vi "MC_7_24_12c_JW.vi"() -> ()   [LabVIEW 2011]
uses:
  <vilib>/Utility/file.llb/Read From Spreadsheet File (string).vi
  <vilib>/Utility/inputDevices.llb/keyboardAcquire.vi
  <vilib>/Utility/file.llb/Write To Spreadsheet File (DBL).vi
  <vilib>/Utility/file.llb/Write To Spreadsheet File (string).vi
  <vilib>/regexp/Match Regular Expression.xnode
panel:
  in  "Room Temp":dbl
  out "No Image 2":path=path "\\\\acad1\\physics/Jurchescu-group/JW-PD/Image Not Found.png"
  out "Save1 Array":string[][](array[string])
  out "XY Graph-Lin":cluster{dbl[], dbl[]}[](graph)
  out "Lin Vd":dbl
  out "Lin-Vg Array-Used":dbl[](array[numeric])
  out "Lin Id-Used":dbl[](array[numeric])
  out "Comments":string
  out "Folder Index":dbl caption="Length"
  out "Current \nRecord":string[](array[string])
  out "Transformer \nHeaders":string[](array[string])
  out "Current Device ID":string
  out "Column":string
  out "Row":string
  out "Rec: Concentration":dbl
  out "Rec: Solvent":string
  out "Rec: Method":string
  in  "?":T1(tab)
  out "Rec: Material":string
  in  "Treatment Concentration (mM):":dbl=30.0
  in  "Surface Treatment:":string
  in  "# Drops*:":dbl=inf
  in  "Solution Temp (C):":dbl=55.0
  in  "Relative Humidity (%):":dbl=nan
  in  "Room Temp (F):":dbl=nan
  in  "Time (s):":dbl=80.0
  out "Accel (RPM/s):":dbl
  in  "RPM:":dbl=1000.0
  in  "Wait Time (s):":dbl=10.0
  in  "Sample #:":dbl=1.0
  in  "Fabricator:":string="Jeremy"
  in  "Data File":path
  out "Data Folder":path
  in  "Image Folder":path
  out "Image File":path=path "D:/UserData/Desktop/Jeremy/WFU/Research/Programs/VI mods/Image Not Found.png"
  in  "Ramp (s):":dbl=3.0
  out "Calc: Off I-Sat":dbl caption="Off I-Sat" format="%#_4e"
  in  "Manuel-Dielectric":bool
  in  "Manuel-Length":bool
  out "Calc: VT-Lin":dbl
  out "New: VT-Lin":dbl
  out "Rec: VT-Lin":dbl caption="VT-Lin" format="%#_3g"
  out "Calc: Trap Density-STS":dbl format="%#_3e"
  out "New: Trap Density-STS":dbl format="%#_3e"
  out "Rec: Trap Density-STS":dbl caption="N-Sat (STS)" format="%#_3e"
  out "Calc: Trap Density-VT":dbl format="%#_3e"
  out "New: Trap Density-VT":dbl format="%#_3e"
  out "Rec: Trap Density-VT":dbl caption="N-Sat (VT)" format="%#_3e"
  out "Calc: Mobility-Lin":dbl format="%#_4e"
  out "New: Mobility-Lin":dbl format="%#_4e"
  out "Rec: Mobility-Lin":dbl caption="Mobility-Lin" format="%#_4e"
  out "Calc: Mobility-Sat":dbl format="%#_4e"
  out "Rec: Length":dbl caption="Length" format="%#_3g"
  out "Rec: Width":dbl caption="Width" format="%#_4g"
  out "Rec: Dielectric (d)":dbl caption="Dielectric (d)" format="%#_3g"
  out "XY Graph":cluster{dbl[], dbl[]}[](graph)
  in  "NumPts":dbl=5.0
  in  "Cancel Button":bool
  in  "Next Button":bool
  in  "Previous Button":bool
  in  "Up Button":bool
  in  "Down Button":bool
  out "Data Name:":string
  in  "Save Changes?":bool
  in  "New: Dielectric":dbl
  in  "New: Length":dbl
  in  "New: Width":dbl
  out "New: Mobility-Sat":dbl format="%#_4e"
  in  "Slide":dbl(slide) step=1.0 scale=-14.3..89.0 scale format="%#_1p"
  in  "Blank Button":bool
  in  "Zoom":i16(slide)=-3 scale=-5.0..5.0
  out "Image Out 2":T2(plugin-control)
  out "Image Out":T2(plugin-control)
  in  "Magnification":u16(ring) items=["5x", "10x", "20x", "50x", "80x"]
  out "Total Width":dbl
  out "Distances":dbl[](array[numeric])
  in  "Undo Button":bool
  in  "Remove Button":bool
  out "Rec: Mobility-Sat":dbl caption="Mobility-Sat" format="%#_4e"
  out "Index":string
  out "Image Name":string
  in  "Export":bool
  out "Calc: VT-Sat":dbl format="%#_3g"
  out "New: VT-Sat":dbl format="%#_3g"
  in  "Manual-Width":bool caption="Manual"
  out "XY Graph 2":cluster{dbl[], dbl[]}[](graph)
  in  "Next Button 2":bool
  in  "Previous Button 2":bool
  in  "Slide 2":dbl(slide) step=1.0 scale=-1.0..82.0 scale format="%#_1p"
  out "Calc: STS":dbl format="%#_3g"
  out "New: STS":dbl format="%#_3g"
  in  "NumPts 2":dbl=5.0 caption="NumPts"
  out "Rec: VT-Sat":dbl caption="VT-Sat" format="%#_3g"
  out "Rec: STS":dbl caption="STS-Sat" format="%#_3g"
  out "Rec: On/Off":dbl caption="On/Off-Sat" format="%#_4e"
  in  "Save Changes? 2":bool
  in  "Save Changes? 3":bool
  out "Date Recorded":string="Date Recorded" caption="Measured"
  out "Date Created":string caption="Fabricated"
  out "Rec: Temp":dbl caption="Sample Temp"
  out "New: Temp":dbl
  out "String":string
  in  "No Image":path=path "\\\\acad1\\physics/Jurchescu-group/JW-PD/Image Not Found.png"
  in  "Project":path=path "\\\\acad1\\physics/Jurchescu-group/JW-PD/Group Library/Origin Project Files/DeviceData_7_25a_JWW.opj"
  out "Index 2":dbl
  out "Sat Id-Log-Used":dbl[](array[numeric])
  out "Vg Array-Log-Used":dbl[](array[numeric])
  out "ROI Descriptor out":T3 {"Contours"."Type" items=["No Selection", "Point", "Line", "Rectangle", "Oval", "Polygon", "Freehand Region", "Annulus", "Unused2", "Unused3", "Broken Line", "Freehand Line", "Rotated Rectangle"]}
  out "ROI Descriptor":T3 {"Contours"."Type" items=["No Selection", "Point", "Line", "Rectangle", "Oval", "Polygon", "Freehand Region", "Annulus", "Unused2", "Unused3", "Broken Line", "Freehand Line", "Rotated Rectangle"]}
  out "Numeric 3":dbl
  out "Array 6":dbl[][](array[numeric])
  out "Cluster":T4
  out "Array 5":dbl[](array[numeric])
  out "Array 4":dbl[](array[numeric])
  out "Array 3":dbl[](array[numeric])
  out "Numeric 2":dbl
  out "Numeric":dbl
  out "Sat Id-Used":dbl[](array[numeric])
  out "Sat Vg Array-Used":dbl[](array[numeric])
  out "MobVi Index":dbl
  in  "Row Start":dbl=20.0
  # "Data Locations"
  # "Data Location"
  # "Image Location"
  # "Sample Properties"
  # "*     Inf = Full coverage\n   NaN = Unknown or Not Applicable"
  # "Recorded"
  # "Calculated"
  # "Re-Calculated"
  # "Manual"
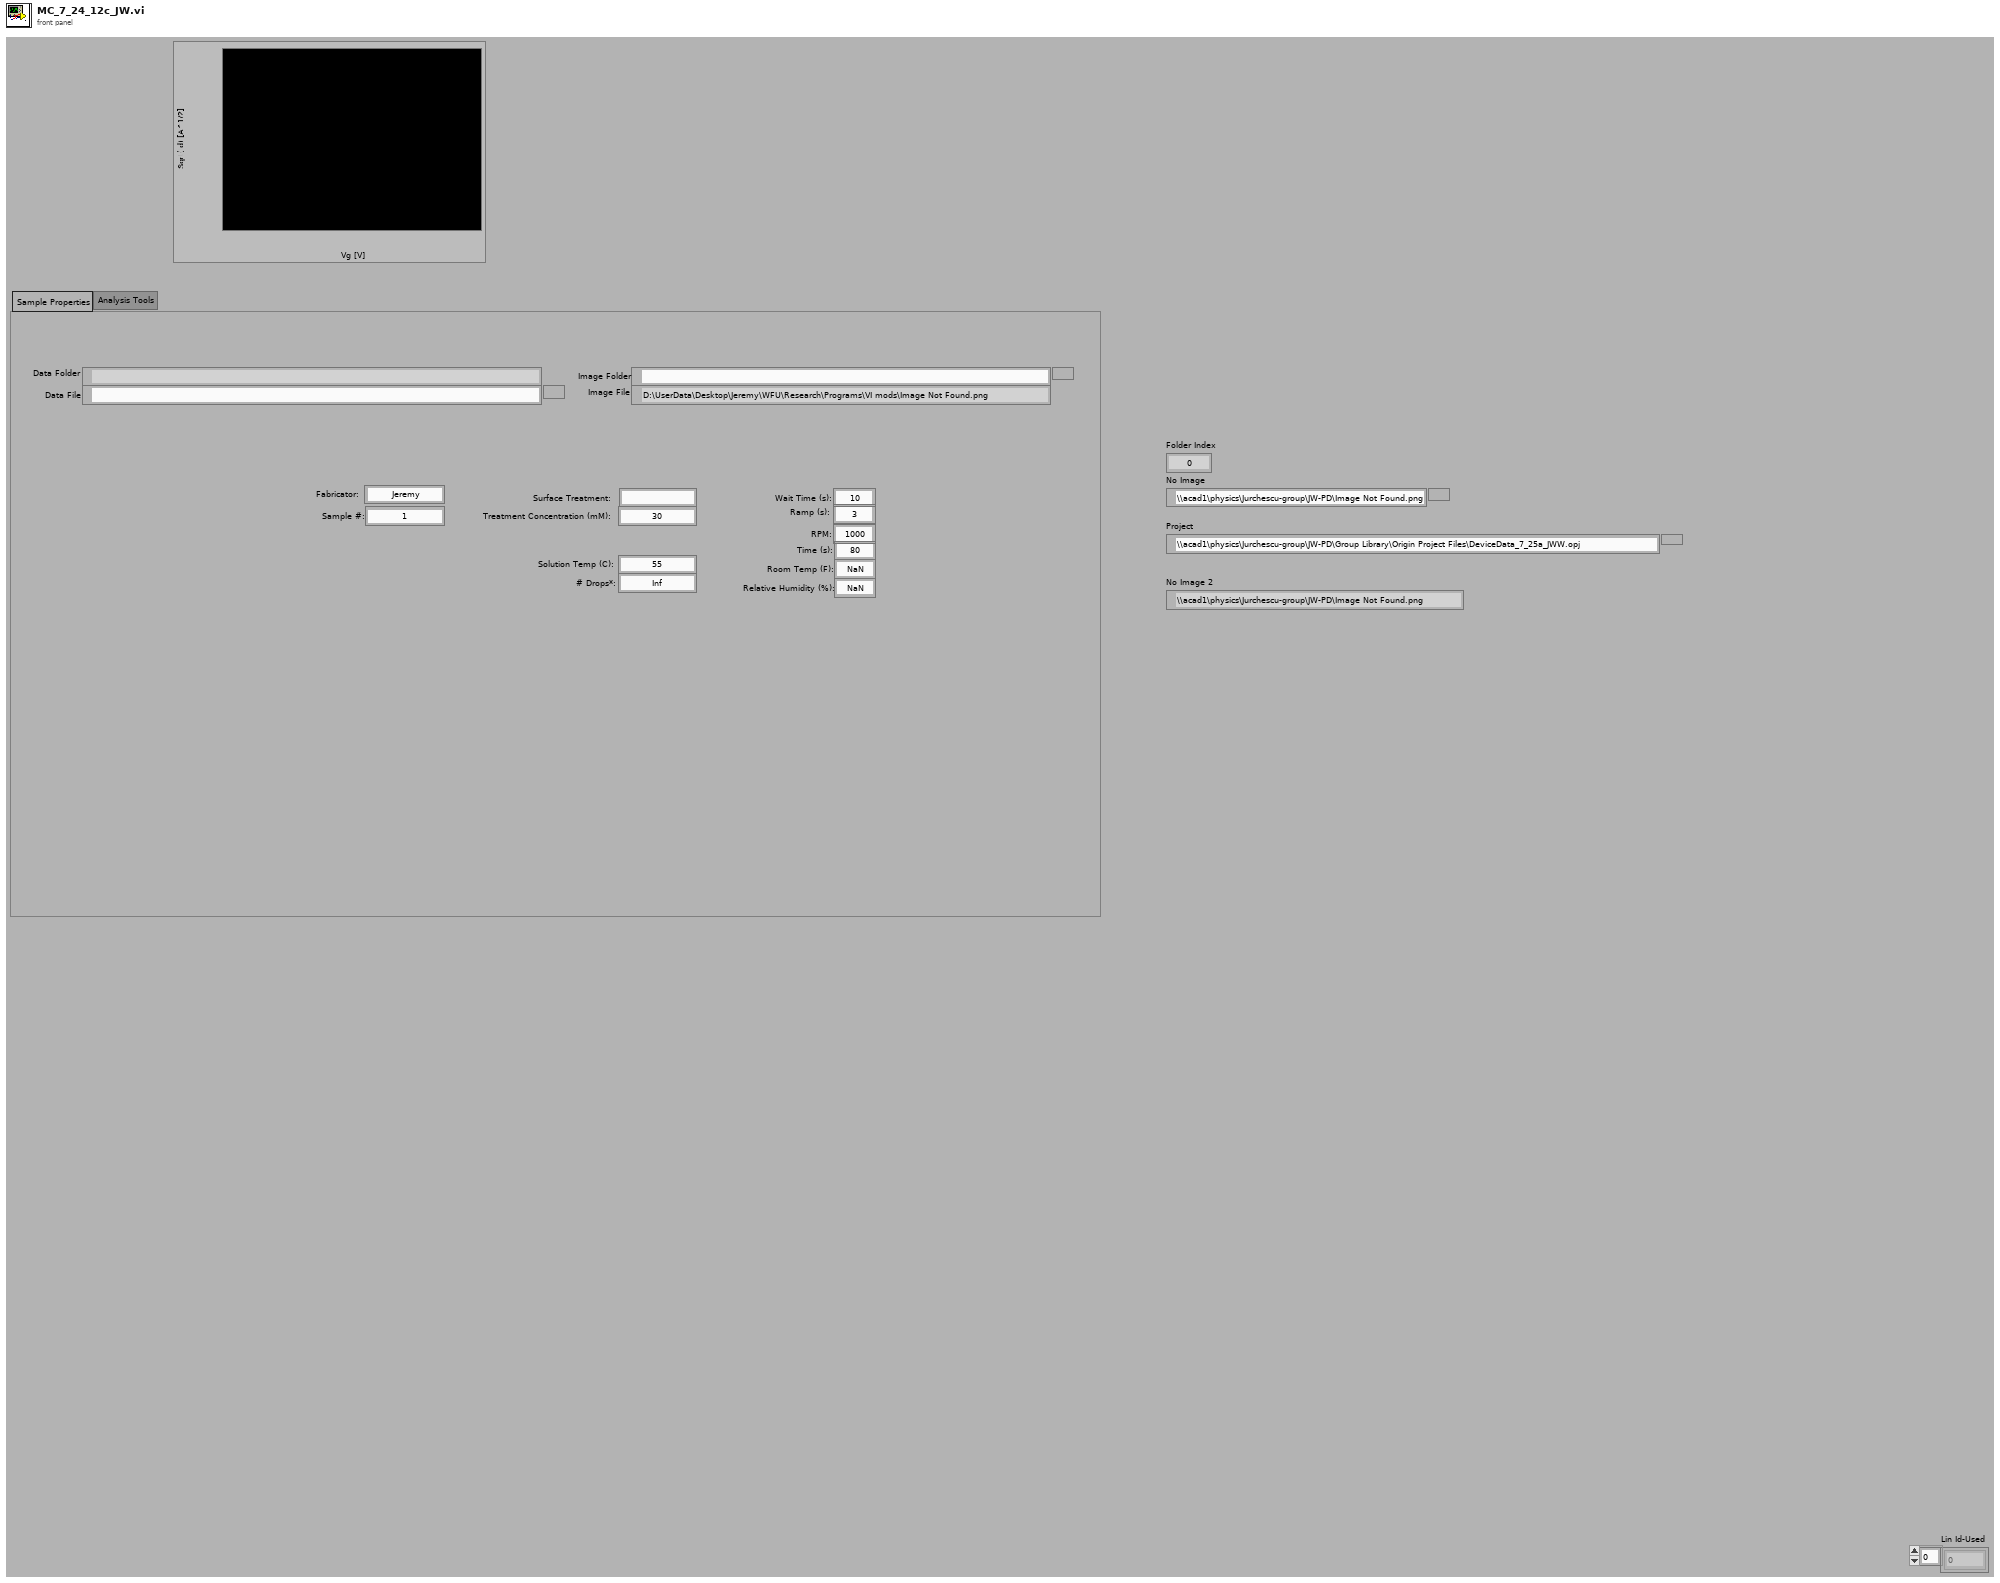
[diagram p1: front panel]
types:
  T1 = enum32{"Sample Properties", "Analysis Tools", "Current Database"}
  T2 = typedef "IMAQ Image.ctl" = refnum<image>
  T3 = typedef "ROI Descriptor" = cluster{"Global Rectangle":i32[], "Contours":cluster{"ID":enum32{"External", "Internal"}, "Type":u32, "Coordinates":i32[]}[]}
  T4 = cluster{"Numeric":dbl, "Numeric 2":dbl, "Numeric 3":dbl, "Numeric 4":dbl}
  T5 = cluster{"Mobility-Sat":dbl, "Moblitity-Lin":dbl, "On/Off":dbl, "Off Current":dbl, "Vt-Sat":dbl, "STS":dbl, "Trap Density-VT":dbl, "Trap Density-STS":dbl}
  T6 = cluster{"Date Recorded":string, "Index":string, "Length":dbl, "Width":dbl, "Sample Temp":dbl}
  T7 = cluster{"Date Created":string, "Material":string, "Solvent":string, "Concentration":dbl, "Method":string, "Dielectric (nm)":dbl, "Treatment":string, "Comments":string}
  T8 = cluster{"Mobility-Sat":dbl, "Vt-Sat":dbl, "Mobility-Lin":dbl, "Vt-Lin":dbl, "Off I-Sat":dbl, "On/Off I-Sat":dbl}
  T9 = cluster{"[0]":cluster{dbl[], dbl[]}, "[1]":cluster{dbl[], dbl[]}, "[2]":cluster{dbl[], dbl[]}, "[3]":cluster{dbl[], dbl[]}, "[4]":cluster{dbl[], dbl[]}, "[5]":cluster{dbl[], dbl[]}, "[6]":cluster{dbl[], dbl[]}, "[7]":cluster{dbl[], dbl[]}, "[8]":cluster{dbl[], dbl[]}}
  T10 = cluster{"Global Rectangle":i32[], "Contours":cluster{"Contour Type":u32, "ROI Type":u32, "Points":i32[]}[]}
  T11 = typedef "LVBoundsTypeDef.ctl" = cluster{"Width":u32, "Height":u32}
  T12 = enum16{"0", "1", "2", "3", "4", "5", "6", "7", "8", "9", "A", "B", "C", "D", "E", "F", "G", "H", "I", "J", "K", "L", "M", "N", "O", "P", "Q", "R", "S", "T", "U", "V", "W", "X", "Y", "Z", "F1", "F2", "F3", "F4", "F5", "F6", "F7", "F8", "F9", "F10", "F11", "F12", "F13", "F14", "F15", "ADD", "BACK", "BACKSLASH", "CAPITAL", "COMMA", "DECIMAL", "DELETE", "DIVIDE", "DOWN", "END", "EQUALS", "ESCAPE", "GRAVE (`)", "HOME", "INSERT", "LBRACKET", "LCONTROL", "LEFT", "L ALT", "LSHIFT", "LWIN", "MINUS", "MULTIPLY", "NEXT", "NUMLOCK", "NUMPAD_0", "NUMPAD_1", "NUMPAD_2", "NUMPAD_3", "NUMPAD_4", "NUMPAD_5", "NUMPAD_6", "NUMPAD_7", "NUMPAD_8", "NUMPAD_9", "PAUSE", "PERIOD", "PRIOR (PG UP)", "RBRACKET", "RCONTROL", "RETURN", "RIGHT", "R ALT", "RSHIFT", "RWIN", "SCROLL", "SEMICOLON", "SLASH", "SPACE", "SUBTRACT", "TAB", "UP", "ENTER (num pad)", "' (quote)"}[]
  T13 = enum16{"0", "1", "2", "3", "4", "5", "6", "7", "8", "9", "A", "B", "C", "D", "E", "F", "G", "H", "I", "J", "K", "L", "M", "N", "O", "P", "Q", "R", "S", "T", "U", "V", "W", "X", "Y", "Z", "F1", "F2", "F3", "F4", "F5", "F6", "F7", "F8", "F9", "F10", "F11", "F12", "F13", "F14", "F15", "ADD", "BACK", "BACKSLASH", "CAPITAL", "COMMA", "DECIMAL", "DELETE", "DIVIDE", "DOWN", "END", "EQUALS", "ESCAPE", "GRAVE (`)", "HOME", "INSERT", "LBRACKET", "LCONTROL", "LEFT", "L ALT", "LSHIFT", "LWIN", "MINUS", "MULTIPLY", "NEXT", "NUMLOCK", "NUMPAD_0", "NUMPAD_1", "NUMPAD_2", "NUMPAD_3", "NUMPAD_4", "NUMPAD_5", "NUMPAD_6", "NUMPAD_7", "NUMPAD_8", "NUMPAD_9", "PAUSE", "PERIOD", "PRIOR (PG UP)", "RBRACKET", "RCONTROL", "RETURN", "RIGHT", "R ALT", "RSHIFT", "RWIN", "SCROLL", "SEMICOLON", "SLASH", "SPACE", "SUBTRACT", "TAB", "UP", "ENTER (num pad)", "' (quote)"}
  T14 = cluster{"Contour Type":u32, "ROI Type":u32, "Points":i32[]}[]
  T15 = cluster{i32[], cluster{"Contour Type":u32, "ROI Type":u32, "Points":i32[]}[]}
  T16 = cluster{string, sgl, bool, bool, bool, bool, bool, bool, i32}
  T17 = cluster{i32, cluster{string, sgl, bool, bool, bool, bool, bool, bool, i32}, i32, i32}
  T18 = cluster{"Contour Type":u32, "ROI Type":u32, "Points":i32[]}
  T19 = cluster{"Points[0]":i32, "Points[1]":i32, "Points[2]":i32, "Points[3]":i32, "Points[4]":i32, "Points[5]":i32, "Points[6]":i32, "Points[7]":i32, "Points[8]":i32}
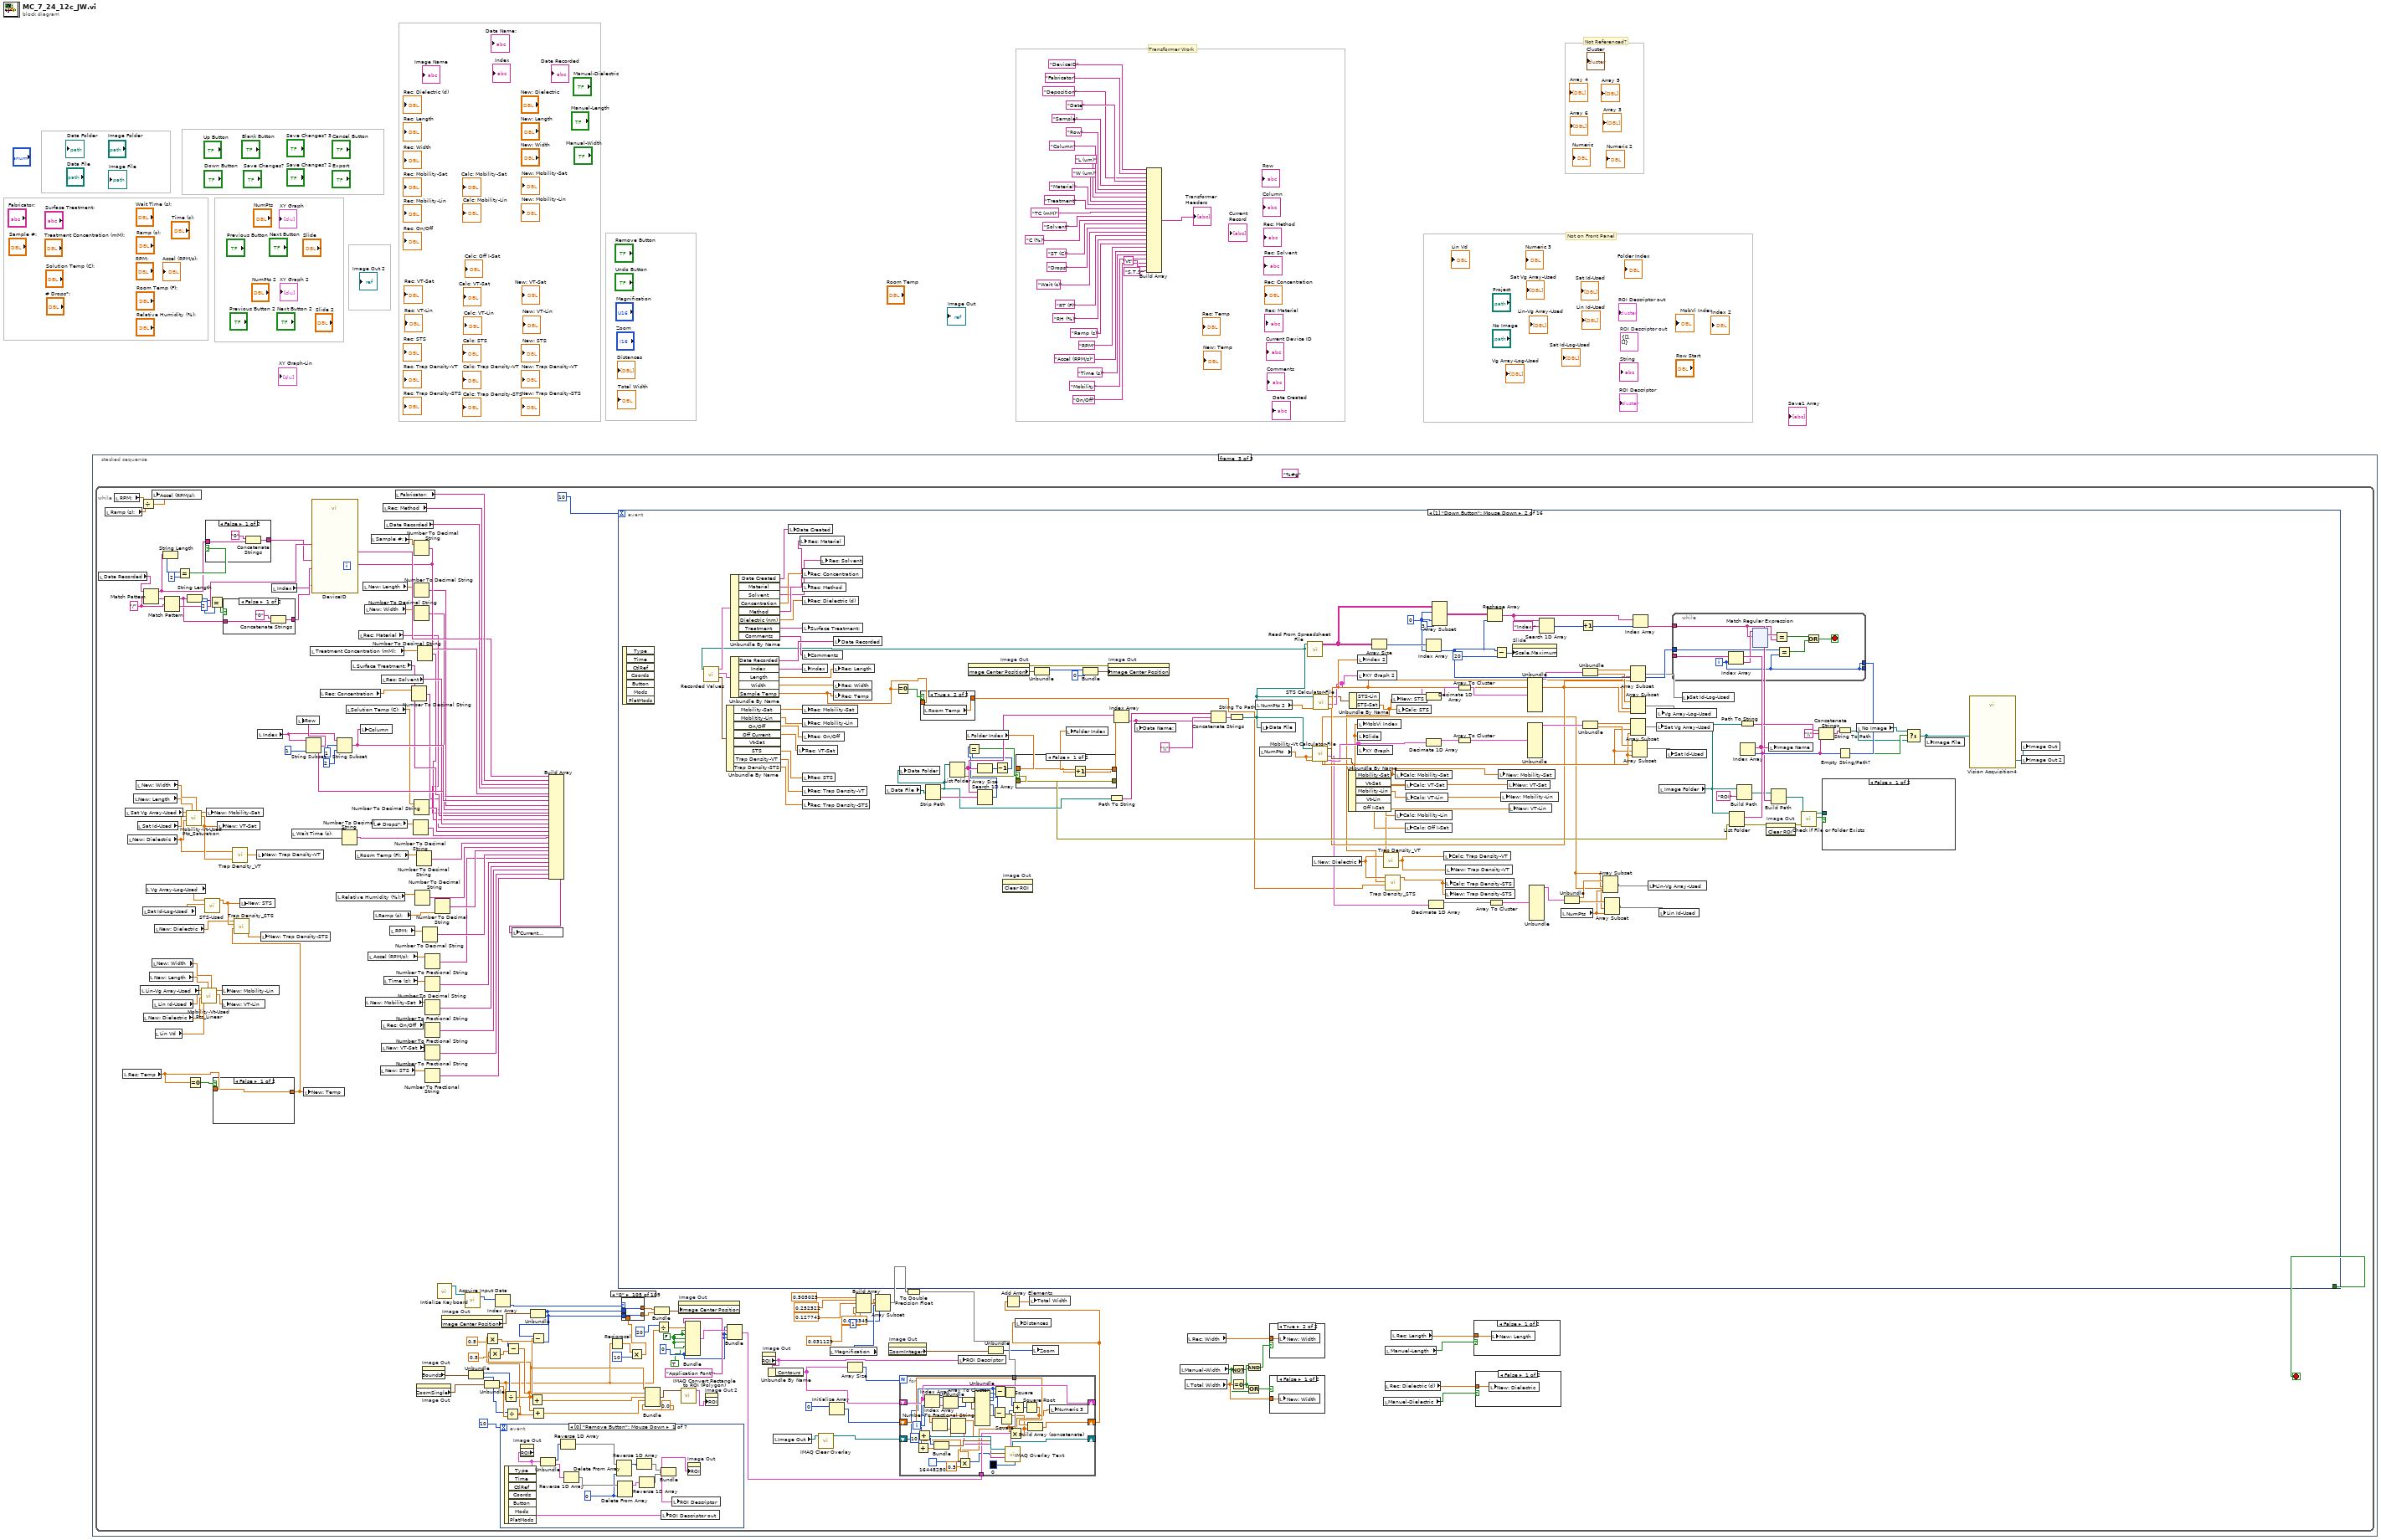
[diagram p0: block diagram]
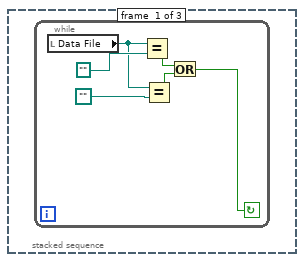
[diagram p2: hidden frame]
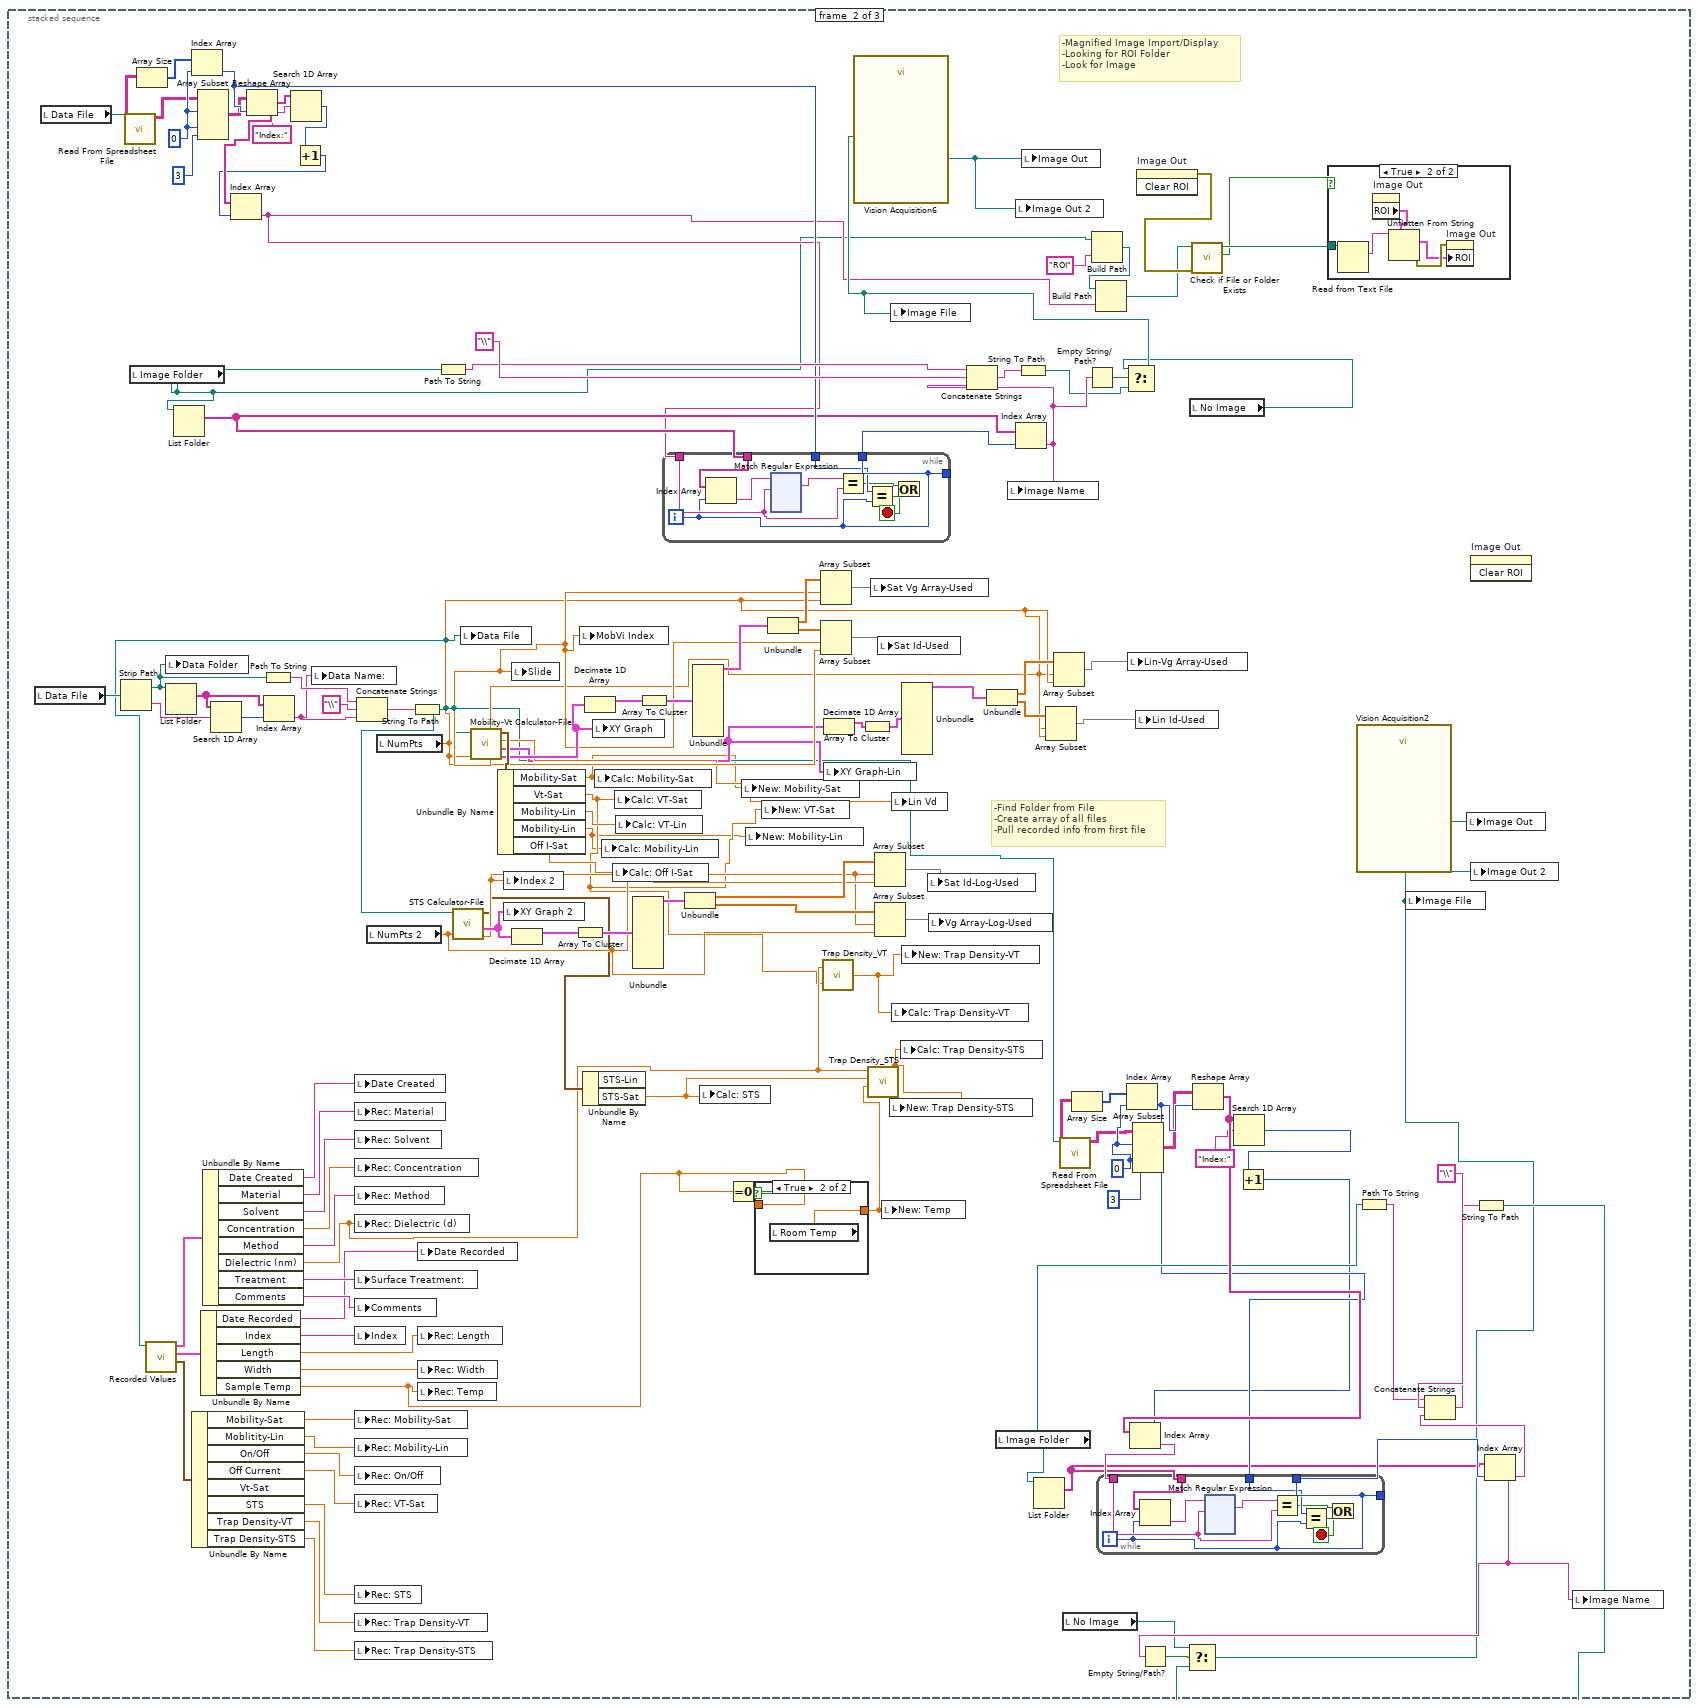
[diagram p3: hidden frame]
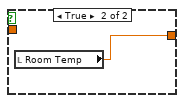
[diagram p6: hidden frame]
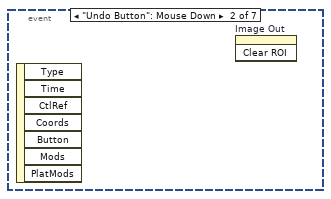
[diagram p13: hidden frame]
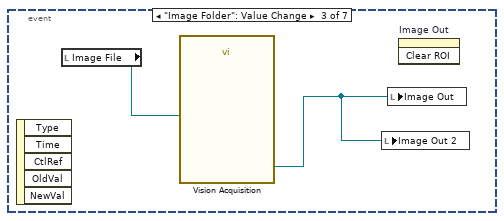
[diagram p14: hidden frame]
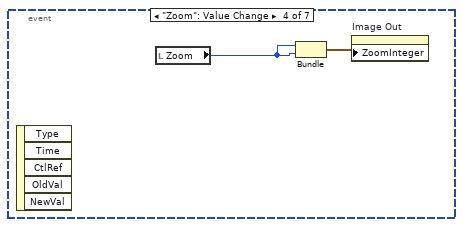
[diagram p15: hidden frame]
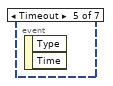
[diagram p16: hidden frame]
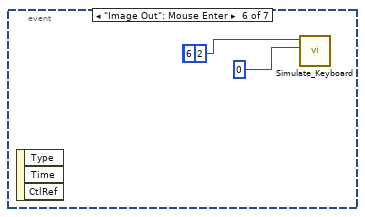
[diagram p17: hidden frame]
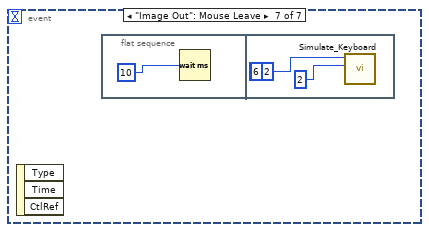
[diagram p18: hidden frame]
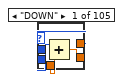
[diagram p19: hidden frame]
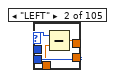
[diagram p20: hidden frame]
diagram:
  (unwired) T3 {"Global Rectangle"=[], "Contours"=[]}  # ROI Descriptor out
  # "Not Referenced?"
  # "Transformer Work"
  # "Not on Front Panel"
  n1 = stacked-sequence {
    frame #0 {
      n2 = while {
        stop <- w29 continue-if-true
        n3 = local read "Data File"() -> (w31:path)
        n4 = Equal?(x=w31, y=path "") -> (x = y?=w33:bool)
        n5 = Equal?(x=w31, y=path "") -> (x = y?=w32:bool)
        n6 = Or(x=w33, y=w32) -> (x .or. y?=w29:bool)
      }
    }
    frame #1 {
      w127 = 0
      w151 = 0
      # "-Find Folder from File\n-Create array of all files\n-Pull recorded info from first file"
      # "-Magnified Image Import/Display\n-Looking for ROI Folder\n-Look for Image"
      n7 = local read "Data File"() -> (w131:path)
      n8 = local read "Data File"() -> (w146:path)
      n9 = Strip Path(path=w131) -> (stripped path=w132:path, name=w118:string)
      n10 = call-poly <vilib>:"Read From Spreadsheet File.vi"("file path (dialog if empty)"=w146) -> ("all rows"=w149:string[][])  [unwired: 6 in, 4 out]
      n11 = local read "Image Folder"() -> (w88:path)
      n12 = Array Size(array=w149) -> (size(s)=w150:i32[])
      n13 = local write "Data Folder"(w132) -> ()
      n14 = List Folder(path=w132) -> (filenames=w122:string[])  [unwired: 3 in, 3 out]
      n15 = List Folder(path=w88) -> (filenames=w155:string[])  [unwired: 3 in, 3 out]
      n16 = Index Array(array=w150, index=w151) -> (element=w157:i32)
      n17 = Array Subset(array=w149, index (row)=w151, index (col)=w151, length (col)=3) -> (w148:string[][])  [unwired: 1 in]
      n18 = Search 1D Array(1D array=w122, element=w118) -> (index of element=w121:i32)  [unwired: 1 in]
      n19 = Reshape Array(w148, w157) -> (w162:string[])
      n20 = Path To String(path=w132) -> (string=w117:string)
      n21 = Index Array(array=w122, index=w121) -> (element=w87:string)
      n22 = Search 1D Array(1D array=w162, element="Index:") -> (index of element=w154:i32)  [unwired: 1 in]
      n23 = Increment(x=w154) -> (x+1=w153:i32)
      n24 = Index Array(array=w162, index=w153) -> (element=w89:string)
      n25 = local write "Data Name:"(w87) -> ()
      n26 = Concatenate Strings(w117, "\\", w87) -> (w119:string)
      n27 = local read "NumPts 2"() -> (w61:dbl)
      n28 = local read "NumPts"() -> (w52:dbl)
      n29 = String To Path(string=w119) -> (path=w44:path)
      n30 = call "Recorded Values.vi"("Path"=w44) -> ("Recorded Char"=w85:T5, "Recorded Prop"=w84:T6, "Fabrication Prop"=w86:T7)  [unwired: 8 in]
      n31 = Unbundle By Name(w85) -> ("Mobility-Sat"=w73:dbl, "Moblitity-Lin"=w72:dbl, "On/Off"=w71:dbl, "Off Current"=w70:dbl, "STS"=w69:dbl, "Trap Density-VT"=w68:dbl, "Trap Density-STS"=w67:dbl)  [unwired: 1 out]
      n32 = Unbundle By Name(w84) -> ("Date Recorded"=w77:string, "Index"=w76:string, "Length"=w75:dbl, "Width"=w74:dbl, "Sample Temp"=w43:dbl)
      n33 = Unbundle By Name(w86) -> ("Date Created"=w66:string, "Material"=w83:string, "Solvent"=w82:string, "Concentration"=w81:dbl, "Method"=w80:string, "Dielectric (nm)"=w39:dbl, "Treatment"=w79:string, "Comments"=w78:string)
      n34 = local write "Date Created"(w66) -> ()
      n35 = local write "Rec: Material"(w83) -> ()
      n36 = local write "Rec: Solvent"(w82) -> ()
      n37 = local write "Rec: Concentration"(w81) -> ()
      n38 = local write "Rec: Method"(w80) -> ()
      n39 = local write "Rec: Dielectric (d)"(w39) -> ()
      n40 = local write "Surface Treatment:"(w79) -> ()
      n41 = local write "Comments"(w78) -> ()
      n42 = local write "Index"(w76) -> ()
      n43 = local write "Rec: Mobility-Sat"(w73) -> ()
      n44 = local write "Rec: Mobility-Lin"(w72) -> ()
      n45 = local write "Rec: On/Off"(w71) -> ()
      n46 = local write "Rec: VT-Sat"(w70) -> ()
      n47 = local write "Rec: STS"(w69) -> ()
      n48 = local write "Rec: Trap Density-VT"(w68) -> ()
      n49 = local write "Rec: Trap Density-STS"(w67) -> ()
      n50 = local write "Date Recorded"(w77) -> ()
      n51 = local write "Rec: Length"(w75) -> ()
      n52 = local write "Rec: Width"(w74) -> ()
      n53 = local write "Rec: Temp"(w43) -> ()
      n54 = Path To String(path=w88) -> (string=w159:string)
      n55 = call "STS Calculator-File.vi"("NumPts"=w61, "Path"=w44) -> ("STS Index-Sat"=w59:dbl, "XY Graph-Sat"=w60:cluster{dbl[], dbl[]}[], "Ouput"=w58:cluster{"STS-Sat":dbl, "STS-Lin":dbl})  [unwired: 5 in, 2 out]
      n56 = local write "Data File"(w44) -> ()
      n57 = call "Mobility-Vt Calculator-File.vi"("NumPts"=w52, "Path"=w44) -> ("XY Graph-Sat"=w63:cluster{dbl[], dbl[]}[], "XY Graph-Lin"=w47:cluster{dbl[], dbl[]}[], "Lin Vd"=w48:dbl, "Output"=w64:T8, "Index-Sat"=w62:dbl, "Index-Lin"=w51:dbl)  [unwired: 4 in]
      n58 = Unbundle By Name(w64) -> ("Mobility-Sat"=w38:dbl, "Vt-Sat"=w37:dbl, "Mobility-Lin"=w65:dbl, "Mobility-Lin"=w36:dbl, "Off I-Sat"=w45:dbl)
      n59 = local write "Index 2"(w59) -> ()
      n60 = local write "XY Graph 2"(w60) -> ()
      n61 = local write "Slide"(w62) -> ()
      n62 = Decimate 1D Array(w60) -> (w109:cluster{dbl[], dbl[]}[])  [unwired: 1 out]
      n63 = Array To Cluster(array=w109) -> (cluster=w111:T9)
      n64 = local write "MobVi Index"(w62) -> ()
      n65 = Unbundle By Name(w58) -> ("STS-Sat"=w42:dbl)  [unwired: 1 out]
      n66 = Decimate 1D Array(w63) -> (w145:cluster{dbl[], dbl[]}[])  [unwired: 1 out]
      n67 = local write "XY Graph"(w63) -> ()
      n68 = local write "Calc: Mobility-Sat"(w38) -> ()
      n69 = local write "Calc: Mobility-Lin"(w36) -> ()
      n70 = local write "Calc: Off I-Sat"(w45) -> ()
      n71 = local write "Calc: VT-Sat"(w37) -> ()
      n72 = local write "Calc: VT-Lin"(w65) -> ()
      n73 = Unbundle(w111) -> ("[0]"=w110:cluster{dbl[], dbl[]})  [unwired: 8 out]
      n74 = Array To Cluster(array=w145) -> (cluster=w143:T9)
      n75 = while {
        tunnel: w155 -> [w297]
        tunnel: w89 -> [w295]
        tunnel: [w294] -> _
        tunnel: [w294] -> w156
        tunnel: w157 -> [w293]
        i -> [w294]
        stop <- w290 stop-if-true
        n76 = Index Array(array=w297, index=w294) -> (element=w298:string)
        n77 = xnode "Match Regular Expression"("input string"=w298, "regular expression"=w295) -> ("whole match"=w296:string)  [unwired: 4 in, 4 out]
        n78 = Equal?(x=w296, y=w295) -> (x = y?=w292:bool)
        n79 = Equal?(x=w293, y=w294) -> (x = y?=w291:bool)
        n80 = Or(x=w292, y=w291) -> (x .or. y?=w290:bool)
      }
      n81 = Unbundle(w110) -> (w107:dbl[], w106:dbl[])
      n82 = Unbundle(w143) -> ("[0]"=w144:cluster{dbl[], dbl[]})  [unwired: 8 out]
      n83 = local write "Calc: STS"(w42) -> ()
      n84 = Equal To 0?(x=w43) -> (x = 0?=w46:bool)
      n85 = local write "New: Mobility-Sat"(w38) -> ()
      n86 = local write "New: Mobility-Lin"(w36) -> ()
      n87 = case shown="True" w46 {
        tunnel: [w163 w164] -> w41
        tunnel: w43 -> [w163 _]
        frame False {
        }
        frame True {
          n88 = local read "Room Temp"() -> (w164:dbl)
        }
      }
      n89 = local write "New: VT-Sat"(w37) -> ()
      n90 = Unbundle(w144) -> (w108:dbl[], w112:dbl[])
      n91 = Array Subset(array=w108, index=w62, length=w52) -> (w115:dbl[])
      n92 = Array Subset(array=w112, index=w62, length=w52) -> (w116:dbl[])
      n93 = call "Trap Density_VT.vi"("VT"=w37, "Dielectric"=w39) -> ("Trap Density-VT"=w35:dbl)
      n94 = Decimate 1D Array(w47) -> (w57:cluster{dbl[], dbl[]}[])  [unwired: 1 out]
      n95 = local write "XY Graph-Lin"(w47) -> ()
      n96 = Array To Cluster(array=w57) -> (cluster=w56:T9)
      n97 = call "Trap Density_STS.vi"("Temp (T) [K]"=w41, "S.T.S. (S)"=w42, "Dielectric"=w39) -> ("Trap Density (N)"=w40:dbl)  [unwired: 8 in]
      n98 = local write "Sat Vg Array-Used"(w115) -> ()
      n99 = Array Subset(array=w107, index=w59, length=w61) -> (w114:dbl[])
      n100 = Array Subset(array=w106, index=w59, length=w61) -> (w113:dbl[])
      n101 = local write "Sat Id-Used"(w116) -> ()
      n102 = local write "New: Temp"(w41) -> ()
      n103 = local write "New: Trap Density-STS"(w40) -> ()
      n104 = local write "Lin Vd"(w48) -> ()
      n105 = local write "Calc: Trap Density-VT"(w35) -> ()
      n106 = local write "Calc: Trap Density-STS"(w40) -> ()
      n107 = Unbundle(w56) -> ("[0]"=w55:cluster{dbl[], dbl[]})  [unwired: 8 out]
      n108 = local write "New: Trap Density-VT"(w35) -> ()
      n109 = local write "Sat Id-Log-Used"(w114) -> ()
      n110 = local write "Vg Array-Log-Used"(w113) -> ()
      n111 = Unbundle(w55) -> (w54:dbl[], w53:dbl[])
      n112 = local read "Image Folder"() -> (w138:path)
      n113 = Index Array(array=w155, index=w156) -> (element=w105:string)
      n114 = Concatenate Strings(w159, "\\", w105) -> (w160:string)
      n115 = local write "Image Name"(w105) -> ()
      n116 = String To Path(string=w160) -> (path=w103:path)
      n117 = List Folder(path=w138) -> (filenames=w134:string[])  [unwired: 3 in, 3 out]
      n118 = Array Subset(array=w53, index=w51, length=w52) -> (w49:dbl[])
      n119 = Array Subset(array=w54, index=w51, length=w52) -> (w50:dbl[])
      n120 = call-poly <vilib>:"Read From Spreadsheet File.vi"("file path (dialog if empty)"=w44) -> ("all rows"=w125:string[][])  [unwired: 6 in, 4 out]
      n121 = local read "No Image"() -> (w97:path)
      n122 = Array Size(array=w125) -> (size(s)=w126:i32[])
      n123 = Empty String/Path?(string/path=w105) -> (empty?=w104:bool)
      n124 = Build Path(base path=w88, name or relative path="ROI") -> (appended path=w91:path)
      n125 = Build Path(base path=w91, name or relative path=w89) -> (appended path=w90:path)
      n126 = Index Array(array=w126, index=w127) -> (element=w137:i32)
      n127 = local write "Lin-Vg Array-Used"(w50) -> ()
      n128 = Array Subset(array=w125, index (row)=w127, index (col)=w127, length (col)=3) -> (w124:string[][])  [unwired: 1 in]
      n129 = local write "Lin Id-Used"(w49) -> ()
      n130 = invoke on="Image Out" class="ImageControl" method="Clear ROI"() -> (error out=w95:errorcluster)  [unwired: 3 in, 2 out]
      n131 = local read "No Image"() -> (w96:path)
      n132 = Select(t=w96, s=w104, f=w103) -> (s? t:f=w102:path)
      n133 = call "Vision Acquisition6"("Image Path"=w102) -> ("Image Out"=w158:T2)  [unwired: 25 in, 1 out]
      n134 = local write "Image File"(w102) -> ()
      n135 = local write "Image Out 2"(w158) -> ()
      n136 = local write "Image Out"(w158) -> ()
      n137 = call <vilib>:"Check if File or Folder Exists.vi"("error in (no error)"=w95, "path"=w90) -> ("file or folder exists?"=w93:bool, "dup path"=w94:path)  [unwired: 7 in, 1 out]
      n138 = Reshape Array(w124, w137) -> (w142:string[])
      n139 = Search 1D Array(1D array=w142, element="Index:") -> (index of element=w130:i32)  [unwired: 1 in]
      n140 = Increment(x=w130) -> (x+1=w129:i32)
      n141 = Index Array(array=w142, index=w129) -> (element=w135:string)
      n142 = while {
        tunnel: w134 -> [w177]
        tunnel: w135 -> [w175]
        tunnel: [w174] -> _
        tunnel: [w174] -> w136
        tunnel: w137 -> [w173]
        i -> [w174]
        stop <- w170 stop-if-true
        n143 = Index Array(array=w177, index=w174) -> (element=w178:string)
        n144 = xnode "Match Regular Expression"("input string"=w178, "regular expression"=w175) -> ("whole match"=w176:string)  [unwired: 4 in, 4 out]
        n145 = Equal?(x=w176, y=w175) -> (x = y?=w172:bool)
        n146 = Equal?(x=w173, y=w174) -> (x = y?=w171:bool)
        n147 = Or(x=w172, y=w171) -> (x .or. y?=w170:bool)
      }
      n148 = case shown="True" w93 {
        tunnel: w94 -> [_ w165]
        frame False {
        }
        frame True {
          n149 = Read from Text File(file (use dialog)=w165) -> (text=w169:string)  [unwired: 3 in, 3 out]
          n150 = property on="Image Out" class="ImageControl"() -> ("ROI"=w166:T10)  [unwired: 2 in, 2 out]
          n151 = Unflatten From String(type=w166, binary string=w169) -> (value=w167:T10, error out=w168:errorcluster)  [unwired: 3 in, 1 out]
          n152 = property on="Image Out" class="ImageControl"(error in=w168, "ROI"=w167) -> ()  [unwired: 1 in, 2 out]
        }
      }
      n153 = Path To String(path=w138) -> (string=w139:string)
      n154 = invoke on="Image Out" class="ImageControl" method="Clear ROI"() -> ()  [unwired: 3 in, 3 out]
      n155 = Index Array(array=w134, index=w136) -> (element=w100:string)
      n156 = Empty String/Path?(string/path=w100) -> (empty?=w101:bool)
      n157 = Concatenate Strings(w139, "\\", w100) -> (w140:string)
      n158 = String To Path(string=w140) -> (path=w99:path)
      n159 = Select(t=w97, s=w101, f=w99) -> (s? t:f=w98:path)
      n160 = call "Vision Acquisition2"("Image Path"=w98) -> ("Image Out"=w133:T2)  [unwired: 25 in, 1 out]
      n161 = local write "Image File"(w98) -> ()
      n162 = local write "Image Out"(w133) -> ()
      n163 = local write "Image Out 2"(w133) -> ()
      n164 = local write "Image Name"(w100) -> ()
    }
    frame #2 {
      (unwired) "%#g"
      n165 = while {
        stop <- w575 stop-if-true
        w471 = "/"
        w525 = FALSE
        w523 = 0
        n166 = local read "Date Recorded"() -> (w474:string)
        n167 = local read "Ramp (s):"() -> (w441:dbl)
        n168 = local read "RPM:"() -> (w442:dbl)
        n169 = local read "Rec: Temp"() -> (w413:dbl)
        n170 = local read "Sat Vg Array-Used"() -> (w430:dbl[])
        n171 = local read "New: Dielectric"() -> (w415:dbl)
        n172 = local read "New: Length"() -> (w431:dbl)
        n173 = local read "New: Width"() -> (w433:dbl)
        n174 = local read "Sat Id-Used"() -> (w429:dbl[])
        n175 = local read "Lin-Vg Array-Used"() -> (w424:dbl[])
        n176 = Divide(x=w442, y=w441) -> (x/y=w440:dbl)
        n177 = local read "Sat Id-Log-Used"() -> (w428:dbl[])
        n178 = local read "New: Dielectric"() -> (w421:dbl)
        n179 = Match Pattern(string=w474, regular expression=w471) -> (before substring=w465:string, after substring=w472:string)  [unwired: 1 in, 2 out]
        n180 = local read "Vg Array-Log-Used"() -> (w427:dbl[])
        n181 = local read "New: Length"() -> (w423:dbl)
        n182 = local write "Accel (RPM/s):"(w440) -> ()
        n183 = local read "New: Width"() -> (w420:dbl)
        n184 = local read "Lin Id-Used"() -> (w425:dbl[])
        n185 = local read "New: Dielectric"() -> (w417:dbl)
        n186 = local read "Lin Vd"() -> (w419:dbl)
        n187 = String Length(string=w465) -> (length=w468:i32)
        n188 = Match Pattern(string=w472, regular expression=w471) -> (before substring=w459:string, after substring=w470:string)  [unwired: 1 in, 2 out]
        n189 = Equal?(x=w468, y=2) -> (x = y?=w466:bool)
        n190 = call "Mobility-Vt-Used Pts_Saturation.vi"("Width"=w433, "Length"=w431, "Dielectric (d)"=w415, "Sat Id Used"=w429, "Vg Used"=w430) -> ("Vt"=w416:dbl, "Mobility"=w432:dbl)  [unwired: 4 in, 1 out]
        n191 = String Length(string=w459) -> (length=w461:i32)
        n192 = Equal To 0?(x=w413) -> (x = 0?=w412:bool)
        n193 = call "Mobility-Vt-Used Pts_Linear.vi"("Width"=w420, "Length"=w423, "Vd"=w419, "Dielectric (d)"=w421, "Sat Id Used"=w425, "Vg Used"=w424) -> ("Vt"=w426:dbl, "Mobility"=w422:dbl)  [unwired: 3 in, 1 out]
        n194 = call "STS-Used.vi"("Id Used"=w428, "Vg-Used"=w427) -> ("STS"=w418:dbl)  [unwired: 9 in]
        n195 = case shown="False" w466 {
          tunnel: w465 -> [w585 w587]
          tunnel: [w584 w587] -> w464
          frame False {
            n196 = Concatenate Strings("0", w585) -> (w584:string)
          }
          frame True {
          }
        }
        n197 = local write "New: Mobility-Sat"(w432) -> ()
        n198 = Equal?(x=w461, y=2) -> (x = y?=w463:bool)
        n199 = case shown="False" w412 {
          tunnel: [w576 w577] -> w410
          tunnel: w413 -> [w576 _]
          frame False {
          }
          frame True {
            n200 = local read "Room Temp"() -> (w577:dbl)
          }
        }
        n201 = local write "New: VT-Sat"(w416) -> ()
        n202 = local write "New: Mobility-Lin"(w422) -> ()
        n203 = local write "New: VT-Lin"(w426) -> ()
        n204 = case shown="False" w463 {
          tunnel: w459 -> [w581 w583]
          tunnel: [w580 w583] -> w460
          frame False {
            n205 = Concatenate Strings("0", w581) -> (w580:string)
          }
          frame True {
          }
        }
        n206 = call "Trap Density_VT.vi"("VT"=w416, "Dielectric"=w415) -> ("Trap Density-VT"=w414:dbl)
        n207 = call "Trap Density_STS.vi"("Temp (T) [K]"=w410, "S.T.S. (S)"=w418, "Dielectric"=w417) -> ("Trap Density (N)"=w411:dbl)  [unwired: 8 in]
        n208 = local write "New: STS"(w418) -> ()
        n209 = local write "New: Trap Density-VT"(w414) -> ()
        n210 = local read "Index"() -> (w444:string)
        n211 = local write "New: Trap Density-STS"(w411) -> ()
        n212 = local read "Index"() -> (w458:string)
        n213 = local read "Wait Time (s):"() -> (w504:dbl)
        n214 = local write "New: Temp"(w410) -> ()
        n215 = String Subset(string=w444, length (rest)=1) -> (substring=w499:string)  [unwired: 1 in]
        n216 = local write "Row"(w499) -> ()
        n217 = local read "Treatment Concentration (mM):"() -> (w452:dbl)
        n218 = local read "Rec: Concentration"() -> (w439:dbl)
        n219 = local read "Relative Humidity (%):"() -> (w449:dbl)
        n220 = String Subset(string=w444, offset (0)=1, length (rest)=2) -> (substring=w500:string)
        n221 = Number To Decimal String(number=w504) -> (decimal integer string=w505:string)  [unwired: 1 in]
        n222 = local read "Solution Temp (C):"() -> (w493:dbl)
        n223 = local read "Surface Treatment:"() -> (w451:string)
        n224 = local read "Room Temp (F):"() -> (w497:dbl)
        n225 = local read "Rec: Material"() -> (w447:string)
        n226 = local write "Column"(w500) -> ()
        n227 = local read "New: Length"() -> (w457:dbl)
        n228 = local read "New: Width"() -> (w456:dbl)
        n229 = local read "New: Mobility-Sat"() -> (w486:dbl)
        n230 = local read "Accel (RPM/s):"() -> (w484:dbl)
        n231 = local read "Sample #:"() -> (w476:dbl)
        n232 = local read "# Drops*:"() -> (w494:dbl)
        n233 = local read "Ramp (s):"() -> (w502:dbl)
        n234 = local read "New: STS"() -> (w478:dbl)
        n235 = local read "Rec: Solvent"() -> (w453:string)
        n236 = local read "New: VT-Sat"() -> (w480:dbl)
        n237 = local read "Rec: On/Off"() -> (w482:dbl)
        n238 = local read "Rec: Method"() -> (w477:string)
        n239 = local read "Time (s):"() -> (w489:dbl)
        n240 = local read "Date Recorded"() -> (w473:string)
        n241 = local read "RPM:"() -> (w490:dbl)
        n242 = local read "Fabricator:"() -> (w498:string)
        n243 = Number To Decimal String(number=w439) -> (decimal integer string=w438:string)  [unwired: 1 in]
        n244 = Number To Decimal String(number=w494) -> (decimal integer string=w495:string)  [unwired: 1 in]
        n245 = Number To Decimal String(number=w476) -> (decimal integer string=w469:string)  [unwired: 1 in]
        n246 = call "DeviceID"("Sample"=w469, "Year"=w470, "Month"=w464, "Day"=w460, "Index"=w458) -> ("Result"=w475:string)  [unwired: 9 in, 1 out]
        n247 = Number To Decimal String(number=w457) -> (decimal integer string=w455:string)  [unwired: 1 in]
        n248 = Number To Decimal String(number=w456) -> (decimal integer string=w454:string)  [unwired: 1 in]
        n249 = Number To Decimal String(number=w493) -> (decimal integer string=w492:string)  [unwired: 1 in]
        n250 = Number To Decimal String(number=w449) -> (decimal integer string=w448:string)  [unwired: 1 in]
        n251 = Number To Decimal String(number=w497) -> (decimal integer string=w496:string)  [unwired: 1 in]
        n252 = property on="Image Out" class="ImageControl"() -> ("ZoomSingle"=w543:cluster{"X":sgl, "Y":sgl})  [unwired: 2 in, 2 out]
        n253 = Number To Decimal String(number=w452) -> (decimal integer string=w450:string)  [unwired: 1 in]
        n254 = property on="Image Out" class="ImageControl"() -> ("Bounds"=w544:T11)  [unwired: 2 in, 2 out]
        n255 = Number To Decimal String(number=w490) -> (decimal integer string=w491:string)  [unwired: 1 in]
        n256 = Number To Fractional String(number=w484) -> (F-format string=w485:string)  [unwired: 3 in]
        n257 = Number To Decimal String(number=w489) -> (decimal integer string=w488:string)  [unwired: 1 in]
        n258 = Number To Fractional String(number=w486) -> (F-format string=w487:string)  [unwired: 3 in]
        n259 = Number To Fractional String(number=w482) -> (F-format string=w483:string)  [unwired: 3 in]
        n260 = Number To Fractional String(number=w480) -> (F-format string=w481:string)  [unwired: 3 in]
        n261 = Number To Fractional String(number=w478) -> (F-format string=w479:string)  [unwired: 3 in]
        n262 = Number To Decimal String(number=w502) -> (decimal integer string=w503:string)  [unwired: 1 in]
        n263 = call <vilib>:"Intialize Keyboard.vi"() -> ("device ID"=w555:refnum<k1>)  [unwired: 10 in, 1 out]
        n264 = property on="Image Out" class="ImageControl"() -> ("Image Center Position"=w550:cluster{"X":u32, "Y":u32})  [unwired: 2 in, 2 out]
        n265 = call-poly <vilib>:"Acquire Input Data.vi"("device ID"=w555) -> ("keys pressed"=w554:T12)  [unwired: 16 in, 2 out]
        n266 = Unbundle(w544) -> ("Width"=w541:u32, "Height"=w540:u32)
        n267 = Unbundle(w543) -> ("X"=w518:sgl, "Y"=w542:sgl)
        n268 = Index Array(array=w554) -> (element=w558:T13)  [unwired: 1 in]
        n269 = event shown="[0] \"Remove Button\": Mouse Down" {
          selector: _ -> [_ _ _ _ _ _ _]
          dyn-events: _ -> [_ _ _ _ _ _ _]
          timeout: 10 -> [_ _ _ _ _ _ _]
          event "Remove Button": Mouse Down {
            w592 = 0
            n270 = event-data() -> ()  [unwired: 1 in, 7 out]
            n271 = property on="Image Out" class="ImageControl"() -> ("ROI"=w590:T10)  [unwired: 2 in, 2 out]
            n272 = Unbundle(w590) -> ("Global Rectangle"=w593:i32[], "Contours"=w595:T14)
            n273 = Reverse 1D Array(array=w593) -> (reversed array=w594:i32[])
            n274 = Reverse 1D Array(array=w595) -> (reversed array=w596:T14)
            n275 = Delete From Array(array=w594, index=w592) -> (array with subset deleted=w597:i32[])  [unwired: 1 in, 1 out]
            n276 = Delete From Array(array=w596, index=w592) -> (array with subset deleted=w598:T14)  [unwired: 1 in, 1 out]
            n277 = Reverse 1D Array(array=w597) -> (reversed array=w599:i32[])
            n278 = Reverse 1D Array(array=w598) -> (reversed array=w600:T14)
            n279 = Bundle(w599, w600) -> (w591:T15)  [unwired: 1 in]
            n280 = local write "ROI Descriptor out"(w590) -> ()
            n281 = local write "ROI Descriptor"(w591) -> ()
            n282 = property on="Image Out" class="ImageControl"("ROI"=w591) -> ()  [unwired: 2 in, 2 out]
          }
          event "Undo Button": Mouse Down {
            n283 = event-data() -> ()  [unwired: 1 in, 7 out]
            n284 = invoke on="Image Out" class="ImageControl" method="Clear ROI"() -> ()  [unwired: 3 in, 3 out]
          }
          event "Image Folder": Value Change {
            n285 = event-data() -> ()  [unwired: 1 in, 5 out]
            n286 = local read "Image File"() -> (w602:path)
            n287 = call "Vision Acquisition"("Image Path"=w602) -> ("Image Out"=w601:T2)  [unwired: 25 in, 1 out]
            n288 = local write "Image Out 2"(w601) -> ()
            n289 = local write "Image Out"(w601) -> ()
            n290 = invoke on="Image Out" class="ImageControl" method="Clear ROI"() -> ()  [unwired: 3 in, 3 out]
          }
          event "Zoom": Value Change {
            n291 = event-data() -> ()  [unwired: 1 in, 5 out]
            n292 = local read "Zoom"() -> (w603:i16)
            n293 = Bundle("Zoom"=w603, "Zoom"=w603) -> (w604:cluster{"Zoom":i16, "Zoom":i16})  [unwired: 1 in]
            n294 = property on="Image Out" class="ImageControl"("ZoomInteger"=w604) -> ()  [unwired: 2 in, 2 out]
          }
          event Timeout {
            n295 = event-data() -> ()  [unwired: 1 in, 2 out]
          }
          event "Image Out": Mouse Enter {
            (unwired) 6
            n296 = event-data() -> ()  [unwired: 1 in, 3 out]
            n297 = call "Simulate_Keyboard.vi"("Action"=0, "Virtual Key"=162) -> ()  [unwired: 7 in, 1 out]
          }
          event "Image Out": Mouse Leave {
            n298 = event-data() -> ()  [unwired: 1 in, 3 out]
            n299 = flat-sequence {
              frame #0 {
                n300 = Wait (ms)(milliseconds to wait=10) -> ()  [unwired: 1 out]
              }
              frame #1 {
                (unwired) 6
                n301 = call "Simulate_Keyboard.vi"("Action"=2, "Virtual Key"=162) -> ()  [unwired: 7 in, 1 out]
              }
            }
          }
        }
        n302 = Divide(x=w541, y=w518) -> (x/y=w531:sgl)
        n303 = Multiply(x=w531, y=0.5) -> (x*y=w537:dbl)
        n304 = Divide(x=w540, y=w542) -> (x/y=w530:sgl)
        n305 = Multiply(x=w530, y=0.5) -> (x*y=w536:dbl)
        n306 = Unbundle(w550) -> ("X"=w532:u32, "Y"=w533:u32)
        n307 = Subtract(x=w533, y=w536) -> (x-y=w534:dbl)
        n308 = Subtract(x=w532, y=w537) -> (x-y=w535:dbl)
        n309 = Add(x=w535, y=w531) -> (x+y=w549:dbl)
        n310 = Add(x=w534, y=w530) -> (x+y=w548:dbl)
        n311 = Build Array(w475, w498, w477, w473, w469, w499, w500, w455, w454, w447, w451, w450, w453, w438, w492, w495, w505, w496, w448, w503, w491, w485, w488, w487, w483, w481, w479) -> (w501:string[])
        n312 = local write "Current \nRecord"(w501) -> ()
        n313 = Reciprocal(x=w518) -> (1/x=w517:sgl)
        n314 = event shown="[1] \"Down Button\": Mouse Down" {
          selector: _ -> [_ _ _ _ _ _ _ _ _ _ _ _ _ _ _ _]
          dyn-events: _ -> [_ _ _ _ _ _ _ _ _ _ _ _ _ _ _ _]
          timeout: 10 -> [_ _ _ _ _ _ _ _ _ _ _ _ _ _ _ _]
          tunnel: [_ _ _ _ _ _ _ _ _ _ _ _ _ TRUE _ TRUE] -> w575
          event Timeout {
            n315 = event-data() -> ()  [unwired: 1 in, 2 out]
          }
          event "Down Button": Mouse Down {
            w942 = 0
            n316 = event-data() -> ()  [unwired: 1 in, 7 out]
            n317 = local read "Data File"() -> (w947:path)
            n318 = Strip Path(path=w947) -> (stripped path=w938:path, name=w956:string)
            n319 = local write "Data Folder"(w938) -> ()
            n320 = List Folder(path=w938) -> (filenames=w952:string[], error out=w892:errorcluster)  [unwired: 3 in, 2 out]
            n321 = local read "Folder Index"() -> (w894:dbl)
            n322 = property on="Image Out" class="ImageControl"() -> (error out=w895:errorcluster, "Image Center Position"=w899:cluster{"X":u32, "Y":u32})  [unwired: 2 in, 1 out]
            n323 = Array Size(array=w952) -> (size(s)=w948:i32)
            n324 = Search 1D Array(1D array=w952, element=w956) -> (index of element=w949:i32)  [unwired: 1 in]
            n325 = Decrement(x=w948) -> (x-1=w950:i32)
            n326 = Equal?(x=w949, y=w950) -> (x = y?=w951:bool)
            n327 = invoke on="Image Out" class="ImageControl" method="Clear ROI"() -> ()  [unwired: 3 in, 3 out]
            n328 = case shown="False" w951 {
              tunnel: w894 -> [w1109 _]
              tunnel: [w1108 0] -> w893
              tunnel: w892 -> [w1107 w1110]
              tunnel: [w1107 w1110] -> w891
              frame False {
                n329 = Increment(x=w1109) -> (x+1=w1108:dbl)
              }
              frame True {
              }
            }
            n330 = Unbundle(w899) -> ("X"=w897:u32)  [unwired: 1 out]
            n331 = local write "Folder Index"(w893) -> ()
            n332 = Bundle("X"=w897, 0) -> (w898:cluster{"X":u32, i32})  [unwired: 1 in]
            n333 = property on="Image Out" class="ImageControl"(error in=w895, "Image Center Position"=w898) -> ()  [unwired: 1 in, 2 out]
            n334 = Path To String(path=w938) -> (string=w957:string)
            n335 = Index Array(array=w952, index=w893) -> (element=w953:string)
            n336 = local write "Data Name:"(w953) -> ()
            n337 = Concatenate Strings(w957, "\\", w953) -> (w955:string)
            n338 = String To Path(string=w955) -> (path=w864:path)
            n339 = call "Recorded Values.vi"("Path"=w864) -> ("Recorded Char"=w959:T5, "Recorded Prop"=w960:T6, "Fabrication Prop"=w958:T7)  [unwired: 8 in]
            n340 = Unbundle By Name(w959) -> ("Mobility-Sat"=w972:dbl, "Moblitity-Lin"=w973:dbl, "On/Off"=w974:dbl, "Off Current"=w975:dbl, "STS"=w976:dbl, "Trap Density-VT"=w977:dbl, "Trap Density-STS"=w978:dbl)  [unwired: 1 out]
            n341 = Unbundle By Name(w958) -> ("Date Created"=w979:string, "Material"=w961:string, "Solvent"=w962:string, "Concentration"=w963:dbl, "Method"=w964:string, "Dielectric (nm)"=w965:dbl, "Treatment"=w966:string, "Comments"=w967:string)
            n342 = Unbundle By Name(w960) -> ("Date Recorded"=w968:string, "Index"=w969:string, "Length"=w970:dbl, "Width"=w971:dbl, "Sample Temp"=w861:dbl)
            n343 = local write "Date Created"(w979) -> ()
            n344 = local write "Rec: VT-Sat"(w975) -> ()
            n345 = local write "Rec: Material"(w961) -> ()
            n346 = local write "Rec: Concentration"(w963) -> ()
            n347 = local write "Rec: Method"(w964) -> ()
            n348 = local write "Rec: Dielectric (d)"(w965) -> ()
            n349 = local write "Surface Treatment:"(w966) -> ()
            n350 = local write "Comments"(w967) -> ()
            n351 = local write "Index"(w969) -> ()
            n352 = local write "Rec: Mobility-Sat"(w972) -> ()
            n353 = local write "Rec: Mobility-Lin"(w973) -> ()
            n354 = local write "Rec: On/Off"(w974) -> ()
            n355 = local write "Rec: STS"(w976) -> ()
            n356 = local write "Rec: Trap Density-VT"(w977) -> ()
            n357 = local write "Rec: Trap Density-STS"(w978) -> ()
            n358 = local write "Rec: Solvent"(w962) -> ()
            n359 = local write "Date Recorded"(w968) -> ()
            n360 = local write "Rec: Length"(w970) -> ()
            n361 = local write "Rec: Width"(w971) -> ()
            n362 = local write "Rec: Temp"(w861) -> ()
            n363 = Equal To 0?(x=w861) -> (x = 0?=w862:bool)
            n364 = case shown="True" w862 {
              tunnel: [w980 w981] -> w860
              tunnel: w861 -> [w980 _]
              frame False {
              }
              frame True {
                n365 = local read "Room Temp"() -> (w981:dbl)
              }
            }
            n366 = local read "NumPts 2"() -> (w886:dbl)
            n367 = local read "NumPts"() -> (w890:dbl)
            n368 = local write "Data File"(w864) -> ()
            n369 = call-poly <vilib>:"Read From Spreadsheet File.vi"("file path (dialog if empty)"=w864) -> ("all rows"=w944:string[][])  [unwired: 6 in, 4 out]
            n370 = call "Mobility-Vt Calculator-File.vi"("NumPts"=w890, "Path"=w864) -> ("XY Graph-Sat"=w888:cluster{dbl[], dbl[]}[], "XY Graph-Lin"=w874:cluster{dbl[], dbl[]}[], "Output"=w889:T8, "Index-Sat"=w887:dbl, "Index-Lin"=w872:dbl)  [unwired: 4 in, 1 out]
            n371 = local read "New: Dielectric"() -> (w869:dbl)
            n372 = call "STS Calculator-File.vi"("NumPts"=w886, "Path"=w864) -> ("STS Index-Sat"=w885:dbl, "XY Graph-Sat"=w884:cluster{dbl[], dbl[]}[], "Ouput"=w883:cluster{"STS-Sat":dbl, "STS-Lin":dbl})  [unwired: 5 in, 2 out]
            n373 = Unbundle By Name(w889) -> ("Mobility-Sat"=w882:dbl, "Vt-Sat"=w868:dbl, "Mobility-Lin"=w881:dbl, "Vt-Lin"=w880:dbl, "Off I-Sat"=w865:dbl)
            n374 = Unbundle By Name(w883) -> ("STS-Sat"=w863:dbl)  [unwired: 1 out]
            n375 = local write "Index 2"(w885) -> ()
            n376 = local write "XY Graph 2"(w884) -> ()
            n377 = local write "MobVi Index"(w887) -> ()
            n378 = local write "Slide"(w887) -> ()
            n379 = local write "XY Graph"(w888) -> ()
            n380 = Array Size(array=w944) -> (size(s)=w943:i32[])
            n381 = call "Trap Density_VT.vi"("VT"=w868, "Dielectric"=w869) -> ("Trap Density-VT"=w867:dbl)
            n382 = call "Trap Density_STS.vi"("Temp (T) [K]"=w860, "S.T.S. (S)"=w863, "Dielectric"=w869) -> ("Trap Density (N)"=w866:dbl)  [unwired: 8 in]
            n383 = local write "New: STS"(w863) -> ()
            n384 = local write "Calc: Mobility-Lin"(w880) -> ()
            n385 = local write "Calc: Mobility-Sat"(w882) -> ()
            n386 = local write "Calc: STS"(w863) -> ()
            n387 = local write "Calc: VT-Sat"(w868) -> ()
            n388 = local write "Calc: Off I-Sat"(w865) -> ()
            n389 = local write "Calc: VT-Lin"(w881) -> ()
            n390 = Index Array(array=w943, index=w942) -> (element=w924:i32)
            n391 = Decimate 1D Array(w884) -> (w918:cluster{dbl[], dbl[]}[])  [unwired: 1 out]
            n392 = Decimate 1D Array(w888) -> (w928:cluster{dbl[], dbl[]}[])  [unwired: 1 out]
            n393 = Decimate 1D Array(w874) -> (w879:cluster{dbl[], dbl[]}[])  [unwired: 1 out]
            n394 = Array Subset(array=w944, index (row)=w942, index (col)=w942, length (col)=3) -> (w945:string[][])  [unwired: 1 in]
            n395 = local write "Calc: Trap Density-VT"(w867) -> ()
            n396 = local write "Calc: Trap Density-STS"(w866) -> ()
            n397 = local write "New: Trap Density-STS"(w866) -> ()
            n398 = local write "New: Trap Density-VT"(w867) -> ()
            n399 = Array To Cluster(array=w918) -> (cluster=w916:T9)
            n400 = Array To Cluster(array=w928) -> (cluster=w930:T9)
            n401 = Reshape Array(w945, w924) -> (w931:string[])
            n402 = Array To Cluster(array=w879) -> (cluster=w878:T9)
            n403 = Subtract(x=w924, y=20) -> (x-y=w923:i32)
            n404 = local write "New: Mobility-Sat"(w882) -> ()
            n405 = local write "New: Mobility-Lin"(w881) -> ()
            n406 = local write "New: VT-Sat"(w868) -> ()
            n407 = local write "New: VT-Lin"(w880) -> ()
            n408 = property on="Slide" class="Slide (strict)"("Scale.Maximum"=w923) -> ()  [unwired: 2 in, 2 out]
            n409 = Unbundle(w916) -> ("[0]"=w917:cluster{dbl[], dbl[]})  [unwired: 8 out]
            n410 = Unbundle(w930) -> ("[0]"=w929:cluster{dbl[], dbl[]})  [unwired: 8 out]
            n411 = Unbundle(w878) -> ("[0]"=w875:cluster{dbl[], dbl[]})  [unwired: 8 out]
            n412 = Search 1D Array(1D array=w931, element="Index:") -> (index of element=w939:i32)  [unwired: 1 in]
            n413 = local read "NumPts"() -> (w873:dbl)
            n414 = Unbundle(w875) -> (w877:dbl[], w876:dbl[])
            n415 = Increment(x=w939) -> (x+1=w940:i32)
            n416 = Unbundle(w917) -> (w915:dbl[], w914:dbl[])
            n417 = Unbundle(w929) -> (w920:dbl[], w919:dbl[])
            n418 = Array Subset(array=w877, index=w872, length=w873) -> (w871:dbl[])
            n419 = Array Subset(array=w876, index=w872, length=w873) -> (w870:dbl[])
            n420 = Array Subset(array=w915, index=w885, length=w886) -> (w922:dbl[])
            n421 = Array Subset(array=w914, index=w885, length=w886) -> (w921:dbl[])
            n422 = Array Subset(array=w920, index=w887, length=w890) -> (w927:dbl[])
            n423 = Array Subset(array=w919, index=w887, length=w890) -> (w926:dbl[])
            n424 = Index Array(array=w931, index=w940) -> (element=w903:string)
            n425 = local write "Lin-Vg Array-Used"(w871) -> ()
            n426 = local write "Sat Vg Array-Used"(w927) -> ()
            n427 = local write "Vg Array-Log-Used"(w921) -> ()
            n428 = local write "Lin Id-Used"(w870) -> ()
            n429 = local read "Image Folder"() -> (w901:path)
            n430 = local write "Sat Id-Used"(w926) -> ()
            n431 = local write "Sat Id-Log-Used"(w922) -> ()
            n432 = List Folder(path=w901, error in=w891) -> (filenames=w937:string[], error out=w904:errorcluster)  [unwired: 2 in, 2 out]
            n433 = while {
              tunnel: w937 -> [w994]
              tunnel: w903 -> [w992]
              tunnel: [w991] -> _
              tunnel: [w991] -> w936
              tunnel: w924 -> [w990]
              i -> [w991]
              stop <- w987 stop-if-true
              n434 = Index Array(array=w994, index=w991) -> (element=w995:string)
              n435 = xnode "Match Regular Expression"("input string"=w995, "regular expression"=w992) -> ("whole match"=w993:string)  [unwired: 4 in, 4 out]
              n436 = Equal?(x=w993, y=w992) -> (x = y?=w989:bool)
              n437 = Equal?(x=w990, y=w991) -> (x = y?=w988:bool)
              n438 = Or(x=w989, y=w988) -> (x .or. y?=w987:bool)
            }
            n439 = Build Path(base path=w901, name or relative path="ROI") -> (appended path=w900:path)
            n440 = Path To String(path=w901) -> (string=w934:string)
            n441 = Index Array(array=w937, index=w936) -> (element=w912:string)
            n442 = invoke on="Image Out" class="ImageControl" method="Clear ROI"(error in=w904) -> (error out=w907:errorcluster)  [unwired: 2 in, 2 out]
            n443 = local write "Image Name"(w912) -> ()
            n444 = Build Path(base path=w900, name or relative path=w903) -> (appended path=w908:path)
            n445 = call <vilib>:"Check if File or Folder Exists.vi"("error in (no error)"=w907, "path"=w908) -> ("file or folder exists?"=w905:bool, "dup path"=w906:path)  [unwired: 7 in, 1 out]
            n446 = Concatenate Strings(w934, "\\", w912) -> (w933:string)
            n447 = case shown="False" w905 {
              tunnel: w906 -> [_ w982]
              frame False {
              }
              frame True {
                n448 = Read from Text File(file (use dialog)=w982) -> (text=w986:string)  [unwired: 3 in, 3 out]
                n449 = property on="Image Out" class="ImageControl"() -> ("ROI"=w983:T10)  [unwired: 2 in, 2 out]
                n450 = Unflatten From String(type=w983, binary string=w986) -> (value=w984:T10, error out=w985:errorcluster)  [unwired: 3 in, 1 out]
                n451 = property on="Image Out" class="ImageControl"(error in=w985, "ROI"=w984) -> ()  [unwired: 1 in, 2 out]
              }
            }
            n452 = String To Path(string=w933) -> (path=w911:path)
            n453 = Empty String/Path?(string/path=w912) -> (empty?=w913:bool)
            n454 = local read "No Image"() -> (w909:path)
            n455 = Select(t=w909, s=w913, f=w911) -> (s? t:f=w910:path)
            n456 = local write "Image File"(w910) -> ()
            n457 = call "Vision Acquisition4"("Image Path"=w910) -> ("Image Out"=w935:T2)  [unwired: 25 in, 1 out]
            n458 = local write "Image Out"(w935) -> ()
            n459 = local write "Image Out 2"(w935) -> ()
          }
          event "Data File": Value Change {
            w1216 = 0
            n460 = event-data() -> ()  [unwired: 1 in, 5 out]
            n461 = local read "Data File"() -> (w1212:path)
            n462 = Strip Path(path=w1212) -> (stripped path=w1211:path, name=w1225:string)
            n463 = local write "Data Folder"(w1211) -> ()
            n464 = property on="Image Out" class="ImageControl"() -> (error out=w1167:errorcluster, "Image Center Position"=w1171:cluster{"X":u32, "Y":u32})  [unwired: 2 in, 1 out]
            n465 = List Folder(path=w1211) -> (filenames=w1221:string[], error out=w1177:errorcluster)  [unwired: 3 in, 2 out]
            n466 = Search 1D Array(1D array=w1221, element=w1225) -> (index of element=w1166:i32)  [unwired: 1 in]
            n467 = local write "Folder Index"(w1166) -> ()
            n468 = Unbundle(w1171) -> ("X"=w1169:u32)  [unwired: 1 out]
            n469 = Path To String(path=w1211) -> (string=w1226:string)
            n470 = Index Array(array=w1221, index=w1166) -> (element=w1222:string)
            n471 = Bundle("X"=w1169, 0) -> (w1170:cluster{"X":u32, i32})  [unwired: 1 in]
            n472 = local write "Data Name:"(w1222) -> ()
            n473 = property on="Image Out" class="ImageControl"(error in=w1167, "Image Center Position"=w1170) -> ()  [unwired: 1 in, 2 out]
            n474 = Concatenate Strings(w1226, "\\", w1222) -> (w1224:string)
            n475 = String To Path(string=w1224) -> (path=w1115:path)
            n476 = call "Recorded Values.vi"("Path"=w1115) -> ("Recorded Char"=w1164:T5, "Recorded Prop"=w1163:T6, "Fabrication Prop"=w1165:T7)  [unwired: 8 in]
            n477 = Unbundle By Name(w1164) -> ("Mobility-Sat"=w1151:dbl, "Moblitity-Lin"=w1150:dbl, "On/Off"=w1149:dbl, "Off Current"=w1148:dbl, "STS"=w1147:dbl, "Trap Density-VT"=w1146:dbl, "Trap Density-STS"=w1145:dbl)  [unwired: 1 out]
            n478 = Unbundle By Name(w1165) -> ("Date Created"=w1144:string, "Material"=w1162:string, "Solvent"=w1161:string, "Concentration"=w1160:dbl, "Method"=w1159:string, "Dielectric (nm)"=w1158:dbl, "Treatment"=w1157:string, "Comments"=w1156:string)
            n479 = Unbundle By Name(w1163) -> ("Date Recorded"=w1155:string, "Index"=w1154:string, "Length"=w1153:dbl, "Width"=w1152:dbl, "Sample Temp"=w1113:dbl)
            n480 = local write "Date Created"(w1144) -> ()
            n481 = local write "Rec: Material"(w1162) -> ()
            n482 = local write "Rec: VT-Sat"(w1148) -> ()
            n483 = local write "Rec: Concentration"(w1160) -> ()
            n484 = local write "Rec: Method"(w1159) -> ()
            n485 = local write "Rec: Dielectric (d)"(w1158) -> ()
            n486 = local write "Surface Treatment:"(w1157) -> ()
            n487 = local write "Comments"(w1156) -> ()
            n488 = local write "Index"(w1154) -> ()
            n489 = local write "Rec: Mobility-Sat"(w1151) -> ()
            n490 = local write "Rec: Mobility-Lin"(w1150) -> ()
            n491 = local write "Rec: On/Off"(w1149) -> ()
            n492 = local write "Rec: STS"(w1147) -> ()
            n493 = local write "Rec: Trap Density-VT"(w1146) -> ()
            n494 = local write "Rec: Trap Density-STS"(w1145) -> ()
            n495 = local write "Rec: Solvent"(w1161) -> ()
            n496 = local write "Date Recorded"(w1155) -> ()
            n497 = local write "Rec: Length"(w1153) -> ()
            n498 = local write "Rec: Width"(w1152) -> ()
            n499 = local write "Rec: Temp"(w1113) -> ()
            n500 = Equal To 0?(x=w1113) -> (x = 0?=w1114:bool)
            n501 = case shown="False" w1114 {
              tunnel: [w1227 w1228] -> w1112
              tunnel: w1113 -> [w1227 _]
              frame False {
              }
              frame True {
                n502 = local read "Room Temp"() -> (w1228:dbl)
              }
            }
            n503 = local read "NumPts 2"() -> (w1139:dbl)
            n504 = local write "Data File"(w1115) -> ()
            n505 = local read "NumPts"() -> (w1140:dbl)
            n506 = call-poly <vilib>:"Read From Spreadsheet File.vi"("file path (dialog if empty)"=w1115) -> ("all rows"=w1218:string[][])  [unwired: 6 in, 4 out]
            n507 = local read "New: Dielectric"() -> (w1121:dbl)
            n508 = call "STS Calculator-File.vi"("NumPts"=w1139, "Path"=w1115) -> ("STS Index-Sat"=w1137:dbl, "XY Graph-Sat"=w1138:cluster{dbl[], dbl[]}[], "Ouput"=w1136:cluster{"STS-Sat":dbl, "STS-Lin":dbl})  [unwired: 5 in, 2 out]
            n509 = call "Mobility-Vt Calculator-File.vi"("NumPts"=w1140, "Path"=w1115) -> ("XY Graph-Sat"=w1143:cluster{dbl[], dbl[]}[], "XY Graph-Lin"=w1133:cluster{dbl[], dbl[]}[], "Output"=w1141:T8, "Index-Sat"=w1142:dbl, "Index-Lin"=w1128:dbl)  [unwired: 4 in, 1 out]
            n510 = Unbundle By Name(w1141) -> ("Mobility-Sat"=w1124:dbl, "Vt-Sat"=w1117:dbl, "Mobility-Lin"=w1123:dbl, "Mobility-Lin"=w1122:dbl, "Off I-Sat"=w1116:dbl)
            n511 = local write "Index 2"(w1137) -> ()
            n512 = local write "XY Graph 2"(w1138) -> ()
            n513 = Unbundle By Name(w1136) -> ("STS-Sat"=w1118:dbl)  [unwired: 1 out]
            n514 = local write "MobVi Index"(w1142) -> ()
            n515 = Array Size(array=w1218) -> (size(s)=w1217:i32[])
            n516 = call "Trap Density_VT.vi"("VT"=w1117, "Dielectric"=w1121) -> ("Trap Density-VT"=w1120:dbl)
            n517 = call "Trap Density_STS.vi"("Temp (T) [K]"=w1112, "S.T.S. (S)"=w1118, "Dielectric"=w1121) -> ("Trap Density (N)"=w1119:dbl)  [unwired: 8 in]
            n518 = local write "Slide"(w1142) -> ()
            n519 = local write "Calc: Mobility-Sat"(w1124) -> ()
            n520 = local write "Calc: Mobility-Lin"(w1122) -> ()
            n521 = local write "Calc: Off I-Sat"(w1116) -> ()
            n522 = local write "Calc: VT-Sat"(w1117) -> ()
            n523 = local write "Calc: VT-Lin"(w1123) -> ()
            n524 = local write "Calc: STS"(w1118) -> ()
            n525 = Decimate 1D Array(w1133) -> (w1135:cluster{dbl[], dbl[]}[])  [unwired: 1 out]
            n526 = local write "Calc: Trap Density-VT"(w1120) -> ()
            n527 = local write "Calc: Trap Density-STS"(w1119) -> ()
            n528 = local write "New: Trap Density-STS"(w1119) -> ()
            n529 = local write "New: Trap Density-VT"(w1120) -> ()
            n530 = Decimate 1D Array(w1138) -> (w1192:cluster{dbl[], dbl[]}[])  [unwired: 1 out]
            n531 = Index Array(array=w1217, index=w1216) -> (element=w1198:i32)
            n532 = Decimate 1D Array(w1143) -> (w1201:cluster{dbl[], dbl[]}[])  [unwired: 1 out]
            n533 = local write "XY Graph"(w1143) -> ()
            n534 = Array Subset(array=w1218, index (row)=w1216, index (col)=w1216, length (col)=3) -> (w1219:string[][])  [unwired: 1 in]
            n535 = Array To Cluster(array=w1135) -> (cluster=w1134:T9)
            n536 = local write "New: STS"(w1118) -> ()
            n537 = Array To Cluster(array=w1192) -> (cluster=w1190:T9)
            n538 = Array To Cluster(array=w1201) -> (cluster=w1203:T9)
            n539 = Reshape Array(w1219, w1198) -> (w1204:string[])
            n540 = local write "New: Mobility-Sat"(w1124) -> ()
            n541 = local write "New: Mobility-Lin"(w1123) -> ()
            n542 = Subtract(x=w1198, y=20) -> (x-y=w1196:i32)
            n543 = local write "New: VT-Sat"(w1117) -> ()
            n544 = local write "New: VT-Lin"(w1122) -> ()
            n545 = Unbundle(w1134) -> ("[0]"=w1132:cluster{dbl[], dbl[]})  [unwired: 8 out]
            n546 = property on="Slide" class="Slide (strict)"("Scale.Maximum"=w1196) -> ()  [unwired: 2 in, 2 out]
            n547 = local read "NumPts"() -> (w1129:dbl)
            n548 = Unbundle(w1132) -> (w1131:dbl[], w1130:dbl[])
            n549 = Unbundle(w1190) -> ("[0]"=w1191:cluster{dbl[], dbl[]})  [unwired: 8 out]
            n550 = Unbundle(w1203) -> ("[0]"=w1202:cluster{dbl[], dbl[]})  [unwired: 8 out]
            n551 = Search 1D Array(1D array=w1204, element="Index:") -> (index of element=w1213:i32)  [unwired: 1 in]
            n552 = local read "NumPts"() -> (w1125:dbl)
            n553 = Array Subset(array=w1131, index=w1128, length=w1129) -> (w1127:dbl[])
            n554 = Array Subset(array=w1130, index=w1128, length=w1129) -> (w1126:dbl[])
            n555 = Increment(x=w1213) -> (x+1=w1214:i32)
            n556 = Unbundle(w1191) -> (w1188:dbl[], w1187:dbl[])
            n557 = Unbundle(w1202) -> (w1189:dbl[], w1193:dbl[])
            n558 = local read "Image Folder"() -> (w1173:path)
            n559 = local write "Lin-Vg Array-Used"(w1127) -> ()
            n560 = Array Subset(array=w1188, index=w1137, length=w1139) -> (w1195:dbl[])
            n561 = Array Subset(array=w1187, index=w1137, length=w1139) -> (w1194:dbl[])
            n562 = Array Subset(array=w1189, index=w1142, length=w1125) -> (w1200:dbl[])
            n563 = Array Subset(array=w1193, index=w1142, length=w1125) -> (w1199:dbl[])
            n564 = Index Array(array=w1204, index=w1214) -> (element=w1175:string)
            n565 = local write "Lin Id-Used"(w1126) -> ()
            n566 = local write "Sat Vg Array-Used"(w1200) -> ()
            n567 = local write "Vg Array-Log-Used"(w1194) -> ()
            n568 = local write "Sat Id-Log-Used"(w1195) -> ()
            n569 = local write "Sat Id-Used"(w1199) -> ()
            n570 = local write "Index"(w1175) -> ()
            n571 = List Folder(path=w1173, error in=w1177) -> (filenames=w1209:string[], error out=w1176:errorcluster)  [unwired: 2 in, 2 out]
            n572 = Build Path(base path=w1173, name or relative path="ROI") -> (appended path=w1172:path)
            n573 = while {
              tunnel: w1209 -> [w1241]
              tunnel: w1175 -> [w1239]
              tunnel: [w1238] -> _
              tunnel: [w1238] -> w1208
              tunnel: w1198 -> [w1237]
              i -> [w1238]
              stop <- w1234 stop-if-true
              n574 = Index Array(array=w1241, index=w1238) -> (element=w1242:string)
              n575 = xnode "Match Regular Expression"("input string"=w1242, "regular expression"=w1239) -> ("whole match"=w1240:string)  [unwired: 4 in, 4 out]
              n576 = Equal?(x=w1240, y=w1239) -> (x = y?=w1236:bool)
              n577 = Equal?(x=w1237, y=w1238) -> (x = y?=w1235:bool)
              n578 = Or(x=w1236, y=w1235) -> (x .or. y?=w1234:bool)
            }
            n579 = invoke on="Image Out" class="ImageControl" method="Clear ROI"(error in=w1176) -> (error out=w1180:errorcluster)  [unwired: 2 in, 2 out]
            n580 = Build Path(base path=w1172, name or relative path=w1175) -> (appended path=w1181:path)
            n581 = call <vilib>:"Check if File or Folder Exists.vi"("error in (no error)"=w1180, "path"=w1181) -> ("file or folder exists?"=w1178:bool, "dup path"=w1179:path)  [unwired: 7 in, 1 out]
            n582 = case shown="True" w1178 {
              tunnel: w1179 -> [_ w1229]
              frame False {
              }
              frame True {
                n583 = Read from Text File(file (use dialog)=w1229) -> (text=w1233:string)  [unwired: 3 in, 3 out]
                n584 = property on="Image Out" class="ImageControl"() -> ("ROI"=w1230:T10)  [unwired: 2 in, 2 out]
                n585 = Unflatten From String(type=w1230, binary string=w1233) -> (value=w1231:T10, error out=w1232:errorcluster)  [unwired: 3 in, 1 out]
                n586 = property on="Image Out" class="ImageControl"(error in=w1232, "ROI"=w1231) -> ()  [unwired: 1 in, 2 out]
              }
            }
            n587 = invoke on="Image Out" class="ImageControl" method="Clear ROI"() -> ()  [unwired: 3 in, 3 out]
            n588 = Path To String(path=w1173) -> (string=w1207:string)
            n589 = Index Array(array=w1209, index=w1208) -> (element=w1185:string)
            n590 = Concatenate Strings(w1207, "\\", w1185) -> (w1206:string)
            n591 = local write "Image Name"(w1185) -> ()
            n592 = String To Path(string=w1206) -> (path=w1184:path)
            n593 = Empty String/Path?(string/path=w1185) -> (empty?=w1186:bool)
            n594 = local read "No Image"() -> (w1182:path)
            n595 = Select(t=w1182, s=w1186, f=w1184) -> (s? t:f=w1183:path)
            n596 = local write "Image File"(w1183) -> ()
            n597 = call "Vision Acquisition3"("Image Path"=w1183) -> ("Image Out"=w1210:T2)  [unwired: 25 in, 1 out]
            n598 = local write "Image Out"(w1210) -> ()
            n599 = local write "Image Out 2"(w1210) -> ()
          }
          event "Up Button": Mouse Down {
            w1459 = 0
            n600 = event-data() -> ()  [unwired: 1 in, 5 out]
            n601 = local read "Data File"() -> (w1455:path)
            n602 = Strip Path(path=w1455) -> (stripped path=w1454:path, name=w1470:string)
            n603 = local write "Data Folder"(w1454) -> ()
            n604 = List Folder(path=w1454) -> (filenames=w1464:string[], error out=w1421:errorcluster)  [unwired: 3 in, 2 out]
            n605 = Array Size(array=w1464) -> (size(s)=w1409:i32)
            n606 = Search 1D Array(1D array=w1464, element=w1470) -> (index of element=w1465:i32)  [unwired: 1 in]
            n607 = Equal To 0?(x=w1465) -> (x = 0?=w1466:bool)
            n608 = local read "Folder Index"() -> (w1408:dbl)
            n609 = property on="Image Out" class="ImageControl"() -> (error out=w1411:errorcluster, "Image Center Position"=w1415:cluster{"X":u32, "Y":u32})  [unwired: 2 in, 1 out]
            n610 = case shown="True" w1466 {
              tunnel: w1408 -> [w1600 _]
              tunnel: [w1599 w1601] -> w1407
              tunnel: w1409 -> [_ w1602]
              frame False {
                n611 = Decrement(x=w1600) -> (x-1=w1599:dbl)
              }
              frame True {
                n612 = Decrement(x=w1602) -> (x-1=w1601:i32)
              }
            }
            n613 = Unbundle(w1415) -> ("X"=w1413:u32)  [unwired: 1 out]
            n614 = local write "Folder Index"(w1407) -> ()
            n615 = Bundle("X"=w1413, 0) -> (w1414:cluster{"X":u32, i32})  [unwired: 1 in]
            n616 = Path To String(path=w1454) -> (string=w1471:string)
            n617 = Index Array(array=w1464, index=w1407) -> (element=w1467:string)
            n618 = local write "Data Name:"(w1467) -> ()
            n619 = property on="Image Out" class="ImageControl"(error in=w1411, "Image Center Position"=w1414) -> ()  [unwired: 1 in, 2 out]
            n620 = Concatenate Strings(w1471, "\\", w1467) -> (w1469:string)
            n621 = String To Path(string=w1469) -> (path=w1357:path)
            n622 = call "Recorded Values.vi"("Path"=w1357) -> ("Recorded Char"=w1405:T5, "Recorded Prop"=w1404:T6, "Fabrication Prop"=w1406:T7)  [unwired: 8 in]
            n623 = Unbundle By Name(w1405) -> ("Mobility-Sat"=w1392:dbl, "Moblitity-Lin"=w1391:dbl, "On/Off"=w1390:dbl, "Off Current"=w1389:dbl, "STS"=w1388:dbl, "Trap Density-VT"=w1387:dbl, "Trap Density-STS"=w1386:dbl)  [unwired: 1 out]
            n624 = Unbundle By Name(w1406) -> ("Date Created"=w1385:string, "Material"=w1403:string, "Solvent"=w1402:string, "Concentration"=w1401:dbl, "Method"=w1400:string, "Dielectric (nm)"=w1399:dbl, "Treatment"=w1398:string, "Comments"=w1397:string)
            n625 = Unbundle By Name(w1404) -> ("Date Recorded"=w1396:string, "Index"=w1395:string, "Length"=w1394:dbl, "Width"=w1393:dbl, "Sample Temp"=w1354:dbl)
            n626 = local write "Date Created"(w1385) -> ()
            n627 = local write "Rec: Material"(w1403) -> ()
            n628 = local write "Rec: VT-Sat"(w1389) -> ()
            n629 = local write "Rec: Solvent"(w1402) -> ()
            n630 = local write "Rec: Concentration"(w1401) -> ()
            n631 = local write "Rec: Method"(w1400) -> ()
            n632 = local write "Rec: Dielectric (d)"(w1399) -> ()
            n633 = local write "Surface Treatment:"(w1398) -> ()
            n634 = local write "Comments"(w1397) -> ()
            n635 = local write "Index"(w1395) -> ()
            n636 = local write "Rec: Mobility-Sat"(w1392) -> ()
            n637 = local write "Rec: Mobility-Lin"(w1391) -> ()
            n638 = local write "Rec: On/Off"(w1390) -> ()
            n639 = local write "Rec: STS"(w1388) -> ()
            n640 = local write "Rec: Trap Density-VT"(w1387) -> ()
            n641 = local write "Rec: Trap Density-STS"(w1386) -> ()
            n642 = local write "Date Recorded"(w1396) -> ()
            n643 = local write "Rec: Length"(w1394) -> ()
            n644 = local write "Rec: Width"(w1393) -> ()
            n645 = local write "Rec: Temp"(w1354) -> ()
            n646 = Equal To 0?(x=w1354) -> (x = 0?=w1356:bool)
            n647 = case shown="False" w1356 {
              tunnel: [w1472 w1473] -> w1355
              tunnel: w1354 -> [w1472 _]
              frame False {
              }
              frame True {
                n648 = local read "Room Temp"() -> (w1473:dbl)
              }
            }
            n649 = local read "NumPts 2"() -> (w1380:dbl)
            n650 = local write "Data File"(w1357) -> ()
            n651 = local read "NumPts"() -> (w1384:dbl)
            n652 = local read "New: Dielectric"() -> (w1363:dbl)
            n653 = call "Mobility-Vt Calculator-File.vi"("NumPts"=w1384, "Path"=w1357) -> ("XY Graph-Sat"=w1382:cluster{dbl[], dbl[]}[], "XY Graph-Lin"=w1367:cluster{dbl[], dbl[]}[], "Output"=w1383:T8, "Index-Sat"=w1381:dbl, "Index-Lin"=w1368:dbl)  [unwired: 4 in, 1 out]
            n654 = call "STS Calculator-File.vi"("NumPts"=w1380, "Path"=w1357) -> ("STS Index-Sat"=w1379:dbl, "XY Graph-Sat"=w1378:cluster{dbl[], dbl[]}[], "Ouput"=w1377:cluster{"STS-Sat":dbl, "STS-Lin":dbl})  [unwired: 5 in, 2 out]
            n655 = call-poly <vilib>:"Read From Spreadsheet File.vi"("file path (dialog if empty)"=w1357) -> ("all rows"=w1461:string[][])  [unwired: 6 in, 4 out]
            n656 = Unbundle By Name(w1383) -> ("Mobility-Sat"=w1366:dbl, "Vt-Sat"=w1359:dbl, "Mobility-Lin"=w1365:dbl, "Mobility-Lin"=w1364:dbl, "Off I-Sat"=w1358:dbl)
            n657 = Unbundle By Name(w1377) -> ("STS-Sat"=w1360:dbl)  [unwired: 1 out]
            n658 = local write "Index 2"(w1379) -> ()
            n659 = local write "XY Graph 2"(w1378) -> ()
            n660 = local write "MobVi Index"(w1381) -> ()
            n661 = local write "Slide"(w1381) -> ()
            n662 = local write "XY Graph"(w1382) -> ()
            n663 = Array Size(array=w1461) -> (size(s)=w1460:i32[])
            n664 = local write "Calc: Mobility-Sat"(w1366) -> ()
            n665 = local write "Calc: Mobility-Lin"(w1364) -> ()
            n666 = call "Trap Density_VT.vi"("VT"=w1359, "Dielectric"=w1363) -> ("Trap Density-VT"=w1362:dbl)
            n667 = call "Trap Density_STS.vi"("Temp (T) [K]"=w1355, "S.T.S. (S)"=w1360, "Dielectric"=w1363) -> ("Trap Density (N)"=w1361:dbl)  [unwired: 8 in]
            n668 = local write "Calc: VT-Sat"(w1359) -> ()
            n669 = local write "Calc: Off I-Sat"(w1358) -> ()
            n670 = local write "Calc: VT-Lin"(w1365) -> ()
            n671 = local write "Calc: STS"(w1360) -> ()
            n672 = local write "New: STS"(w1360) -> ()
            n673 = Decimate 1D Array(w1367) -> (w1376:cluster{dbl[], dbl[]}[])  [unwired: 1 out]
            n674 = local write "Calc: Trap Density-VT"(w1362) -> ()
            n675 = local write "Calc: Trap Density-STS"(w1361) -> ()
            n676 = local write "New: Trap Density-STS"(w1361) -> ()
            n677 = local write "New: Trap Density-VT"(w1362) -> ()
            n678 = Decimate 1D Array(w1378) -> (w1438:cluster{dbl[], dbl[]}[])  [unwired: 1 out]
            n679 = Index Array(array=w1460, index=w1459) -> (element=w1444:i32)
            n680 = Decimate 1D Array(w1382) -> (w1448:cluster{dbl[], dbl[]}[])  [unwired: 1 out]
            n681 = Array To Cluster(array=w1376) -> (cluster=w1375:T9)
            n682 = Array Subset(array=w1461, index (row)=w1459, index (col)=w1459, length (col)=3) -> (w1462:string[][])  [unwired: 1 in]
            n683 = Array To Cluster(array=w1438) -> (cluster=w1436:T9)
            n684 = Array To Cluster(array=w1448) -> (cluster=w1450:T9)
            n685 = Reshape Array(w1462, w1444) -> (w1451:string[])
            n686 = Subtract(x=w1444, y=20) -> (x-y=w1443:i32)
            n687 = Unbundle(w1375) -> ("[0]"=w1372:cluster{dbl[], dbl[]})  [unwired: 8 out]
            n688 = local write "New: Mobility-Sat"(w1366) -> ()
            n689 = local write "New: Mobility-Lin"(w1365) -> ()
            n690 = local write "New: VT-Sat"(w1359) -> ()
            n691 = local write "New: VT-Lin"(w1364) -> ()
            n692 = property on="Slide" class="Slide (strict)"("Scale.Maximum"=w1443) -> ()  [unwired: 2 in, 2 out]
            n693 = Unbundle(w1436) -> ("[0]"=w1437:cluster{dbl[], dbl[]})  [unwired: 8 out]
            n694 = Unbundle(w1450) -> ("[0]"=w1449:cluster{dbl[], dbl[]})  [unwired: 8 out]
            n695 = local read "NumPts"() -> (w1369:dbl)
            n696 = Unbundle(w1372) -> (w1371:dbl[], w1370:dbl[])
            n697 = Search 1D Array(1D array=w1451, element="Index:") -> (index of element=w1456:i32)  [unwired: 1 in]
            n698 = Increment(x=w1456) -> (x+1=w1457:i32)
            n699 = Unbundle(w1437) -> (w1435:dbl[], w1434:dbl[])
            n700 = Unbundle(w1449) -> (w1442:dbl[], w1441:dbl[])
            n701 = Array Subset(array=w1371, index=w1368, length=w1369) -> (w1373:dbl[])
            n702 = Array Subset(array=w1370, index=w1368, length=w1369) -> (w1374:dbl[])
            n703 = local read "Image Folder"() -> (w1410:path)
            n704 = local write "Lin-Vg Array-Used"(w1373) -> ()
            n705 = Array Subset(array=w1435, index=w1379, length=w1380) -> (w1440:dbl[])
            n706 = Array Subset(array=w1434, index=w1379, length=w1380) -> (w1439:dbl[])
            n707 = Array Subset(array=w1442, index=w1381, length=w1384) -> (w1447:dbl[])
            n708 = Array Subset(array=w1441, index=w1381, length=w1384) -> (w1446:dbl[])
            n709 = local write "Lin Id-Used"(w1374) -> ()
            n710 = Index Array(array=w1451, index=w1457) -> (element=w1417:string)
            n711 = local write "Sat Vg Array-Used"(w1447) -> ()
            n712 = local write "Vg Array-Log-Used"(w1439) -> ()
            n713 = local write "Sat Id-Log-Used"(w1440) -> ()
            n714 = local write "Sat Id-Used"(w1446) -> ()
            n715 = local write "Index"(w1417) -> ()
            n716 = List Folder(path=w1410, error in=w1421) -> (filenames=w1453:string[], error out=w1420:errorcluster)  [unwired: 2 in, 2 out]
            n717 = Build Path(base path=w1410, name or relative path="ROI") -> (appended path=w1418:path)
            n718 = while {
              tunnel: w1453 -> [w1486]
              tunnel: w1417 -> [w1484]
              tunnel: [w1483] -> w1452
              tunnel: w1444 -> [w1482]
              i -> [w1483]
              stop <- w1479 stop-if-true
              n719 = Index Array(array=w1486, index=w1483) -> (element=w1487:string)
              n720 = xnode "Match Regular Expression"("input string"=w1487, "regular expression"=w1484) -> ("whole match"=w1485:string)  [unwired: 4 in, 4 out]
              n721 = Equal?(x=w1485, y=w1484) -> (x = y?=w1481:bool)
              n722 = Equal?(x=w1482, y=w1483) -> (x = y?=w1480:bool)
              n723 = Or(x=w1481, y=w1480) -> (x .or. y?=w1479:bool)
            }
            n724 = invoke on="Image Out" class="ImageControl" method="Clear ROI"(error in=w1420) -> (error out=w1424:errorcluster)  [unwired: 2 in, 2 out]
            n725 = Build Path(base path=w1418, name or relative path=w1417) -> (appended path=w1416:path)
            n726 = call <vilib>:"Check if File or Folder Exists.vi"("error in (no error)"=w1424, "path"=w1416) -> ("file or folder exists?"=w1422:bool, "dup path"=w1423:path)  [unwired: 7 in, 1 out]
            n727 = case shown="True" w1422 {
              tunnel: w1423 -> [_ w1474]
              frame False {
              }
              frame True {
                n728 = Read from Text File(file (use dialog)=w1474) -> (text=w1478:string)  [unwired: 3 in, 3 out]
                n729 = property on="Image Out" class="ImageControl"() -> ("ROI"=w1475:T10)  [unwired: 2 in, 2 out]
                n730 = Unflatten From String(type=w1475, binary string=w1478) -> (value=w1476:T10, error out=w1477:errorcluster)  [unwired: 3 in, 1 out]
                n731 = property on="Image Out" class="ImageControl"(error in=w1477, "ROI"=w1476) -> ()  [unwired: 1 in, 2 out]
              }
            }
            n732 = Index Array(array=w1453, index=w1452) -> (element=w1426:string)
            n733 = local write "Image Name"(w1426) -> ()
            n734 = Empty String/Path?(string/path=w1426) -> (empty?=w1433:bool)
            n735 = Build Path(base path=w1410, name or relative path=w1426) -> (appended path=w1425:path)
            n736 = local read "No Image"() -> (w1432:path)
            n737 = Select(t=w1432, s=w1433, f=w1425) -> (s? t:f=w1427:path)
            n738 = call <vilib>:"Get File Extension.vi"("file"=w1427) -> ("lowercase file extension"=w1429:string)  [unwired: 7 in, 3 out]
            n739 = local write "Image File"(w1427) -> ()
            n740 = local write "String"(w1429) -> ()
            n741 = Search 1D Array(1D array=string[] ["bmp", "jpeg", "png", "jpg", "gif"], element=w1429) -> (index of element=w1428:i32)  [unwired: 1 in]
            n742 = call "Vision Acquisition5"("Image Path"=w1427) -> ("Image Out"=w1431:T2)  [unwired: 25 in, 1 out]
            n743 = Less Than 0?(x=w1428) -> ()  [unwired: 1 out]
            n744 = local write "Image Out"(w1431) -> ()
            n745 = local write "Image Out 2"(w1431) -> ()
          }
          event "Save Changes? 3": Mouse Down {
            n746 = event-data() -> ()  [unwired: 1 in, 7 out]
            n747 = local read "Image Folder"() -> (w1603:path)
            n748 = Build Path(base path=w1603, name or relative path="ROI") -> (appended path=w1610:path)
            n749 = call <vilib>:"Check if File or Folder Exists.vi"("path"=w1610) -> ("file or folder exists?"=w1612:bool, "dup path"=w1609:path)  [unwired: 8 in, 1 out]
            n750 = case shown="False" w1612 {
              tunnel: w1609 -> [w1614 w1615]
              tunnel: [w1613 w1615] -> w1604
              frame False {
                n751 = Create Folder(path (use dialog)=w1614) -> (created path=w1613:path)  [unwired: 2 in, 2 out]
              }
              frame True {
              }
            }
            n752 = local read "Index"() -> (w1606:string)
            n753 = property on="Image Out" class="ImageControl"() -> ("ROI"=w1608:T10)  [unwired: 2 in, 2 out]
            n754 = Build Path(base path=w1604, name or relative path=w1606) -> (appended path=w1605:path)
            n755 = Flatten To String(anything=w1608) -> (data string=w1607:string)  [unwired: 3 in, 2 out]
            n756 = Write to Text File(file (use dialog)=w1605, text=w1607) -> ()  [unwired: 2 in, 3 out]
          }
          event "Next Button": Mouse Down {
            n757 = event-data() -> ()  [unwired: 1 in, 5 out]
            n758 = local read "XY Graph"() -> (w1628:cluster{dbl[], dbl[]}[])
            n759 = Decimate 1D Array(w1628) -> (w1624:cluster{dbl[], dbl[]}[], w1623:cluster{dbl[], dbl[]}[])
            n760 = Array To Cluster(array=w1624) -> (cluster=w1634:T9)
            n761 = local read "MobVi Index"() -> (w1630:dbl)
            n762 = Unbundle(w1634) -> ("[0]"=w1633:cluster{dbl[], dbl[]})  [unwired: 8 out]
            n763 = local read "NumPts"() -> (w1629:dbl)
            n764 = Unbundle(w1633) -> (w1632:dbl[], w1631:dbl[])
            n765 = Increment(x=w1630) -> (x+1=w1625:dbl)
            n766 = local read "New: Dielectric"() -> (w1619:dbl)
            n767 = local read "New: Length"() -> (w1618:dbl)
            n768 = local read "New: Width"() -> (w1617:dbl)
            n769 = local write "MobVi Index"(w1625) -> ()
            n770 = Array Subset(array=w1632, index=w1625, length=w1629) -> (w1621:dbl[])
            n771 = Array Subset(array=w1631, index=w1625, length=w1629) -> (w1620:dbl[])
            n772 = local write "Sat Vg Array-Used"(w1621) -> ()
            n773 = local write "Sat Id-Used"(w1620) -> ()
            n774 = call "Mobility-Vt-Used Pts_Saturation.vi"("Width"=w1617, "Length"=w1618, "Dielectric (d)"=w1619, "Sat Id Used"=w1620, "Vg Used"=w1621) -> ("Vt"=w1616:dbl, "Mobility"=w1622:dbl)  [unwired: 4 in, 1 out]
            n775 = Bundle(w1621, w1620) -> (w1627:cluster{dbl[], dbl[]})  [unwired: 1 in]
            n776 = Build Array (concatenate)(w1624, w1623, w1627) -> (w1626:cluster{dbl[], dbl[]}[])
            n777 = local write "New: Mobility-Sat"(w1622) -> ()
            n778 = local write "New: VT-Sat"(w1616) -> ()
            n779 = local write "XY Graph"(w1626) -> ()
          }
          event "Next Button 2": Mouse Down {
            n780 = event-data() -> ()  [unwired: 1 in, 7 out]
            n781 = local read "XY Graph 2"() -> (w1643:cluster{dbl[], dbl[]}[])
            n782 = Decimate 1D Array(w1643) -> (w1639:cluster{dbl[], dbl[]}[], w1638:cluster{dbl[], dbl[]}[])
            n783 = Array To Cluster(array=w1639) -> (cluster=w1649:T9)
            n784 = local read "Index 2"() -> (w1645:dbl)
            n785 = Unbundle(w1649) -> ("[0]"=w1648:cluster{dbl[], dbl[]})  [unwired: 8 out]
            n786 = local read "NumPts 2"() -> (w1644:dbl)
            n787 = Unbundle(w1648) -> (w1647:dbl[], w1646:dbl[])
            n788 = Increment(x=w1645) -> (x+1=w1640:dbl)
            n789 = local write "Index 2"(w1640) -> ()
            n790 = Array Subset(array=w1646, index=w1640, length=w1644) -> (w1635:dbl[])
            n791 = Array Subset(array=w1647, index=w1640, length=w1644) -> (w1636:dbl[])
            n792 = call "STS-Used.vi"("Id Used"=w1636, "Vg-Used"=w1635) -> ("STS"=w1637:dbl)  [unwired: 9 in]
            n793 = Bundle(w1636, w1635) -> (w1642:cluster{dbl[], dbl[]})  [unwired: 1 in]
            n794 = local write "Vg Array-Log-Used"(w1635) -> ()
            n795 = local write "Sat Id-Log-Used"(w1636) -> ()
            n796 = local write "New: STS"(w1637) -> ()
            n797 = Build Array (concatenate)(w1639, w1638, w1642) -> (w1641:cluster{dbl[], dbl[]}[])
            n798 = local write "XY Graph 2"(w1641) -> ()
          }
          event "Previous Button 2": Mouse Down {
            n799 = event-data() -> ()  [unwired: 1 in, 7 out]
            n800 = local read "XY Graph 2"() -> (w1659:cluster{dbl[], dbl[]}[])
            n801 = Decimate 1D Array(w1659) -> (w1656:cluster{dbl[], dbl[]}[], w1655:cluster{dbl[], dbl[]}[])
            n802 = Array To Cluster(array=w1656) -> (cluster=w1664:T9)
            n803 = local read "Index 2"() -> (w1652:dbl)
            n804 = Unbundle(w1664) -> ("[0]"=w1663:cluster{dbl[], dbl[]})  [unwired: 8 out]
            n805 = local read "NumPts 2"() -> (w1660:dbl)
            n806 = Unbundle(w1663) -> (w1662:dbl[], w1661:dbl[])
            n807 = Decrement(x=w1652) -> (x-1=w1653:dbl)
            n808 = local write "Index 2"(w1653) -> ()
            n809 = Array Subset(array=w1662, index=w1653, length=w1660) -> (w1650:dbl[])
            n810 = Array Subset(array=w1661, index=w1653, length=w1660) -> (w1651:dbl[])
            n811 = local write "Vg Array-Log-Used"(w1651) -> ()
            n812 = local write "Sat Id-Log-Used"(w1650) -> ()
            n813 = Bundle(w1650, w1651) -> (w1658:cluster{dbl[], dbl[]})  [unwired: 1 in]
            n814 = call "STS-Used.vi"("Id Used"=w1650, "Vg-Used"=w1651) -> ("STS"=w1654:dbl)  [unwired: 9 in]
            n815 = Build Array (concatenate)(w1656, w1655, w1658) -> (w1657:cluster{dbl[], dbl[]}[])
            n816 = local write "New: STS"(w1654) -> ()
            n817 = local write "XY Graph 2"(w1657) -> ()
          }
          event "Previous Button": Mouse Down {
            n818 = event-data() -> ()  [unwired: 1 in, 5 out]
            n819 = local read "XY Graph"() -> (w1678:cluster{dbl[], dbl[]}[])
            n820 = Decimate 1D Array(w1678) -> (w1675:cluster{dbl[], dbl[]}[], w1674:cluster{dbl[], dbl[]}[])
            n821 = Array To Cluster(array=w1675) -> (cluster=w1683:T9)
            n822 = local read "MobVi Index"() -> (w1673:dbl)
            n823 = Unbundle(w1683) -> ("[0]"=w1682:cluster{dbl[], dbl[]})  [unwired: 8 out]
            n824 = local read "NumPts"() -> (w1679:dbl)
            n825 = Unbundle(w1682) -> (w1681:dbl[], w1680:dbl[])
            n826 = Decrement(x=w1673) -> (x-1=w1672:dbl)
            n827 = local read "New: Dielectric"() -> (w1666:dbl)
            n828 = local read "New: Length"() -> (w1667:dbl)
            n829 = local read "New: Width"() -> (w1668:dbl)
            n830 = local write "MobVi Index"(w1672) -> ()
            n831 = Array Subset(array=w1681, index=w1672, length=w1679) -> (w1671:dbl[])
            n832 = Array Subset(array=w1680, index=w1672, length=w1679) -> (w1670:dbl[])
            n833 = local write "Sat Vg Array-Used"(w1671) -> ()
            n834 = local write "Sat Id-Used"(w1670) -> ()
            n835 = call "Mobility-Vt-Used Pts_Linear.vi"("Width"=w1668, "Length"=w1667, "Dielectric (d)"=w1666, "Sat Id Used"=w1670, "Vg Used"=w1671) -> ("Vt"=w1665:dbl, "Mobility"=w1669:dbl)  [unwired: 4 in, 1 out]
            n836 = Bundle(w1671, w1670) -> (w1677:cluster{dbl[], dbl[]})  [unwired: 1 in]
            n837 = local write "New: VT-Sat"(w1665) -> ()
            n838 = Build Array (concatenate)(w1675, w1674, w1677) -> (w1676:cluster{dbl[], dbl[]}[])
            n839 = local write "New: Mobility-Sat"(w1669) -> ()
            n840 = local write "XY Graph"(w1676) -> ()
          }
          event "Slide": Value Change {
            n841 = event-data() -> ()  [unwired: 1 in, 5 out]
            n842 = local read "XY Graph"() -> (w1696:cluster{dbl[], dbl[]}[])
            n843 = Decimate 1D Array(w1696) -> (w1693:cluster{dbl[], dbl[]}[], w1692:cluster{dbl[], dbl[]}[])
            n844 = Array To Cluster(array=w1693) -> (cluster=w1701:T9)
            n845 = Unbundle(w1701) -> ("[0]"=w1700:cluster{dbl[], dbl[]})  [unwired: 8 out]
            n846 = local read "NumPts"() -> (w1697:dbl)
            n847 = local read "Slide"() -> (w1685:dbl)
            n848 = Unbundle(w1700) -> (w1699:dbl[], w1698:dbl[])
            n849 = local read "New: Dielectric"() -> (w1686:dbl)
            n850 = local read "New: Length"() -> (w1687:dbl)
            n851 = local read "New: Width"() -> (w1688:dbl)
            n852 = local write "MobVi Index"(w1685) -> ()
            n853 = Array Subset(array=w1699, index=w1685, length=w1697) -> (w1691:dbl[])
            n854 = Array Subset(array=w1698, index=w1685, length=w1697) -> (w1690:dbl[])
            n855 = local write "Sat Vg Array-Used"(w1691) -> ()
            n856 = local write "Sat Id-Used"(w1690) -> ()
            n857 = call "Mobility-Vt-Used Pts_Linear.vi"("Width"=w1688, "Length"=w1687, "Dielectric (d)"=w1686, "Sat Id Used"=w1690, "Vg Used"=w1691) -> ("Vt"=w1684:dbl, "Mobility"=w1689:dbl)  [unwired: 4 in, 1 out]
            n858 = Bundle(w1691, w1690) -> (w1695:cluster{dbl[], dbl[]})  [unwired: 1 in]
            n859 = local write "New: VT-Sat"(w1684) -> ()
            n860 = Build Array (concatenate)(w1693, w1692, w1695) -> (w1694:cluster{dbl[], dbl[]}[])
            n861 = local write "New: Mobility-Sat"(w1689) -> ()
            n862 = local write "XY Graph"(w1694) -> ()
          }
          event "Slide 2": Value Change {
            n863 = event-data() -> ()  [unwired: 1 in, 5 out]
            n864 = local read "XY Graph 2"() -> (w1710:cluster{dbl[], dbl[]}[])
            n865 = Decimate 1D Array(w1710) -> (w1707:cluster{dbl[], dbl[]}[], w1706:cluster{dbl[], dbl[]}[])
            n866 = Array To Cluster(array=w1707) -> (cluster=w1715:T9)
            n867 = Unbundle(w1715) -> ("[0]"=w1714:cluster{dbl[], dbl[]})  [unwired: 8 out]
            n868 = local read "NumPts 2"() -> (w1711:dbl)
            n869 = local read "Slide 2"() -> (w1705:dbl)
            n870 = Unbundle(w1714) -> (w1713:dbl[], w1712:dbl[])
            n871 = local write "Index 2"(w1705) -> ()
            n872 = Array Subset(array=w1713, index=w1705, length=w1711) -> (w1703:dbl[])
            n873 = Array Subset(array=w1712, index=w1705, length=w1711) -> (w1702:dbl[])
            n874 = local write "Vg Array-Log-Used"(w1702) -> ()
            n875 = local write "Sat Id-Log-Used"(w1703) -> ()
            n876 = call "STS-Used.vi"("Id Used"=w1703, "Vg-Used"=w1702) -> ("STS"=w1704:dbl)  [unwired: 9 in]
            n877 = Bundle(w1703, w1702) -> (w1709:cluster{dbl[], dbl[]})  [unwired: 1 in]
            n878 = local write "New: STS"(w1704) -> ()
            n879 = Build Array (concatenate)(w1707, w1706, w1709) -> (w1708:cluster{dbl[], dbl[]}[])
            n880 = local write "XY Graph 2"(w1708) -> ()
          }
          event "Save Changes?": Mouse Down {
            n881 = event-data() -> ()  [unwired: 1 in, 5 out]
            n882 = flat-sequence {
              tunnel: [w1743] -> w1720
              tunnel: [w1737] -> w1719
              tunnel: [w1723] -> w1718
              tunnel: w1720 -> [w2024]
              tunnel: w1719 -> [w2021]
              tunnel: [w2022] -> w1717
              tunnel: w1718 -> [w2022]
              tunnel: [w2021] -> w1716
              tunnel: w1717 -> [w2029]
              tunnel: w1716 -> [w2028]
              frame #0 {
                n883 = local read "New: Temp"() -> (w1724:dbl)
                n884 = local read "Data File"() -> (w1743:path)
                n885 = local read "New: Length"() -> (w1728:dbl)
                n886 = local read "New: Width"() -> (w1726:dbl)
                n887 = To Single Precision Float(number=w1724) -> (single precision float=w1725:sgl)
                n888 = call-poly <vilib>:"Read From Spreadsheet File.vi"("file path (dialog if empty)"=w1743) -> ("all rows"=w1721:string[][])  [unwired: 6 in, 4 out]
                n889 = Number To Decimal String(number=w1725) -> (decimal integer string=w1740:string)  [unwired: 1 in]
                n890 = To Single Precision Float(number=w1726) -> (single precision float=w1727:sgl)
                n891 = To Single Precision Float(number=w1728) -> (single precision float=w1729:sgl)
                n892 = local read "Index"() -> (w1746:string)
                n893 = Strip Path(path=w1743) -> (stripped path=w1751:path)  [unwired: 1 out]
                n894 = Number To Decimal String(number=w1729) -> (decimal integer string=w1744:string)  [unwired: 1 in]
                n895 = Number To Decimal String(number=w1727) -> (decimal integer string=w1745:string)  [unwired: 1 in]
                n896 = Array Size(array=w1721) -> (size(s)=w1734:i32[])
                n897 = Concatenate Strings("_", w1740, "K") -> (w1738:string)
                n898 = Array Subset(array=w1721, index (row)=0, index (col)=0, length (col)=3) -> (w1730:string[][])  [unwired: 1 in]
                n899 = Index Array(array=w1734, index=0) -> (element=w1736:i32)
                n900 = call "Build Text"("Temp"=w1738, "Index"=w1746, "Length"=w1744, "Width"=w1745) -> ("Result"=w1747:string)  [unwired: 10 in, 1 out]
                n901 = flat-sequence {
                  tunnel: [w1978] -> w1742
                  tunnel: w1742 -> [w1995]
                  frame #0 {
                    # "Makes Empty File for Transformer Data"
                    n902 = local read "Data Folder"() -> (w1967:path)
                    n903 = Build Path(base path=w1967, name or relative path="Stats") -> (appended path=w1969:path)
                    n904 = call <vilib>:"Check if File or Folder Exists.vi"("path"=w1969) -> ("file or folder exists?"=w1970:bool, "dup path"=w1971:path)  [unwired: 8 in, 1 out]
                    n905 = case shown="False" w1970 {
                      tunnel: [w1975 w1977] -> w1972
                      tunnel: w1971 -> [w1976 w1977]
                      frame False {
                        n906 = Create Folder(path (use dialog)=w1976) -> (created path=w1975:path)  [unwired: 2 in, 2 out]
                      }
                      frame True {
                      }
                    }
                    n907 = Build Path(base path=w1972, name or relative path="Tranformer Data.txt") -> (appended path=w1974:path)
                    n908 = call-poly <vilib>:"Write To Spreadsheet File.vi"("append to file? (new file:F)"=TRUE, "file path (dialog if empty)"=w1974) -> ()  [unwired: 6 in, 1 out]
                  }
                  frame #1 {
                    # "Adds Headers if they don't exist"
                    n909 = Concatenate Strings("Stats\\", "Tranformer Data.txt") -> (w1985:string)
                    n910 = local read "Data Folder"() -> (w1984:path)
                    n911 = Build Path(base path=w1984, name or relative path=w1985) -> (appended path=w1978:path)
                    n912 = call-poly <vilib>:"Read From Spreadsheet File.vi"("file path (dialog if empty)"=w1978) -> ("first row"=w1983:string[])  [unwired: 6 in, 4 out]
                    n913 = Search 1D Array(1D array=w1983, element="DeviceID") -> (index of element=w1981:i32)  [unwired: 1 in]
                    n914 = Equal?(x=w1981, y=0) -> (x = y?=w1979:bool)
                    n915 = case shown="False" w1979 {
                      tunnel: w1978 -> [w1989 _]
                      frame False {
                        n916 = local read "Transformer \nHeaders"() -> (w1988:string[])
                        n917 = call-poly <vilib>:"Write To Spreadsheet File.vi"("1D data"=w1988, "file path (dialog if empty)"=w1989) -> ()  [unwired: 6 in, 1 out]
                      }
                      frame True {
                      }
                    }
                  }
                  frame #2 {
                    # "Adds current device if it doesn't exist"
                    n918 = local read "Current \nRecord"() -> (w1994:string[])
                    n919 = Index Array(array=w1994, index=0) -> (element=w1993:string)
                    n920 = Concatenate Strings("Stats\\", "Tranformer Data.txt") -> (w1998:string)
                    n921 = local read "Data Folder"() -> (w1997:path)
                    n922 = local write "Current Device ID"(w1993) -> ()
                    n923 = local read "Current Device ID"() -> (w2003:string)
                    n924 = Build Path(base path=w1997, name or relative path=w1998) -> (appended path=w1996:path)
                    n925 = call-poly <vilib>:"Read From Spreadsheet File.vi"("file path (dialog if empty)"=w1996) -> ("all rows"=w1990:string[][])  [unwired: 6 in, 4 out]
                    n926 = Index Array(array=w1990, index (col)=0) -> (element=w1991:string[])  [unwired: 1 in]
                    n927 = Search 1D Array(1D array=w1991, element=w2003) -> (index of element=w1992:i32)  [unwired: 1 in]
                    n928 = Equal?(x=w1992, y=-1) -> (x = y?=w2005:bool)
                    n929 = case shown="False" w2005 {
                      tunnel: w1995 -> [w2008 w2019]
                      tunnel: w1992 -> [w2011 _]
                      tunnel: w1990 -> [w2012 _]
                      frame False {
                        n930 = local read "Current \nRecord"() -> (w2010:string[])
                        n931 = Replace Array Subset(array=w2012, new element=w2010, index (row)=w2011) -> (w2009:string[][])  [unwired: 1 in]
                        n932 = flat-sequence {
                          tunnel: w2008 -> [w2013]
                          tunnel: w2009 -> [w2014]
                          tunnel: [w2014] -> w2007
                          tunnel: [w2013] -> w2006
                          tunnel: w2007 -> [w2016]
                          tunnel: w2006 -> [w2015]
                          frame #0 {
                            n933 = Delete(path (use dialog)=w2013) -> ()  [unwired: 4 in, 3 out]
                          }
                          frame #1 {
                            n934 = call-poly <vilib>:"Write To Spreadsheet File.vi"("append to file? (new file:F)"=TRUE, "2D data"=w2016, "file path (dialog if empty)"=w2015) -> ()  [unwired: 5 in, 1 out]
                          }
                        }
                      }
                      frame True {
                        n935 = local read "Current \nRecord"() -> (w2018:string[])
                        n936 = call-poly <vilib>:"Write To Spreadsheet File.vi"("append to file? (new file:F)"=TRUE, "1D data"=w2018, "file path (dialog if empty)"=w2019) -> ()  [unwired: 5 in, 1 out]
                      }
                    }
                  }
                }
                n937 = Reshape Array(w1730, w1736) -> (w1722:string[])
                n938 = Path To String(path=w1751) -> (string=w1749:string)
                n939 = stacked-sequence {
                  tunnel: w1722 -> [w1758 w1771 w1789 w1807 w1825 w1843 w1861 w1879 w1896 w1914 w1932 w1950]
                  tunnel: [_ _ _ _ _ _ _ _ _ _ _ w1948] -> w1723
                  frame #0 {
                    n940 = Search 1D Array(1D array=w1758, element="Dielectric (nm):") -> (index of element=w1755:i32)  [unwired: 1 in]
                    n941 = Equal?(x=w1755, y=-1) -> (x = y?=w1754:bool)
                    n942 = local read "Save1 Array"() -> (w1753:string[][])
                    n943 = case shown="False" w1754 {
                      tunnel: w1753 -> [w1764 w1768]
                      tunnel: w1755 -> [w1760 _]
                      tunnel: [w1759 w1768] -> w1752
                      frame False {
                        n944 = local read "New: Dielectric"() -> (w1766:dbl)
                        n945 = Number To Fractional String(number=w1766) -> (F-format string=w1761:string)  [unwired: 3 in]
                        n946 = Divide(x=w1760, y=3) -> (x/y=w1763:dbl)
                        n947 = To Word Integer(number=w1763) -> (16bit integer=w1762:i16)
                        n948 = Replace Array Subset(array=w1764, new element=w1761, index (row)=w1762, index (col)=1) -> (w1759:string[][])
                      }
                      frame True {
                      }
                    }
                    n949 = local write "Save1 Array"(w1752) -> ()
                  }
                  frame #1 {
                    n950 = Search 1D Array(1D array=w1771, element="Length (um):") -> (index of element=w1773:i32)  [unwired: 1 in]
                    n951 = Equal?(x=w1773, y=-1) -> (x = y?=w1772:bool)
                    n952 = local read "Save1 Array"() -> (w1770:string[][])
                    n953 = case shown="False" w1772 {
                      tunnel: w1770 -> [w1783 w1786]
                      tunnel: w1773 -> [w1780 _]
                      tunnel: [w1779 w1786] -> w1769
                      frame False {
                        n954 = local read "New: Length"() -> (w1776:dbl)
                        n955 = Divide(x=w1780, y=3) -> (x/y=w1782:dbl)
                        n956 = Format Value(format string="%#g", value (0)=w1776) -> (output string=w1777:string)  [unwired: 1 in]
                        n957 = To Word Integer(number=w1782) -> (16bit integer=w1781:i16)
                        n958 = Replace Array Subset(array=w1783, new element=w1777, index (row)=w1781, index (col)=1) -> (w1779:string[][])
                      }
                      frame True {
                      }
                    }
                    n959 = local write "Save1 Array"(w1769) -> ()
                  }
                  frame #2 {
                    n960 = Search 1D Array(1D array=w1789, element="Width (um):") -> (index of element=w1791:i32)  [unwired: 1 in]
                    n961 = Equal?(x=w1791, y=-1) -> (x = y?=w1790:bool)
                    n962 = local read "Save1 Array"() -> (w1788:string[][])
                    n963 = case shown="False" w1790 {
                      tunnel: w1791 -> [w1799 _]
                      tunnel: w1788 -> [w1798 w1804]
                      tunnel: [w1797 w1804] -> w1787
                      frame False {
                        n964 = local read "New: Width"() -> (w1794:dbl)
                        n965 = Divide(x=w1799, y=3) -> (x/y=w1801:dbl)
                        n966 = To Word Integer(number=w1801) -> (16bit integer=w1800:i16)
                        n967 = Format Value(format string="%#g", value (0)=w1794) -> (output string=w1795:string)  [unwired: 1 in]
                        n968 = Replace Array Subset(array=w1798, new element=w1795, index (row)=w1800, index (col)=1) -> (w1797:string[][])
                      }
                      frame True {
                      }
                    }
                    n969 = local write "Save1 Array"(w1787) -> ()
                  }
                  frame #3 {
                    n970 = Search 1D Array(1D array=w1807, element="Sample Temp (K):") -> (index of element=w1809:i32)  [unwired: 1 in]
                    n971 = Equal?(x=w1809, y=-1) -> (x = y?=w1808:bool)
                    n972 = local read "Save1 Array"() -> (w1806:string[][])
                    n973 = case shown="False" w1808 {
                      tunnel: w1806 -> [w1819 w1822]
                      tunnel: w1809 -> [w1816 _]
                      tunnel: [w1815 w1822] -> w1805
                      frame False {
                        n974 = local read "New: Temp"() -> (w1813:dbl)
                        n975 = Divide(x=w1816, y=3) -> (x/y=w1818:dbl)
                        n976 = Format Value(format string="%#g", value (0)=w1813) -> (output string=w1812:string)  [unwired: 1 in]
                        n977 = To Word Integer(number=w1818) -> (16bit integer=w1817:i16)
                        n978 = Replace Array Subset(array=w1819, new element=w1812, index (row)=w1817, index (col)=1) -> (w1815:string[][])
                      }
                      frame True {
                      }
                    }
                    n979 = local write "Save1 Array"(w1805) -> ()
                  }
                  frame #4 {
                    n980 = Search 1D Array(1D array=w1825, element="Mobility-Sat (cm^2/Vs):") -> (index of element=w1827:i32)  [unwired: 1 in]
                    n981 = Equal?(x=w1827, y=-1) -> (x = y?=w1826:bool)
                    n982 = local read "Save1 Array"() -> (w1823:string[][])
                    n983 = case shown="False" w1826 {
                      tunnel: w1823 -> [w1837 w1840]
                      tunnel: w1827 -> [w1834 _]
                      tunnel: [w1833 w1840] -> w1824
                      frame False {
                        n984 = local read "New: Mobility-Sat"() -> (w1830:dbl)
                        n985 = Divide(x=w1834, y=3) -> (x/y=w1836:dbl)
                        n986 = To Word Integer(number=w1836) -> (16bit integer=w1835:i16)
                        n987 = Format Value(format string="%#g", value (0)=w1830) -> (output string=w1831:string)  [unwired: 1 in]
                        n988 = Replace Array Subset(array=w1837, new element=w1831, index (row)=w1835, index (col)=1) -> (w1833:string[][])
                      }
                      frame True {
                      }
                    }
                    n989 = local write "Save1 Array"(w1824) -> ()
                  }
                  frame #5 {
                    n990 = Search 1D Array(1D array=w1843, element="Mobility-Lin (cm^2/Vs):") -> (index of element=w1845:i32)  [unwired: 1 in]
                    n991 = Equal?(x=w1845, y=-1) -> (x = y?=w1844:bool)
                    n992 = local read "Save1 Array"() -> (w1842:string[][])
                    n993 = case shown="False" w1844 {
                      tunnel: w1842 -> [w1855 w1858]
                      tunnel: w1845 -> [w1852 _]
                      tunnel: [w1851 w1858] -> w1841
                      frame False {
                        n994 = local read "New: Mobility-Lin"() -> (w1848:dbl)
                        n995 = Divide(x=w1852, y=3) -> (x/y=w1854:dbl)
                        n996 = To Word Integer(number=w1854) -> (16bit integer=w1853:i16)
                        n997 = Format Value(format string="%#g", value (0)=w1848) -> (output string=w1849:string)  [unwired: 1 in]
                        n998 = Replace Array Subset(array=w1855, new element=w1849, index (row)=w1853, index (col)=1) -> (w1851:string[][])
                      }
                      frame True {
                      }
                    }
                    n999 = local write "Save1 Array"(w1841) -> ()
                  }
                  frame #6 {
                    n1000 = Search 1D Array(1D array=w1861, element="Off I-Sat (A):") -> (index of element=w1863:i32)  [unwired: 1 in]
                    n1001 = Equal?(x=w1863, y=-1) -> (x = y?=w1862:bool)
                    n1002 = local read "Save1 Array"() -> (w1860:string[][])
                    n1003 = case shown="False" w1862 {
                      tunnel: w1860 -> [w1873 w1876]
                      tunnel: w1863 -> [w1870 _]
                      tunnel: [w1869 w1876] -> w1859
                      frame False {
                        n1004 = local read "Calc: Off I-Sat"() -> (w1868:dbl)
                        n1005 = Divide(x=w1870, y=3) -> (x/y=w1872:dbl)
                        n1006 = Format Value(format string="%#g", value (0)=w1868) -> (output string=w1866:string)  [unwired: 1 in]
                        n1007 = To Word Integer(number=w1872) -> (16bit integer=w1871:i16)
                        n1008 = Replace Array Subset(array=w1873, new element=w1866, index (row)=w1871, index (col)=1) -> (w1869:string[][])
                      }
                      frame True {
                      }
                    }
                    n1009 = local write "Save1 Array"(w1859) -> ()
                  }
                  frame #7 {
                    n1010 = Search 1D Array(1D array=w1879, element="Vt-Sat (V):") -> (index of element=w1881:i32)  [unwired: 1 in]
                    n1011 = Equal?(x=w1881, y=-1) -> (x = y?=w1880:bool)
                    n1012 = local read "Save1 Array"() -> (w1878:string[][])
                    n1013 = case shown="False" w1880 {
                      tunnel: w1878 -> [w1889 w1893]
                      tunnel: w1881 -> [w1885 _]
                      tunnel: [w1884 w1893] -> w1877
                      frame False {
                        n1014 = local read "New: VT-Sat"() -> (w1891:dbl)
                        n1015 = Number To Fractional String(number=w1891) -> (F-format string=w1886:string)  [unwired: 3 in]
                        n1016 = Divide(x=w1885, y=3) -> (x/y=w1888:dbl)
                        n1017 = To Word Integer(number=w1888) -> (16bit integer=w1887:i16)
                        n1018 = Replace Array Subset(array=w1889, new element=w1886, index (row)=w1887, index (col)=1) -> (w1884:string[][])
                      }
                      frame True {
                      }
                    }
                    n1019 = local write "Save1 Array"(w1877) -> ()
                  }
                  frame #8 {
                    n1020 = Search 1D Array(1D array=w1896, element="VT-Lin (V):") -> (index of element=w1898:i32)  [unwired: 1 in]
                    n1021 = Equal?(x=w1898, y=-1) -> (x = y?=w1897:bool)
                    n1022 = local read "Save1 Array"() -> (w1895:string[][])
                    n1023 = case shown="False" w1897 {
                      tunnel: w1895 -> [w1908 w1911]
                      tunnel: w1898 -> [w1905 _]
                      tunnel: [w1904 w1911] -> w1894
                      frame False {
                        n1024 = local read "New: VT-Lin"() -> (w1902:dbl)
                        n1025 = Divide(x=w1905, y=3) -> (x/y=w1907:dbl)
                        n1026 = Format Value(format string="%#g", value (0)=w1902) -> (output string=w1901:string)  [unwired: 1 in]
                        n1027 = To Word Integer(number=w1907) -> (16bit integer=w1906:i16)
                        n1028 = Replace Array Subset(array=w1908, new element=w1901, index (row)=w1906, index (col)=1) -> (w1904:string[][])
                      }
                      frame True {
                      }
                    }
                    n1029 = local write "Save1 Array"(w1894) -> ()
                  }
                  frame #9 {
                    n1030 = Search 1D Array(1D array=w1914, element="STS-Sat (V/decade):") -> (index of element=w1916:i32)  [unwired: 1 in]
                    n1031 = Equal?(x=w1916, y=-1) -> (x = y?=w1915:bool)
                    n1032 = local read "Save1 Array"() -> (w1913:string[][])
                    n1033 = case shown="False" w1915 {
                      tunnel: w1913 -> [w1926 w1929]
                      tunnel: w1916 -> [w1923 _]
                      tunnel: [w1922 w1929] -> w1912
                      frame False {
                        n1034 = local read "New: STS"() -> (w1920:dbl)
                        n1035 = Divide(x=w1923, y=3) -> (x/y=w1925:dbl)
                        n1036 = Format Value(format string="%#g", value (0)=w1920) -> (output string=w1919:string)  [unwired: 1 in]
                        n1037 = To Word Integer(number=w1925) -> (16bit integer=w1924:i16)
                        n1038 = Replace Array Subset(array=w1926, new element=w1919, index (row)=w1924, index (col)=1) -> (w1922:string[][])
                      }
                      frame True {
                      }
                    }
                    n1039 = local write "Save1 Array"(w1912) -> ()
                  }
                  frame #10 {
                    n1040 = Search 1D Array(1D array=w1932, element="Trap Density-VT (Traps/Vcm^2):") -> (index of element=w1934:i32)  [unwired: 1 in]
                    n1041 = Equal?(x=w1934, y=-1) -> (x = y?=w1933:bool)
                    n1042 = local read "Save1 Array"() -> (w1931:string[][])
                    n1043 = case shown="False" w1933 {
                      tunnel: w1931 -> [w1944 w1947]
                      tunnel: w1934 -> [w1940 _]
                      tunnel: [w1939 w1947] -> w1930
                      frame False {
                        n1044 = local read "New: Trap Density-VT"() -> (w1938:dbl)
                        n1045 = Format Value(format string="%#g", value (0)=w1938) -> (output string=w1941:string)  [unwired: 1 in]
                        n1046 = Divide(x=w1940, y=3) -> (x/y=w1943:dbl)
                        n1047 = To Word Integer(number=w1943) -> (16bit integer=w1942:i16)
                        n1048 = Replace Array Subset(array=w1944, new element=w1941, index (row)=w1942, index (col)=1) -> (w1939:string[][])
                      }
                      frame True {
                      }
                    }
                    n1049 = local write "Save1 Array"(w1930) -> ()
                  }
                  frame #11 {
                    n1050 = Search 1D Array(1D array=w1950, element="Trap Density-STS (Traps/Vcm^2):") -> (index of element=w1952:i32)  [unwired: 1 in]
                    n1051 = Equal?(x=w1952, y=-1) -> (x = y?=w1951:bool)
                    n1052 = local read "Save1 Array"() -> (w1949:string[][])
                    n1053 = case shown="False" w1951 {
                      tunnel: w1949 -> [w1962 w1965]
                      tunnel: w1952 -> [w1959 _]
                      tunnel: [w1958 w1965] -> w1948
                      frame False {
                        n1054 = local read "New: Trap Density-STS"() -> (w1956:dbl)
                        n1055 = Divide(x=w1959, y=3) -> (x/y=w1961:dbl)
                        n1056 = To Word Integer(number=w1961) -> (16bit integer=w1960:i16)
                        n1057 = Format Value(format string="%#g", value (0)=w1956) -> (output string=w1955:string)  [unwired: 1 in]
                        n1058 = Replace Array Subset(array=w1962, new element=w1955, index (row)=w1960, index (col)=1) -> (w1958:string[][])
                      }
                      frame True {
                      }
                    }
                    n1059 = local write "Save1 Array"(w1948) -> ()
                  }
                }
                n1060 = Concatenate Strings(w1749, "\\", w1747) -> (w1748:string)
                n1061 = String To Path(string=w1748) -> (path=w1737:path)
                n1062 = local write "Save1 Array"(w1721) -> ()
              }
              frame #1 {
                n1063 = Equal?(x=w2024, y=w2021) -> (x = y?=w2023:bool)
                n1064 = case shown="False" w2023 {
                  tunnel: w2024 -> [w2027 _]
                  tunnel: w2021 -> [w2026 _]
                  frame False {
                    n1065 = Move(source path=w2027, 9:TRUE, 10:w2026) -> ()  [unwired: 2 in, 3 out]
                  }
                  frame True {
                  }
                }
              }
              frame #2 {
                n1066 = local write "Data File"(w2028) -> ()
                n1067 = call-poly <vilib>:"Write To Spreadsheet File.vi"("2D data"=w2029, "file path (dialog if empty)"=w2028) -> ()  [unwired: 6 in, 1 out]
              }
            }
          }
          event "Save Changes? 2": Mouse Down {
            n1068 = event-data() -> ()  [unwired: 1 in, 5 out]
            n1069 = stacked-sequence {
              seq-local: [w2089 _ _ _ _] -> [_ w2324 _ _ _]
              seq-local: [w2092 _ _ _ _] -> [_ w2325 _ _ _]
              seq-local: [w2089 _ _ _ _] -> [_ w2323 _ _ _]
              seq-local: [w2087 _ _ _ _] -> [_ w2321 _ _ _]
              seq-local: [_ w2325 _ _ _] -> [_ _ w2330 _ _]
              seq-local: [_ w2321 _ _ _] -> [_ _ w2329 _ _]
              frame #0 {
                n1070 = local read "New: Temp"() -> (w2091:dbl)
                n1071 = local read "Data File"() -> (w2092:path)
                n1072 = local read "New: Length"() -> (w2095:dbl)
                n1073 = local read "New: Width"() -> (w2093:dbl)
                n1074 = To Word Integer(number=w2091) -> (16bit integer=w2090:i16)
                n1075 = call-poly <vilib>:"Read From Spreadsheet File.vi"("file path (dialog if empty)"=w2092) -> ("all rows"=w2086:string[][])  [unwired: 6 in, 4 out]
                n1076 = Number To Decimal String(number=w2090) -> (decimal integer string=w2106:string)  [unwired: 1 in]
                n1077 = To Single Precision Float(number=w2093) -> (single precision float=w2094:sgl)
                n1078 = To Single Precision Float(number=w2095) -> (single precision float=w2096:sgl)
                n1079 = local read "Index"() -> (w2110:string)
                n1080 = Strip Path(path=w2092) -> (stripped path=w2115:path)  [unwired: 1 out]
                n1081 = Number To Decimal String(number=w2096) -> (decimal integer string=w2108:string)  [unwired: 1 in]
                n1082 = Number To Decimal String(number=w2094) -> (decimal integer string=w2109:string)  [unwired: 1 in]
                n1083 = Array Size(array=w2086) -> (size(s)=w2101:i32[])
                n1084 = Concatenate Strings("_", w2106, "K") -> (w2104:string)
                n1085 = Array Subset(array=w2086, index (row)=0, index (col)=0, length (col)=3) -> (w2097:string[][])  [unwired: 1 in]
                n1086 = Index Array(array=w2101, index=0) -> (element=w2103:i32)
                n1087 = call "Build Text2"("Temp"=w2104, "Index"=w2110, "Length"=w2108, "Width"=w2109) -> ("Result"=w2111:string)  [unwired: 10 in, 1 out]
                n1088 = Reshape Array(w2097, w2103) -> (w2088:string[])
                n1089 = Path To String(path=w2115) -> (string=w2113:string)
                n1090 = stacked-sequence {
                  tunnel: w2088 -> [w2122 w2135 w2152 w2169 w2186 w2203 w2220 w2238 w2255 w2272 w2289 w2306]
                  tunnel: [_ _ _ _ _ _ _ _ _ _ _ w2304] -> w2087
                  frame #0 {
                    n1091 = Search 1D Array(1D array=w2122, element="Dielectric (nm):") -> (index of element=w2119:i32)  [unwired: 1 in]
                    n1092 = Equal?(x=w2119, y=-1) -> (x = y?=w2118:bool)
                    n1093 = local read "Save1 Array"() -> (w2117:string[][])
                    n1094 = case shown="False" w2118 {
                      tunnel: w2117 -> [w2128 w2132]
                      tunnel: w2119 -> [w2124 _]
                      tunnel: [w2123 w2132] -> w2116
                      frame False {
                        n1095 = local read "New: Dielectric"() -> (w2130:dbl)
                        n1096 = Number To Fractional String(number=w2130) -> (F-format string=w2125:string)  [unwired: 3 in]
                        n1097 = Divide(x=w2124, y=3) -> (x/y=w2127:dbl)
                        n1098 = To Word Integer(number=w2127) -> (16bit integer=w2126:i16)
                        n1099 = Replace Array Subset(array=w2128, new element=w2125, index (row)=w2126, index (col)=1) -> (w2123:string[][])
                      }
                      frame True {
                      }
                    }
                    n1100 = local write "Save1 Array"(w2116) -> ()
                  }
                  frame #1 {
                    n1101 = Search 1D Array(1D array=w2135, element="Length (um):") -> (index of element=w2137:i32)  [unwired: 1 in]
                    n1102 = Equal?(x=w2137, y=-1) -> (x = y?=w2136:bool)
                    n1103 = local read "Save1 Array"() -> (w2134:string[][])
                    n1104 = case shown="True" w2136 {
                      tunnel: w2134 -> [w2145 w2149]
                      tunnel: w2137 -> [w2141 _]
                      tunnel: [w2140 w2149] -> w2133
                      frame False {
                        n1105 = local read "New: Length"() -> (w2147:dbl)
                        n1106 = Number To Fractional String(number=w2147) -> (F-format string=w2142:string)  [unwired: 3 in]
                        n1107 = Divide(x=w2141, y=3) -> (x/y=w2144:dbl)
                        n1108 = To Word Integer(number=w2144) -> (16bit integer=w2143:i16)
                        n1109 = Replace Array Subset(array=w2145, new element=w2142, index (row)=w2143, index (col)=1) -> (w2140:string[][])
                      }
                      frame True {
                      }
                    }
                    n1110 = local write "Save1 Array"(w2133) -> ()
                  }
                  frame #2 {
                    n1111 = Search 1D Array(1D array=w2152, element="Width (um):") -> (index of element=w2154:i32)  [unwired: 1 in]
                    n1112 = Equal?(x=w2154, y=-1) -> (x = y?=w2153:bool)
                    n1113 = local read "Save1 Array"() -> (w2151:string[][])
                    n1114 = case shown="False" w2153 {
                      tunnel: w2154 -> [w2159 _]
                      tunnel: w2151 -> [w2158 w2166]
                      tunnel: [w2157 w2166] -> w2150
                      frame False {
                        n1115 = local read "New: Width"() -> (w2164:dbl)
                        n1116 = Number To Fractional String(number=w2164) -> (F-format string=w2160:string)  [unwired: 3 in]
                        n1117 = Divide(x=w2159, y=3) -> (x/y=w2162:dbl)
                        n1118 = To Word Integer(number=w2162) -> (16bit integer=w2161:i16)
                        n1119 = Replace Array Subset(array=w2158, new element=w2160, index (row)=w2161, index (col)=1) -> (w2157:string[][])
                      }
                      frame True {
                      }
                    }
                    n1120 = local write "Save1 Array"(w2150) -> ()
                  }
                  frame #3 {
                    n1121 = Search 1D Array(1D array=w2169, element="Sample Temp (K):") -> (index of element=w2171:i32)  [unwired: 1 in]
                    n1122 = Equal?(x=w2171, y=-1) -> (x = y?=w2170:bool)
                    n1123 = local read "Save1 Array"() -> (w2168:string[][])
                    n1124 = case shown="False" w2170 {
                      tunnel: w2168 -> [w2179 w2183]
                      tunnel: w2171 -> [w2175 _]
                      tunnel: [w2174 w2183] -> w2167
                      frame False {
                        n1125 = local read "New: Temp"() -> (w2181:dbl)
                        n1126 = Number To Fractional String(number=w2181) -> (F-format string=w2176:string)  [unwired: 3 in]
                        n1127 = Divide(x=w2175, y=3) -> (x/y=w2178:dbl)
                        n1128 = To Word Integer(number=w2178) -> (16bit integer=w2177:i16)
                        n1129 = Replace Array Subset(array=w2179, new element=w2176, index (row)=w2177, index (col)=1) -> (w2174:string[][])
                      }
                      frame True {
                      }
                    }
                    n1130 = local write "Save1 Array"(w2167) -> ()
                  }
                  frame #4 {
                    n1131 = Search 1D Array(1D array=w2186, element="Mobility-Sat (cm^2/Vs):") -> (index of element=w2188:i32)  [unwired: 1 in]
                    n1132 = Equal?(x=w2188, y=-1) -> (x = y?=w2187:bool)
                    n1133 = local read "Save1 Array"() -> (w2184:string[][])
                    n1134 = case shown="False" w2187 {
                      tunnel: w2184 -> [w2196 w2200]
                      tunnel: w2188 -> [w2192 _]
                      tunnel: [w2191 w2200] -> w2185
                      frame False {
                        n1135 = local read "New: Mobility-Sat"() -> (w2198:dbl)
                        n1136 = Number To Fractional String(number=w2198) -> (F-format string=w2193:string)  [unwired: 3 in]
                        n1137 = Divide(x=w2192, y=3) -> (x/y=w2195:dbl)
                        n1138 = To Word Integer(number=w2195) -> (16bit integer=w2194:i16)
                        n1139 = Replace Array Subset(array=w2196, new element=w2193, index (row)=w2194, index (col)=1) -> (w2191:string[][])
                      }
                      frame True {
                      }
                    }
                    n1140 = local write "Save1 Array"(w2185) -> ()
                  }
                  frame #5 {
                    n1141 = Search 1D Array(1D array=w2203, element="Mobility-Lin (cm^2/Vs):") -> (index of element=w2205:i32)  [unwired: 1 in]
                    n1142 = Equal?(x=w2205, y=-1) -> (x = y?=w2204:bool)
                    n1143 = local read "Save1 Array"() -> (w2202:string[][])
                    n1144 = case shown="False" w2204 {
                      tunnel: w2202 -> [w2213 w2217]
                      tunnel: w2205 -> [w2209 _]
                      tunnel: [w2208 w2217] -> w2201
                      frame False {
                        n1145 = local read "New: Mobility-Lin"() -> (w2215:dbl)
                        n1146 = Number To Fractional String(number=w2215) -> (F-format string=w2210:string)  [unwired: 3 in]
                        n1147 = Divide(x=w2209, y=3) -> (x/y=w2212:dbl)
                        n1148 = To Word Integer(number=w2212) -> (16bit integer=w2211:i16)
                        n1149 = Replace Array Subset(array=w2213, new element=w2210, index (row)=w2211, index (col)=1) -> (w2208:string[][])
                      }
                      frame True {
                      }
                    }
                    n1150 = local write "Save1 Array"(w2201) -> ()
                  }
                  frame #6 {
                    n1151 = Search 1D Array(1D array=w2220, element="Off I-Sat (A):") -> (index of element=w2222:i32)  [unwired: 1 in]
                    n1152 = Equal?(x=w2222, y=-1) -> (x = y?=w2221:bool)
                    n1153 = local read "Save1 Array"() -> (w2219:string[][])
                    n1154 = case shown="False" w2221 {
                      tunnel: w2219 -> [w2232 w2235]
                      tunnel: w2222 -> [w2229 _]
                      tunnel: [w2228 w2235] -> w2218
                      frame False {
                        n1155 = local read "Calc: Off I-Sat"() -> (w2227:dbl)
                        n1156 = Format Value(format string="%#g", value (0)=w2227) -> (output string=w2226:string)  [unwired: 1 in]
                        n1157 = Divide(x=w2229, y=3) -> (x/y=w2231:dbl)
                        n1158 = To Word Integer(number=w2231) -> (16bit integer=w2230:i16)
                        n1159 = Replace Array Subset(array=w2232, new element=w2226, index (row)=w2230, index (col)=1) -> (w2228:string[][])
                      }
                      frame True {
                      }
                    }
                    n1160 = local write "Save1 Array"(w2218) -> ()
                  }
                  frame #7 {
                    n1161 = Search 1D Array(1D array=w2238, element="Vt-Sat (V):") -> (index of element=w2240:i32)  [unwired: 1 in]
                    n1162 = Equal?(x=w2240, y=-1) -> (x = y?=w2239:bool)
                    n1163 = local read "Save1 Array"() -> (w2237:string[][])
                    n1164 = case shown="False" w2239 {
                      tunnel: w2237 -> [w2248 w2252]
                      tunnel: w2240 -> [w2244 _]
                      tunnel: [w2243 w2252] -> w2236
                      frame False {
                        n1165 = local read "New: VT-Sat"() -> (w2250:dbl)
                        n1166 = Number To Fractional String(number=w2250) -> (F-format string=w2245:string)  [unwired: 3 in]
                        n1167 = Divide(x=w2244, y=3) -> (x/y=w2247:dbl)
                        n1168 = To Word Integer(number=w2247) -> (16bit integer=w2246:i16)
                        n1169 = Replace Array Subset(array=w2248, new element=w2245, index (row)=w2246, index (col)=1) -> (w2243:string[][])
                      }
                      frame True {
                      }
                    }
                    n1170 = local write "Save1 Array"(w2236) -> ()
                  }
                  frame #8 {
                    n1171 = Search 1D Array(1D array=w2255, element="VT-Lin (V):") -> (index of element=w2257:i32)  [unwired: 1 in]
                    n1172 = Equal?(x=w2257, y=-1) -> (x = y?=w2256:bool)
                    n1173 = local read "Save1 Array"() -> (w2254:string[][])
                    n1174 = case shown="True" w2256 {
                      tunnel: w2254 -> [w2265 w2269]
                      tunnel: w2257 -> [w2261 _]
                      tunnel: [w2260 w2269] -> w2253
                      frame False {
                        n1175 = local read "New: VT-Lin"() -> (w2267:dbl)
                        n1176 = Number To Fractional String(number=w2267) -> (F-format string=w2262:string)  [unwired: 3 in]
                        n1177 = Divide(x=w2261, y=3) -> (x/y=w2264:dbl)
                        n1178 = To Word Integer(number=w2264) -> (16bit integer=w2263:i16)
                        n1179 = Replace Array Subset(array=w2265, new element=w2262, index (row)=w2263, index (col)=1) -> (w2260:string[][])
                      }
                      frame True {
                      }
                    }
                    n1180 = local write "Save1 Array"(w2253) -> ()
                  }
                  frame #9 {
                    n1181 = Search 1D Array(1D array=w2272, element="STS-Sat (V/decade):") -> (index of element=w2274:i32)  [unwired: 1 in]
                    n1182 = Equal?(x=w2274, y=-1) -> (x = y?=w2273:bool)
                    n1183 = local read "Save1 Array"() -> (w2271:string[][])
                    n1184 = case shown="False" w2273 {
                      tunnel: w2271 -> [w2282 w2286]
                      tunnel: w2274 -> [w2278 _]
                      tunnel: [w2277 w2286] -> w2270
                      frame False {
                        n1185 = local read "New: STS"() -> (w2284:dbl)
                        n1186 = Number To Fractional String(number=w2284) -> (F-format string=w2279:string)  [unwired: 3 in]
                        n1187 = Divide(x=w2278, y=3) -> (x/y=w2281:dbl)
                        n1188 = To Word Integer(number=w2281) -> (16bit integer=w2280:i16)
                        n1189 = Replace Array Subset(array=w2282, new element=w2279, index (row)=w2280, index (col)=1) -> (w2277:string[][])
                      }
                      frame True {
                      }
                    }
                    n1190 = local write "Save1 Array"(w2270) -> ()
                  }
                  frame #10 {
                    n1191 = Search 1D Array(1D array=w2289, element="Trap Density-VT (Traps/Vcm^2):") -> (index of element=w2291:i32)  [unwired: 1 in]
                    n1192 = Equal?(x=w2291, y=-1) -> (x = y?=w2290:bool)
                    n1193 = local read "Save1 Array"() -> (w2288:string[][])
                    n1194 = case shown="False" w2290 {
                      tunnel: w2288 -> [w2299 w2303]
                      tunnel: w2291 -> [w2295 _]
                      tunnel: [w2294 w2303] -> w2287
                      frame False {
                        n1195 = local read "New: Trap Density-VT"() -> (w2301:dbl)
                        n1196 = Number To Fractional String(number=w2301) -> (F-format string=w2296:string)  [unwired: 3 in]
                        n1197 = Divide(x=w2295, y=3) -> (x/y=w2298:dbl)
                        n1198 = To Word Integer(number=w2298) -> (16bit integer=w2297:i16)
                        n1199 = Replace Array Subset(array=w2299, new element=w2296, index (row)=w2297, index (col)=1) -> (w2294:string[][])
                      }
                      frame True {
                      }
                    }
                    n1200 = local write "Save1 Array"(w2287) -> ()
                  }
                  frame #11 {
                    n1201 = Search 1D Array(1D array=w2306, element="Trap Density-STS (Traps/Vcm^2):") -> (index of element=w2308:i32)  [unwired: 1 in]
                    n1202 = Equal?(x=w2308, y=-1) -> (x = y?=w2307:bool)
                    n1203 = local read "Save1 Array"() -> (w2305:string[][])
                    n1204 = case shown="False" w2307 {
                      tunnel: w2305 -> [w2316 w2320]
                      tunnel: w2308 -> [w2312 _]
                      tunnel: [w2311 w2320] -> w2304
                      frame False {
                        n1205 = local read "New: Trap Density-STS"() -> (w2318:dbl)
                        n1206 = Number To Fractional String(number=w2318) -> (F-format string=w2313:string)  [unwired: 3 in]
                        n1207 = Divide(x=w2312, y=3) -> (x/y=w2315:dbl)
                        n1208 = To Word Integer(number=w2315) -> (16bit integer=w2314:i16)
                        n1209 = Replace Array Subset(array=w2316, new element=w2313, index (row)=w2314, index (col)=1) -> (w2311:string[][])
                      }
                      frame True {
                      }
                    }
                    n1210 = local write "Save1 Array"(w2304) -> ()
                  }
                }
                n1211 = Concatenate Strings(w2113, "\\", w2111) -> (w2112:string)
                n1212 = String To Path(string=w2112) -> (path=w2089:path)
                "No Image 2" <- w2089
                n1213 = local write "Save1 Array"(w2086) -> ()
              }
              frame #1 {
                n1214 = Equal?(x=w2324, y=w2323) -> (x = y?=w2322:bool)
                n1215 = case shown="False" w2322 {
                  tunnel: w2324 -> [w2328 _]
                  tunnel: w2323 -> [w2327 _]
                  frame False {
                    n1216 = Move(source path=w2328, 9:TRUE, 10:w2327) -> ()  [unwired: 2 in, 3 out]
                  }
                  frame True {
                  }
                }
              }
              frame #2 {
                n1217 = local write "Data File"(w2330) -> ()
                n1218 = call-poly <vilib>:"Write To Spreadsheet File.vi"("2D data"=w2329, "file path (dialog if empty)"=w2330) -> ()  [unwired: 6 in, 1 out]
              }
              frame #3 {
                w2428 = 0
                # "Moves to next file and displays new image/data"
                n1219 = property on="Image Out" class="ImageControl"() -> (error out=w2390:errorcluster, "Image Center Position"=w2394:cluster{"X":u32, "Y":u32})  [unwired: 2 in, 1 out]
                n1220 = local read "Data File"() -> (w2433:path)
                n1221 = Strip Path(path=w2433) -> (stripped path=w2424:path, name=w2442:string)
                n1222 = Unbundle(w2394) -> ("X"=w2392:u32)  [unwired: 1 out]
                n1223 = local write "Data Folder"(w2424) -> ()
                n1224 = Bundle("X"=w2392, 0) -> (w2393:cluster{"X":u32, i32})  [unwired: 1 in]
                n1225 = property on="Image Out" class="ImageControl"(error in=w2390, "Image Center Position"=w2393) -> ()  [unwired: 1 in, 2 out]
                n1226 = List Folder(path=w2424) -> (filenames=w2438:string[])  [unwired: 3 in, 3 out]
                n1227 = Search 1D Array(1D array=w2438, element=w2442) -> (index of element=w2435:i32)  [unwired: 1 in]
                n1228 = Array Size(array=w2438) -> (size(s)=w2434:i32)
                n1229 = Decrement(x=w2434) -> (x-1=w2436:i32)
                n1230 = Equal?(x=w2435, y=w2436) -> (x = y?=w2437:bool)
                n1231 = local read "Folder Index"() -> (w2386:dbl)
                n1232 = case shown="False" w2437 {
                  tunnel: w2386 -> [w2567 _]
                  tunnel: [w2566 0] -> w2385
                  frame False {
                    n1233 = Increment(x=w2567) -> (x+1=w2566:dbl)
                  }
                  frame True {
                  }
                }
                n1234 = invoke on="Image Out" class="ImageControl" method="Clear ROI"() -> ()  [unwired: 3 in, 3 out]
                n1235 = local write "Folder Index"(w2385) -> ()
                n1236 = Path To String(path=w2424) -> (string=w2443:string)
                n1237 = Index Array(array=w2438, index=w2385) -> (element=w2439:string)
                n1238 = local write "Data Name:"(w2439) -> ()
                n1239 = Concatenate Strings(w2443, "\\", w2439) -> (w2441:string)
                n1240 = String To Path(string=w2441) -> (path=w2336:path)
                n1241 = call "Recorded Values.vi"("Path"=w2336) -> ("Recorded Char"=w2338:T5, "Recorded Prop"=w2339:T6, "Fabrication Prop"=w2337:T7)  [unwired: 8 in]
                n1242 = Unbundle By Name(w2338) -> ("Mobility-Sat"=w2351:dbl, "Moblitity-Lin"=w2352:dbl, "On/Off"=w2353:dbl, "Off Current"=w2354:dbl, "STS"=w2355:dbl, "Trap Density-VT"=w2356:dbl, "Trap Density-STS"=w2357:dbl)  [unwired: 1 out]
                n1243 = Unbundle By Name(w2339) -> ("Date Recorded"=w2347:string, "Index"=w2348:string, "Length"=w2349:dbl, "Width"=w2350:dbl, "Sample Temp"=w2333:dbl)
                n1244 = Unbundle By Name(w2337) -> ("Date Created"=w2358:string, "Material"=w2340:string, "Solvent"=w2341:string, "Concentration"=w2342:dbl, "Method"=w2343:string, "Dielectric (nm)"=w2344:dbl, "Treatment"=w2345:string, "Comments"=w2346:string)
                n1245 = local write "Rec: VT-Sat"(w2354) -> ()
                n1246 = local write "Date Created"(w2358) -> ()
                n1247 = local write "Rec: Material"(w2340) -> ()
                n1248 = local write "Rec: Solvent"(w2341) -> ()
                n1249 = local write "Rec: Concentration"(w2342) -> ()
                n1250 = local write "Rec: Method"(w2343) -> ()
                n1251 = local write "Rec: Dielectric (d)"(w2344) -> ()
                n1252 = local write "Surface Treatment:"(w2345) -> ()
                n1253 = local write "Comments"(w2346) -> ()
                n1254 = local write "Index"(w2348) -> ()
                n1255 = local write "Rec: Mobility-Sat"(w2351) -> ()
                n1256 = local write "Rec: Mobility-Lin"(w2352) -> ()
                n1257 = local write "Rec: On/Off"(w2353) -> ()
                n1258 = local write "Rec: STS"(w2355) -> ()
                n1259 = local write "Rec: Trap Density-VT"(w2356) -> ()
                n1260 = local write "Rec: Trap Density-STS"(w2357) -> ()
                n1261 = local write "Date Recorded"(w2347) -> ()
                n1262 = local write "Rec: Length"(w2349) -> ()
                n1263 = local write "Rec: Width"(w2350) -> ()
                n1264 = local write "Rec: Temp"(w2333) -> ()
                n1265 = Equal To 0?(x=w2333) -> (x = 0?=w2334:bool)
                n1266 = case shown="False" w2334 {
                  tunnel: [w2444 w2445] -> w2332
                  tunnel: w2333 -> [w2444 _]
                  frame False {
                  }
                  frame True {
                    n1267 = local read "Room Temp"() -> (w2445:dbl)
                  }
                }
                n1268 = local write "Data File"(w2336) -> ()
                n1269 = local read "NumPts 2"() -> (w2381:dbl)
                n1270 = local read "NumPts"() -> (w2370:dbl)
                n1271 = local read "NumPts"() -> (w2382:dbl)
                n1272 = call-poly <vilib>:"Read From Spreadsheet File.vi"("file path (dialog if empty)"=w2336) -> ("all rows"=w2430:string[][])  [unwired: 6 in, 4 out]
                n1273 = call "Mobility-Vt Calculator-File.vi"("NumPts"=w2382, "Path"=w2336) -> ("XY Graph-Sat"=w2383:cluster{dbl[], dbl[]}[], "XY Graph-Lin"=w2365:cluster{dbl[], dbl[]}[], "Output"=w2384:T8, "Index-Sat"=w2362:dbl, "Index-Lin"=w2369:dbl)  [unwired: 4 in, 1 out]
                n1274 = Decimate 1D Array(w2365) -> (w2377:cluster{dbl[], dbl[]}[])  [unwired: 1 out]
                n1275 = Array To Cluster(array=w2377) -> (cluster=w2375:T9)
                n1276 = Unbundle(w2375) -> ("[0]"=w2376:cluster{dbl[], dbl[]})  [unwired: 8 out]
                n1277 = local write "XY Graph-Lin"(w2365) -> ()
                n1278 = Unbundle(w2376) -> (w2374:dbl[], w2373:dbl[])
                n1279 = Array Subset(array=w2373, index=w2369, length=w2370) -> (w2371:dbl[])
                n1280 = Array Subset(array=w2374, index=w2369, length=w2370) -> (w2372:dbl[])
                n1281 = call "STS Calculator-File.vi"("NumPts"=w2381, "Path"=w2336) -> ("STS Index-Sat"=w2380:dbl, "XY Graph-Sat"=w2379:cluster{dbl[], dbl[]}[], "Ouput"=w2378:cluster{"STS-Sat":dbl, "STS-Lin":dbl})  [unwired: 5 in, 2 out]
                n1282 = local read "New: Dielectric"() -> (w2364:dbl)
                n1283 = local write "Lin Id-Used"(w2371) -> ()
                n1284 = local write "Lin-Vg Array-Used"(w2372) -> ()
                n1285 = local write "MobVi Index"(w2362) -> ()
                n1286 = local write "Slide"(w2362) -> ()
                n1287 = local write "XY Graph"(w2383) -> ()
                n1288 = local write "Index 2"(w2380) -> ()
                n1289 = local write "XY Graph 2"(w2379) -> ()
                n1290 = Unbundle By Name(w2384) -> ("Mobility-Sat"=w2368:dbl, "Vt-Sat"=w2361:dbl, "Mobility-Lin"=w2367:dbl, "Mobility-Lin"=w2366:dbl, "Off I-Sat"=w2359:dbl)
                n1291 = Array Size(array=w2430) -> (size(s)=w2429:i32[])
                n1292 = local write "Calc: Off I-Sat"(w2359) -> ()
                n1293 = Unbundle By Name(w2378) -> ("STS-Sat"=w2363:dbl)
                n1294 = call "Trap Density_STS.vi"("Temp (T) [K]"=w2332, "S.T.S. (S)"=w2363, "Dielectric"=w2364) -> ("Trap Density (N)"=w2335:dbl)  [unwired: 8 in]
                n1295 = local write "Calc: Mobility-Sat"(w2368) -> ()
                n1296 = local write "Calc: Mobility-Lin"(w2366) -> ()
                n1297 = local write "New: Trap Density-STS"(w2335) -> ()
                n1298 = local write "Calc: Trap Density-STS"(w2335) -> ()
                n1299 = local read "Image Folder"() -> (w2418:path)
                n1300 = local write "Calc: VT-Sat"(w2361) -> ()
                n1301 = local write "Calc: VT-Lin"(w2367) -> ()
                n1302 = local read "New: Dielectric"() -> (w2360:dbl)
                n1303 = Decimate 1D Array(w2383) -> (w2413:cluster{dbl[], dbl[]}[])  [unwired: 1 out]
                n1304 = Index Array(array=w2429, index=w2428) -> (element=w2409:i32)
                n1305 = Decimate 1D Array(w2379) -> (w2403:cluster{dbl[], dbl[]}[])  [unwired: 1 out]
                n1306 = Array Subset(array=w2430, index (row)=w2428, index (col)=w2428, length (col)=3) -> (w2431:string[][])  [unwired: 1 in]
                n1307 = local write "Calc: STS"(w2363) -> ()
                n1308 = List Folder(path=w2418) -> (filenames=w2423:string[])  [unwired: 3 in, 3 out]
                n1309 = local write "New: Mobility-Sat"(w2368) -> ()
                n1310 = Array To Cluster(array=w2413) -> (cluster=w2415:T9)
                n1311 = Array To Cluster(array=w2403) -> (cluster=w2401:T9)
                n1312 = Reshape Array(w2431, w2409) -> (w2416:string[])
                n1313 = local write "New: Mobility-Lin"(w2367) -> ()
                n1314 = Subtract(x=w2409, y=20) -> (x-y=w2408:i32)
                n1315 = local write "New: VT-Sat"(w2361) -> ()
                n1316 = local write "New: VT-Lin"(w2366) -> ()
                n1317 = local write "New: STS"(w2363) -> ()
                n1318 = property on="Slide" class="Slide (strict)"("Scale.Maximum"=w2408) -> ()  [unwired: 2 in, 2 out]
                n1319 = call "Trap Density_VT.vi"("VT"=w2361, "Dielectric"=w2360) -> ("Trap Density-VT"=w2331:dbl)
                n1320 = Unbundle(w2415) -> ("[0]"=w2414:cluster{dbl[], dbl[]})  [unwired: 8 out]
                n1321 = Unbundle(w2401) -> ("[0]"=w2402:cluster{dbl[], dbl[]})  [unwired: 8 out]
                n1322 = Search 1D Array(1D array=w2416, element="Index:") -> (index of element=w2425:i32)  [unwired: 1 in]
                n1323 = local write "New: Trap Density-VT"(w2331) -> ()
                n1324 = local write "Calc: Trap Density-VT"(w2331) -> ()
                n1325 = Increment(x=w2425) -> (x+1=w2426:i32)
                n1326 = Unbundle(w2414) -> (w2405:dbl[], w2404:dbl[])
                n1327 = Unbundle(w2402) -> (w2400:dbl[], w2399:dbl[])
                n1328 = Array Subset(array=w2405, index=w2362, length=w2382) -> (w2412:dbl[])
                n1329 = Array Subset(array=w2404, index=w2362, length=w2382) -> (w2411:dbl[])
                n1330 = Array Subset(array=w2400, index=w2380, length=w2381) -> (w2407:dbl[])
                n1331 = Array Subset(array=w2399, index=w2380, length=w2381) -> (w2406:dbl[])
                n1332 = Index Array(array=w2416, index=w2426) -> (element=w2421:string)
                n1333 = local write "Vg Array-Log-Used"(w2406) -> ()
                n1334 = local write "Sat Id-Log-Used"(w2407) -> ()
                n1335 = local write "Sat Id-Used"(w2411) -> ()
                n1336 = local write "Index"(w2421) -> ()
                n1337 = local write "Sat Vg Array-Used"(w2412) -> ()
                n1338 = while {
                  tunnel: w2423 -> [w2453]
                  tunnel: w2421 -> [w2451]
                  tunnel: [w2450] -> _
                  tunnel: [w2450] -> w2422
                  tunnel: w2409 -> [w2449]
                  i -> [w2450]
                  stop <- w2446 stop-if-true
                  n1339 = Index Array(array=w2453, index=w2450) -> (element=w2454:string)
                  n1340 = xnode "Match Regular Expression"("input string"=w2454, "regular expression"=w2451) -> ("whole match"=w2452:string)  [unwired: 4 in, 4 out]
                  n1341 = Equal?(x=w2452, y=w2451) -> (x = y?=w2448:bool)
                  n1342 = Equal?(x=w2449, y=w2450) -> (x = y?=w2447:bool)
                  n1343 = Or(x=w2448, y=w2447) -> (x .or. y?=w2446:bool)
                }
                n1344 = Path To String(path=w2418) -> (string=w2420:string)
                n1345 = Index Array(array=w2423, index=w2422) -> (element=w2397:string)
                n1346 = local write "Image Name"(w2397) -> ()
                n1347 = Empty String/Path?(string/path=w2397) -> (empty?=w2398:bool)
                n1348 = Concatenate Strings(w2420, "\\", w2397) -> (w2419:string)
                n1349 = String To Path(string=w2419) -> (path=w2396:path)
                n1350 = local read "No Image"() -> (w2395:path)
                n1351 = Select(t=w2395, s=w2398, f=w2396) -> (s? t:f=w2389:path)
                n1352 = local write "Image File"(w2389) -> ()
                n1353 = local read "Image Out"() -> (w2387:T2)
                n1354 = call "IMAQ ReadFile"("File Path"=w2389, "Image"=w2387) -> ("Image Out"=w2388:T2)  [unwired: 5 in, 4 out]
                n1355 = local write "Image Out"(w2388) -> ()
                n1356 = local write "Image Out 2"(w2388) -> ()
              }
              frame #4 {
                # "Output ROI data"
                n1357 = local read "Image Folder"() -> (w2569:path)
                n1358 = Build Path(base path=w2569, name or relative path="ROI") -> (appended path=w2571:path)
                n1359 = local read "Index"() -> (w2570:string)
                n1360 = Build Path(base path=w2571, name or relative path=w2570) -> (appended path=w2576:path)
                n1361 = invoke on="Image Out" class="ImageControl" method="Clear ROI"() -> (error out=w2575:errorcluster)  [unwired: 3 in, 2 out]
                n1362 = call <vilib>:"Check if File or Folder Exists.vi"("error in (no error)"=w2575, "path"=w2576) -> ("file or folder exists?"=w2573:bool, "dup path"=w2574:path)  [unwired: 7 in, 1 out]
                n1363 = case shown="True" w2573 {
                  tunnel: w2574 -> [_ w2577]
                  frame False {
                  }
                  frame True {
                    n1364 = Read from Text File(file (use dialog)=w2577) -> (text=w2581:string)  [unwired: 3 in, 3 out]
                    n1365 = property on="Image Out" class="ImageControl"() -> ("ROI"=w2578:T10)  [unwired: 2 in, 2 out]
                    n1366 = Unflatten From String(type=w2578, binary string=w2581) -> (value=w2579:T10, error out=w2580:errorcluster)  [unwired: 3 in, 1 out]
                    n1367 = property on="Image Out" class="ImageControl"(error in=w2580, "ROI"=w2579) -> ()  [unwired: 1 in, 2 out]
                  }
                }
              }
            }
            n1368 = flat-sequence {
              tunnel: [w2043] -> w2030
              tunnel: w2030 -> [w2057]
              frame #0 {
                # "Makes Empty File for Transformer Data"
                n1369 = local read "Data Folder"() -> (w2032:path)
                n1370 = Build Path(base path=w2032, name or relative path="Stats") -> (appended path=w2034:path)
                n1371 = call <vilib>:"Check if File or Folder Exists.vi"("path"=w2034) -> ("file or folder exists?"=w2035:bool, "dup path"=w2036:path)  [unwired: 8 in, 1 out]
                n1372 = case shown="False" w2035 {
                  tunnel: [w2040 w2042] -> w2037
                  tunnel: w2036 -> [w2041 w2042]
                  frame False {
                    n1373 = Create Folder(path (use dialog)=w2041) -> (created path=w2040:path)  [unwired: 2 in, 2 out]
                  }
                  frame True {
                  }
                }
                n1374 = Build Path(base path=w2037, name or relative path="Tranformer Data.txt") -> (appended path=w2039:path)
                n1375 = call-poly <vilib>:"Write To Spreadsheet File.vi"("append to file? (new file:F)"=TRUE, "file path (dialog if empty)"=w2039) -> ()  [unwired: 6 in, 1 out]
              }
              frame #1 {
                # "Adds Headers if they don't exist"
                n1376 = Concatenate Strings("Stats\\", "Tranformer Data.txt") -> (w2050:string)
                n1377 = local read "Data Folder"() -> (w2049:path)
                n1378 = Build Path(base path=w2049, name or relative path=w2050) -> (appended path=w2043:path)
                n1379 = call-poly <vilib>:"Read From Spreadsheet File.vi"("file path (dialog if empty)"=w2043) -> ("first row"=w2048:string[])  [unwired: 6 in, 4 out]
                n1380 = Search 1D Array(1D array=w2048, element="DeviceID") -> (index of element=w2046:i32)  [unwired: 1 in]
                n1381 = Equal?(x=w2046, y=0) -> (x = y?=w2044:bool)
                n1382 = case shown="False" w2044 {
                  tunnel: w2043 -> [w2054 _]
                  frame False {
                    n1383 = local read "Transformer \nHeaders"() -> (w2053:string[])
                    n1384 = call-poly <vilib>:"Write To Spreadsheet File.vi"("1D data"=w2053, "file path (dialog if empty)"=w2054) -> ()  [unwired: 6 in, 1 out]
                  }
                  frame True {
                  }
                }
              }
              frame #2 {
                # "Adds current device if it doesn't exist"
                n1385 = local read "Current \nRecord"() -> (w2060:string[])
                n1386 = Index Array(array=w2060, index=0) -> (element=w2059:string)
                n1387 = Concatenate Strings("Stats\\", "Tranformer Data.txt") -> (w2063:string)
                n1388 = local read "Data Folder"() -> (w2062:path)
                n1389 = local write "Current Device ID"(w2059) -> ()
                n1390 = local read "Current Device ID"() -> (w2069:string)
                n1391 = Build Path(base path=w2062, name or relative path=w2063) -> (appended path=w2061:path)
                n1392 = call-poly <vilib>:"Read From Spreadsheet File.vi"("file path (dialog if empty)"=w2061) -> ("all rows"=w2056:string[][])  [unwired: 6 in, 4 out]
                n1393 = Index Array(array=w2056, index (col)=0) -> (element=w2067:string[])  [unwired: 1 in]
                n1394 = Search 1D Array(1D array=w2067, element=w2069) -> (index of element=w2055:i32)  [unwired: 1 in]
                n1395 = Equal?(x=w2055, y=-1) -> (x = y?=w2058:bool)
                n1396 = case shown="False" w2058 {
                  tunnel: w2057 -> [w2071 w2084]
                  tunnel: w2055 -> [w2076 _]
                  tunnel: w2056 -> [w2077 _]
                  frame False {
                    n1397 = local read "Current \nRecord"() -> (w2075:string[])
                    n1398 = Replace Array Subset(array=w2077, new element=w2075, index (row)=w2076) -> (w2072:string[][])  [unwired: 1 in]
                    n1399 = flat-sequence {
                      tunnel: [w2078] -> _
                      tunnel: [w2079] -> _
                      tunnel: [w2079] -> w2074
                      tunnel: [w2078] -> w2073
                      tunnel: w2072 -> [w2079]
                      tunnel: w2071 -> [w2078]
                      tunnel: w2074 -> [w2081]
                      tunnel: w2073 -> [w2080]
                      frame #0 {
                        n1400 = Delete(path (use dialog)=w2078) -> ()  [unwired: 4 in, 3 out]
                      }
                      frame #1 {
                        n1401 = call-poly <vilib>:"Write To Spreadsheet File.vi"("append to file? (new file:F)"=TRUE, "2D data"=w2081, "file path (dialog if empty)"=w2080) -> ()  [unwired: 5 in, 1 out]
                      }
                    }
                  }
                  frame True {
                    n1402 = local read "Current \nRecord"() -> (w2083:string[])
                    n1403 = call-poly <vilib>:"Write To Spreadsheet File.vi"("append to file? (new file:F)"=TRUE, "1D data"=w2083, "file path (dialog if empty)"=w2084) -> ()  [unwired: 5 in, 1 out]
                  }
                }
              }
            }
          }
          event "Export": Mouse Down {
            n1404 = event-data() -> ()  [unwired: 1 in, 7 out]
            n1405 = local read "Data Folder"() -> (w2585:path)
            n1406 = Build Path(base path=w2585, name or relative path="Stats") -> (appended path=w2586:path)
            n1407 = call <vilib>:"Check if File or Folder Exists.vi"("path"=w2586) -> ("file or folder exists?"=w2602:bool, "dup path"=w2601:path)  [unwired: 8 in, 1 out]
            n1408 = local read "Project"() -> (w2598:path)
            n1409 = call <userlib>:"OA_ConnectToOrigin.vi"() -> ("error out"=w2599:errorcluster, "Origin.IOApplication"=w2600:refnum<k7>)  [unwired: 8 in]
            n1410 = case shown="False" w2602 {
              tunnel: w2601 -> [w2711 w2712]
              tunnel: [w2710 w2712] -> w2584
              frame False {
                n1411 = Create Folder(path (use dialog)=w2711) -> (created path=w2710:path)  [unwired: 2 in, 2 out]
              }
              frame True {
              }
            }
            n1412 = call <userlib>:"OA_Load.vi"("error in (no error)"=w2599, "Path"=w2598, "Origin.IOApplication"=w2600) -> ("error out"=w2596:errorcluster, "Origin.IOApplication"=w2597:refnum<k7>)  [unwired: 1 out]
            n1413 = call <userlib>:"OAExecute.vi"("script"="document -m 3;", "Error IO"=w2596, "Origin.IOApplication"=w2597) -> ("Error IO Out"=w2594:errorcluster, "Origin.IOApplication"=w2595:refnum<k7>)  [unwired: 1 in, 1 out]
            n1414 = stacked-sequence {
              tunnel: w2585 -> [w2614 w2617 w2630 w2643 w2656 w2669 w2683 w2697]
              tunnel: w2584 -> [w2613 w2618 w2631 w2644 w2657 w2670 w2682 w2698]
              tunnel: w2595 -> [w2610 w2620 w2633 w2646 w2659 w2672 w2685 w2700]
              tunnel: w2594 -> [w2612 w2619 w2632 w2645 w2658 w2671 w2684 w2699]
              tunnel: [_ _ _ _ _ _ _ w2695] -> w2583
              tunnel: [_ _ _ _ _ _ _ w2696] -> w2582
              frame #0 {
                n1415 = call "Param_Analysis_7_24b_JW.vi"("error in (no error)"=w2612, "Data Folder"=w2614, "Parameter String"="Mobility-Sat (cm^2/Vs):", "Parameter Name"="Mobility-Sat", "Stats Folder"=w2613) -> ("error out"=w2606:errorcluster, "Output Array"=w2604:string[][])  [unwired: 4 in, 1 out]
                n1416 = call "Origin_Export_7_24a_JW.vi"("Analysis Array"=w2604, "error in (no error)"=w2606, "Parameter Worksheet Name"="[MOBSvsLTable]Mobilities", "Parameter Folder Script"="pe_cd \"Mobility-Sat\";", "Origin.IOApplication"=w2610) -> ("error out"=w2605:errorcluster, "reference out"=w2607:refnum<k7>)  [unwired: 4 in, 1 out]
                n1417 = call <userlib>:"OAExecute.vi"("script"="window -a MOBSvsLTable;\nwindow -s TV;", "Error IO"=w2605, "Origin.IOApplication"=w2607) -> ()  [unwired: 1 in, 3 out]
              }
              frame #1 {
                n1418 = call "Param_Analysis_7_24b_JW.vi"("error in (no error)"=w2619, "Data Folder"=w2617, "Parameter String"="Mobility-Lin (cm^2/Vs):", "Parameter Name"="Mobility-Lin", "Stats Folder"=w2618) -> ("error out"=w2622:errorcluster, "Output Array"=w2624:string[][])  [unwired: 4 in, 1 out]
                n1419 = call "Origin_Export_7_24a_JW.vi"("Analysis Array"=w2624, "error in (no error)"=w2622, "Parameter Worksheet Name"="[MOBLvsLTable]Mobilities", "Parameter Folder Script"="pe_cd \"Mobility-Lin\";", "Origin.IOApplication"=w2620) -> ("error out"=w2621:errorcluster, "reference out"=w2623:refnum<k7>)  [unwired: 4 in, 1 out]
                n1420 = call <userlib>:"OAExecute.vi"("script"="window -a MOBLvsLTable;\nwindow -s TV;", "Error IO"=w2621, "Origin.IOApplication"=w2623) -> ()  [unwired: 1 in, 3 out]
              }
              frame #2 {
                n1421 = call "Param_Analysis_7_24b_JW.vi"("error in (no error)"=w2632, "Data Folder"=w2630, "Parameter String"="Off I-Sat (A):", "Parameter Name"="Off I-Sat", "Stats Folder"=w2631) -> ("error out"=w2636:errorcluster, "Output Array"=w2634:string[][])  [unwired: 4 in, 1 out]
                n1422 = call "Origin_Export_7_24a_JW.vi"("Analysis Array"=w2634, "error in (no error)"=w2636, "Parameter Worksheet Name"="[OffItable]OffCurrents", "Parameter Folder Script"="pe_cd \"Off I-Sat\";", "Origin.IOApplication"=w2633) -> ("error out"=w2635:errorcluster, "reference out"=w2637:refnum<k7>)  [unwired: 4 in, 1 out]
                n1423 = call <userlib>:"OAExecute.vi"("script"="window -a OffItable;\nwindow -s TV;", "Error IO"=w2635, "Origin.IOApplication"=w2637) -> ()  [unwired: 1 in, 3 out]
              }
              frame #3 {
                n1424 = call "Param_Analysis_7_24b_JW.vi"("error in (no error)"=w2645, "Data Folder"=w2643, "Parameter String"="On/Off I-Sat:", "Parameter Name"="OnOff Ratio", "Stats Folder"=w2644) -> ("error out"=w2649:errorcluster, "Output Array"=w2647:string[][])  [unwired: 4 in, 1 out]
                n1425 = call "Origin_Export_7_24a_JW.vi"("Analysis Array"=w2647, "error in (no error)"=w2649, "Parameter Worksheet Name"="[OnOffTable]On/Off Ratios", "Parameter Folder Script"="pe_cd \"On Off Ratio\";", "Origin.IOApplication"=w2646) -> ("error out"=w2648:errorcluster, "reference out"=w2650:refnum<k7>)  [unwired: 4 in, 1 out]
                n1426 = call <userlib>:"OAExecute.vi"("script"="window -a OnOffTable;\nwindow -s TV;", "Error IO"=w2648, "Origin.IOApplication"=w2650) -> ()  [unwired: 1 in, 3 out]
              }
              frame #4 {
                n1427 = call "Param_Analysis_7_24b_JW.vi"("error in (no error)"=w2658, "Data Folder"=w2656, "Parameter String"="STS-Sat (V/decade):", "Parameter Name"="STS-Sat", "Stats Folder"=w2657) -> ("error out"=w2662:errorcluster, "Output Array"=w2660:string[][])  [unwired: 4 in, 1 out]
                n1428 = call "Origin_Export_7_24a_JW.vi"("Analysis Array"=w2660, "error in (no error)"=w2662, "Parameter Worksheet Name"="[STable]Threshold Swing", "Parameter Folder Script"="pe_cd \"STS-Sat\";", "Origin.IOApplication"=w2659) -> ("error out"=w2661:errorcluster, "reference out"=w2663:refnum<k7>)  [unwired: 4 in, 1 out]
                n1429 = call <userlib>:"OAExecute.vi"("script"="window -a STable;\nwindow -s TV;", "Error IO"=w2661, "Origin.IOApplication"=w2663) -> ()  [unwired: 1 in, 3 out]
              }
              frame #5 {
                n1430 = call "Param_Analysis_7_24b_JW.vi"("error in (no error)"=w2671, "Data Folder"=w2669, "Parameter String"="Trap Density-STS (Traps/Vcm^2):", "Parameter Name"="Trap Density-STS", "Stats Folder"=w2670) -> ("error out"=w2675:errorcluster, "Output Array"=w2673:string[][])  [unwired: 4 in, 1 out]
                n1431 = call "Origin_Export_7_24a_JW.vi"("Analysis Array"=w2673, "error in (no error)"=w2675, "Parameter Worksheet Name"="[NSTSTable]Trap Densities", "Parameter Folder Script"="pe_cd \"Trap Density-STS\";", "Origin.IOApplication"=w2672) -> ("error out"=w2674:errorcluster, "reference out"=w2676:refnum<k7>)  [unwired: 4 in, 1 out]
                n1432 = call <userlib>:"OAExecute.vi"("script"="window -a NSTSTable;\nwindow -s TV;", "Error IO"=w2674, "Origin.IOApplication"=w2676) -> ()  [unwired: 1 in, 3 out]
              }
              frame #6 {
                n1433 = call "Param_Analysis_7_24b_JW.vi"("error in (no error)"=w2684, "Data Folder"=w2683, "Parameter String"="Trap Density-Vt (Traps/Vcm^2):", "Parameter Name"="Trap Density-Vt", "Stats Folder"=w2682) -> ("error out"=w2688:errorcluster, "Output Array"=w2686:string[][])  [unwired: 4 in, 1 out]
                n1434 = call "Origin_Export_7_24a_JW.vi"("Analysis Array"=w2686, "error in (no error)"=w2688, "Parameter Worksheet Name"="[NVTTable]Trap Densities", "Parameter Folder Script"="pe_cd \"Trap Density-Vt\";", "Origin.IOApplication"=w2685) -> ("error out"=w2687:errorcluster, "reference out"=w2689:refnum<k7>)  [unwired: 4 in, 1 out]
                n1435 = call <userlib>:"OAExecute.vi"("script"="window -a NVTTable;\nwindow -s TV;", "Error IO"=w2687, "Origin.IOApplication"=w2689) -> ()  [unwired: 1 in, 3 out]
              }
              frame #7 {
                n1436 = call "Param_Analysis_7_24b_JW.vi"("error in (no error)"=w2699, "Data Folder"=w2697, "Parameter String"="Vt-Sat (V):", "Parameter Name"="Vt-Sat", "Stats Folder"=w2698) -> ("error out"=w2703:errorcluster, "Output Array"=w2701:string[][])  [unwired: 4 in, 1 out]
                n1437 = call "Origin_Export_7_24a_JW.vi"("Analysis Array"=w2701, "error in (no error)"=w2703, "Parameter Worksheet Name"="[VtTable]Threshold Voltages", "Parameter Folder Script"="pe_cd \"Vt-Sat\";", "Origin.IOApplication"=w2700) -> ("error out"=w2702:errorcluster, "reference out"=w2704:refnum<k7>)  [unwired: 4 in, 1 out]
                n1438 = call <userlib>:"OAExecute.vi"("script"="window -a VtTable;\nwindow -s TV;", "Error IO"=w2702, "Origin.IOApplication"=w2704) -> ("Error IO Out"=w2695:errorcluster, "Origin.IOApplication"=w2696:refnum<k7>)  [unwired: 1 in, 1 out]
              }
            }
            n1439 = call "File Dialog"("start path"=w2586) -> ("selected path"=w2589:path)  [unwired: 11 in, 3 out]
            n1440 = Path To String(path=w2589) -> (string=w2588:string)
            n1441 = call <userlib>:"OAExecute.vi"("script"="pe_cd /; ", "Error IO"=w2583, "Origin.IOApplication"=w2582) -> ("Error IO Out"=w2590:errorcluster, "Origin.IOApplication"=w2591:refnum<k7>)  [unwired: 1 in, 1 out]
            n1442 = call <userlib>:"OASaveProject.vi"("path"=w2588, "Error IO"=w2590, "Origin.IOApplication"=w2591) -> ()  [unwired: 3 out]
          }
          event "Blank Button": Mouse Down {
            n1443 = event-data() -> ()  [unwired: 1 in, 7 out]
            n1444 = local read "Data File"() -> (w2720:path)
            n1445 = Strip Path(path=w2720) -> (stripped path=w2716:path, name=w2718:string)
            n1446 = Path To String(path=w2716) -> (string=w2715:string)
            n1447 = Concatenate Strings(w2715, "\\", "X_", w2718) -> (w2714:string)
            n1448 = String To Path(string=w2714) -> (path=w2713:path)
            n1449 = Move(source path=w2720, 10:w2713) -> ()  [unwired: 3 in, 3 out]
            n1450 = local write "Data File"(w2713) -> ()
          }
          event "Cancel Button": Mouse Down {
            (unwired) 6
            n1451 = event-data() -> ()  [unwired: 1 in, 7 out]
            n1452 = call "Simulate_Keyboard.vi"("Action"=2, "Virtual Key"=162) -> ()  [unwired: 7 in, 1 out]
          }
        }
        n1453 = Multiply(x=w517, y=10) -> (x*y=w519:sgl)
        n1454 = case shown="\"0\"" w558 {
          tunnel: w532 -> [w611 w617 w621 w623 w627 w629 w631 w633 w635 w637 w639 w641 w643 w645 w647 w649 w651 w653 w655 w657 w659 w661 w663 w665 w667 w669 w671 w673 w675 w677 w679 w681 w683 w685 w687 w689 w691 w693 w695 w697 w699 w701 w703 w705 w707 w709 w711 w713 w715 w717 w719 w721 w723 w725 w727 w729 w731 w733 w735 w737 w739 w741 w743 w745 w747 w749 w751 w753 w755 w757 w759 w761 w763 w765 w767 w769 w771 w773 w775 w777 w779 w781 w783 w785 w787 w789 w791 w793 w795 w797 w799 w801 w803 w805 w807 w809 w811 w813 w815 w817 w819 w821 w823 w825 w827]
          tunnel: [w611 w616 w620 w623 w627 w629 w631 w633 w635 w637 w639 w641 w643 w645 w647 w649 w651 w653 w655 w657 w659 w661 w663 w665 w667 w669 w671 w673 w675 w677 w679 w681 w683 w685 w687 w689 w691 w693 w695 w697 w699 w701 w703 w705 w707 w709 w711 w713 w715 w717 w719 w721 w723 w725 w727 w729 w731 w733 w735 w737 w739 w741 w743 w745 w747 w749 w751 w753 w755 w757 w759 w761 w763 w765 w767 w769 w771 w773 w775 w777 w779 w781 w783 w785 w787 w789 w791 w793 w795 w797 w799 w801 w803 w805 w807 w809 w811 w813 w815 w817 w819 w821 w823 w825 w827] -> w557
          tunnel: w533 -> [w613 w615 w619 w625 w626 w628 w630 w632 w634 w636 w638 w640 w642 w644 w646 w648 w650 w652 w654 w656 w658 w660 w662 w664 w666 w668 w670 w672 w674 w676 w678 w680 w682 w684 w686 w688 w690 w692 w694 w696 w698 w700 w702 w704 w706 w708 w710 w712 w714 w716 w718 w720 w722 w724 w726 w728 w730 w732 w734 w736 w738 w740 w742 w744 w746 w748 w750 w752 w754 w756 w758 w760 w762 w764 w766 w768 w770 w772 w774 w776 w778 w780 w782 w784 w786 w788 w790 w792 w794 w796 w798 w800 w802 w804 w806 w808 w810 w812 w814 w816 w818 w820 w822 w824 w826]
          tunnel: [w612 w615 w619 w624 w626 w628 w630 w632 w634 w636 w638 w640 w642 w644 w646 w648 w650 w652 w654 w656 w658 w660 w662 w664 w666 w668 w670 w672 w674 w676 w678 w680 w682 w684 w686 w688 w690 w692 w694 w696 w698 w700 w702 w704 w706 w708 w710 w712 w714 w716 w718 w720 w722 w724 w726 w728 w730 w732 w734 w736 w738 w740 w742 w744 w746 w748 w750 w752 w754 w756 w758 w760 w762 w764 w766 w768 w770 w772 w774 w776 w778 w780 w782 w784 w786 w788 w790 w792 w794 w796 w798 w800 w802 w804 w806 w808 w810 w812 w814 w816 w818 w820 w822 w824 w826] -> w556
          tunnel: w519 -> [w610 w614 w618 w622 _ _ _ _ _ _ _ _ _ _ _ _ _ _ _ _ _ _ _ _ _ _ _ _ _ _ _ _ _ _ _ _ _ _ _ _ _ _ _ _ _ _ _ _ _ _ _ _ _ _ _ _ _ _ _ _ _ _ _ _ _ _ _ _ _ _ _ _ _ _ _ _ _ _ _ _ _ _ _ _ _ _ _ _ _ _ _ _ _ _ _ _ _ _ _ _ _ _ _ _ _]
          frame "DOWN" {
            n1455 = Add(x=w613, y=w610) -> (x+y=w612:sgl)
          }
          frame "LEFT" {
            n1456 = Subtract(x=w617, y=w614) -> (x-y=w616:sgl)
          }
          frame "RIGHT" {
            n1457 = Add(x=w621, y=w618) -> (x+y=w620:sgl)
          }
          frame "UP" {
            n1458 = Subtract(x=w625, y=w622) -> (x-y=w624:sgl)
          }
          frame "ENTER (num pad)" {
          }
          frame "' (quote)" {
          }
          frame "END" {
          }
          frame "EQUALS" {
          }
          frame "ESCAPE" {
          }
          frame "GRAVE (`)" {
          }
          frame "HOME" {
          }
          frame "INSERT" {
          }
          frame "LBRACKET" {
          }
          frame "LCONTROL" {
          }
          frame "L ALT" {
          }
          frame "LSHIFT" {
          }
          frame "LWIN" {
          }
          frame "MINUS" {
          }
          frame "MULTIPLY" {
          }
          frame "NEXT" {
          }
          frame "NUMLOCK" {
          }
          frame "NUMPAD_0" {
          }
          frame "NUMPAD_1" {
          }
          frame "NUMPAD_2" {
          }
          frame "NUMPAD_3" {
          }
          frame "NUMPAD_4" {
          }
          frame "NUMPAD_5" {
          }
          frame "NUMPAD_6" {
          }
          frame "NUMPAD_7" {
          }
          frame "NUMPAD_8" {
          }
          frame "NUMPAD_9" {
          }
          frame "PAUSE" {
          }
          frame "PERIOD" {
          }
          frame "PRIOR (PG UP)" {
          }
          frame "RBRACKET" {
          }
          frame "RCONTROL" {
          }
          frame "RETURN" {
          }
          frame "R ALT" {
          }
          frame "RSHIFT" {
          }
          frame "RWIN" {
          }
          frame "SCROLL" {
          }
          frame "SEMICOLON" {
          }
          frame "SLASH" {
          }
          frame "SPACE" {
          }
          frame "SUBTRACT" {
          }
          frame "TAB" {
          }
          frame "DIVIDE" {
          }
          frame "DELETE" {
          }
          frame "DECIMAL" {
          }
          frame "COMMA" {
          }
          frame "CAPITAL" {
          }
          frame "BACKSLASH" {
          }
          frame "BACK" {
          }
          frame "ADD" {
          }
          frame "F15" {
          }
          frame "F14" {
          }
          frame "F13" {
          }
          frame "F12" {
          }
          frame "F11" {
          }
          frame "F10" {
          }
          frame "F9" {
          }
          frame "F8" {
          }
          frame "F7" {
          }
          frame "F6" {
          }
          frame "F5" {
          }
          frame "F4" {
          }
          frame "F3" {
          }
          frame "F2" {
          }
          frame "F1" {
          }
          frame "Z" {
          }
          frame "Y" {
          }
          frame "X" {
          }
          frame "W" {
          }
          frame "V" {
          }
          frame "U" {
          }
          frame "T" {
          }
          frame "S" {
          }
          frame "R" {
          }
          frame "Q" {
          }
          frame "P" {
          }
          frame "O" {
          }
          frame "N" {
          }
          frame "M" {
          }
          frame "L" {
          }
          frame "K" {
          }
          frame "J" {
          }
          frame "I" {
          }
          frame "H" {
          }
          frame "G" {
          }
          frame "F" {
          }
          frame "E" {
          }
          frame "D" {
          }
          frame "C" {
          }
          frame "B" {
          }
          frame "A" {
          }
          frame "9" {
          }
          frame "8" {
          }
          frame "7" {
          }
          frame "6" {
          }
          frame "5" {
          }
          frame "4" {
          }
          frame "3" {
          }
          frame "2" {
          }
          frame "1" {
          }
          frame "0" {
          }
        }
        n1459 = Bundle(w535, w534, w549, w548, 0.0) -> (w547:cluster{dbl, dbl, dbl, dbl, dbl})  [unwired: 1 in]
        n1460 = Bundle("X"=w557, "Y"=w556) -> (w551:cluster{"X":sgl, "Y":sgl})  [unwired: 1 in]
        n1461 = Divide(x=20, y=w518) -> (x/y=w521:sgl)
        n1462 = property on="Image Out" class="ImageControl"("Image Center Position"=w551) -> ()  [unwired: 2 in, 2 out]
        n1463 = call "IMAQ Convert Rectangle to ROI (Polygon)"("Rectangle"=w547) -> ("ROI Descriptor"=w545:T3)  [unwired: 7 in, 2 out]
        n1464 = Bundle("Application Font", w521, w525, w525, w525, w525, w525, TRUE, w523) -> (w527:T16)  [unwired: 1 in]
        n1465 = property on="Image Out 2" class="ImageControl"("ROI"=w545) -> ()  [unwired: 2 in, 2 out]
        n1466 = Bundle(w523, w527, w523, w523) -> (w526:T17)  [unwired: 1 in]
        n1467 = property on="Image Out" class="ImageControl"() -> ("ROI"=w510:T10)  [unwired: 2 in, 2 out]
        n1468 = Unbundle By Name(w510) -> ("Contours"=w574:T14)
        n1469 = local read "Image Out"() -> (w529:T2)
        n1470 = call "IMAQ Clear Overlay"("Image"=w529) -> ("Image Out"=w528:T2)  [unwired: 9 in, 1 out]
        n1471 = Initialize Array(0) -> (w572:i32[])  [unwired: 1 in]
        n1472 = local read "Magnification"() -> (w563:u16)
        n1473 = Array Size(array=w574) -> (size(s)=w573:i32)
        n1474 = Build Array(0.505025, 0.252522, 0.127742, 0.050345, 0.031129) -> (w564:dbl[])
        n1475 = Array Subset(array=w564, index=w563, length=1) -> (w561:dbl[])
        n1476 = property on="Image Out" class="ImageControl"() -> ("ZoomInteger"=w553:cluster{"X":i32, "Y":i32})  [unwired: 2 in, 2 out]
        n1477 = To Double Precision Float(number=w561) -> (double precision float=w560:dbl[])
        n1478 = for {
          N: w573 -> [_]
          shift-right: [w850] -> _
          shift-left: w574 -> [w850]
          shift-right: [w848] -> w559
          shift-left: w572 -> [w847]
          tunnel: w560 -> [w846]
          shift-right: [w843] -> _
          shift-left: w528 -> [w845]
          tunnel: w526 -> [w838]
          i -> [w842]
          n1479 = Index Array(array=w850, index=w842) -> (element=w859:T18)
          n1480 = Unbundle(w859) -> ("Points"=w858:i32[])  [unwired: 2 out]
          n1481 = Array To Cluster(array=w858) -> (cluster=w857:T19)
          n1482 = Unbundle(w857) -> ("Points[0]"=w837:i32, "Points[1]"=w834:i32, "Points[2]"=w849:i32, "Points[3]"=w855:i32)  [unwired: 5 out]
          n1483 = Add(x=w837, y=10) -> (x+y=w835:i32)
          n1484 = Subtract(x=w834, y=w855) -> (x-y=w854:i32)
          n1485 = Subtract(x=w837, y=w849) -> (x-y=w856:i32)
          n1486 = Square(x=w854) -> (x^2=w852:i32)
          n1487 = Square(x=w856) -> (x^2=w853:i32)
          n1488 = Add(x=w853, y=w852) -> (x+y=w851:i32)
          n1489 = Square Root(x=w851) -> (sqrt(x)=w828:dbl)
          n1490 = Multiply(x=w828, y=0.5) -> (x*y=w831:dbl)
          n1491 = Add(x=w831, y=w834) -> (x+y=w833:dbl)
          n1492 = Bundle(w835, w833) -> (w844:cluster{i32, dbl})  [unwired: 1 in]
          n1493 = Multiply(x=w828, y=w846) -> (x*y=w841:dbl[])
          n1494 = Index Array(array=w841) -> (element=w840:dbl)  [unwired: 1 in]
          n1495 = Number To Fractional String(number=w840) -> (F-format string=w839:string)  [unwired: 3 in]
          n1496 = call "IMAQ Overlay Text"("BG Color (Transparent)"=u32 0, "Text Color (black)"=u32 16448250, "Font, Size & Style"=w838, "String"=w839, "Origin"=w844, "Image"=w845) -> ("Image Out"=w843:T2)  [unwired: 4 in, 1 out]
          n1497 = Build Array (concatenate)(w847, w841) -> (w848:dbl[])
          n1498 = local write "Numeric 3"(w828) -> ()
        }
        n1499 = local write "ROI Descriptor"(w510) -> ()
        n1500 = Unbundle(w553) -> ("X"=w552:i32)  [unwired: 1 out]
        n1501 = Add Array Elements(numeric array=w559) -> (sum=w570:dbl)
        n1502 = local write "Distances"(w559) -> ()
        n1503 = local write "Total Width"(w570) -> ()
        n1504 = local write "Zoom"(w552) -> ()
        n1505 = local read "Manual-Width"() -> (w509:bool)
        n1506 = local read "Total Width"() -> (w513:dbl)
        n1507 = local read "Rec: Width"() -> (w511:dbl)
        n1508 = Not(x=w509) -> (.not. x?=w507:bool)
        n1509 = Equal To 0?(x=w513) -> (x = 0?=w508:bool)
        n1510 = Or(x=w508, y=w509) -> (x .or. y?=w512:bool)
        n1511 = And(x=w508, y=w507) -> (x .and. y?=w506:bool)
        n1512 = case shown="True" w506 {
          tunnel: w511 -> [_ w588]
          frame False {
          }
          frame True {
            n1513 = local write "New: Width"(w588) -> ()
          }
        }
        n1514 = case shown="False" w512 {
          tunnel: w513 -> [w589 _]
          frame False {
            n1515 = local write "New: Width"(w589) -> ()
          }
          frame True {
          }
        }
        n1516 = local read "Manuel-Dielectric"() -> (w435:bool)
        n1517 = local read "Rec: Dielectric (d)"() -> (w434:dbl)
        n1518 = local read "Manuel-Length"() -> (w436:bool)
        n1519 = local read "Rec: Length"() -> (w437:dbl)
        n1520 = case shown="False" w436 {
          tunnel: w437 -> [w579 _]
          frame False {
            n1521 = local write "New: Length"(w579) -> ()
          }
          frame True {
          }
        }
        n1522 = case shown="False" w435 {
          tunnel: w434 -> [w578 _]
          frame False {
            n1523 = local write "New: Dielectric"(w578) -> ()
          }
          frame True {
          }
        }
      }
    }
  }
  n1524 = Build Array("DeviceID", "Fabricator", "Deposition", "Date", "Sample", "Row", "Column", "L (um)", "W (um)", "Material", "Treatment", "TC (mM)", "Solvent", "C (%)", "ST (C)", "Drops", "Wait (s)", "RT (F)", "RH (%)", "Ramp (s)", "RPM", "Accel (RPM/s)", "Time (s)", "Mobility", "On/Off", "Vt", "S.T.S") -> (→"Transformer \nHeaders":string[])
